vi "CRYO_MASTER_FULL_CHF2023.vi"() -> ()   [LabVIEW 2020]
uses:
  LSI218Data.lvclass
  LSI336Data.lvclass
  USBData.lvclass
  6240AData.lvclass
  DMMsData.lvclass
  LMData.lvclass
  <vilib>/DAQmx/miscellaneous.llb/DAQmx Fill In Error Info.vi
  <vilib>/DAQmx/create/channels.llb/DAQmx Create Channel (DO-Digital Output).vi
  <vilib>/DAQmx/create/channels.llb/DAQmx Create Channel (AO-Voltage-Basic).vi
  <vilib>/express/express arith-compare/Formula/XNode/ExpressFormulaBlockNode.xnode
  <vilib>/Analysis/NI_AALBase.lvlib
  istr.lib/Agilent 33XXX Series/Agilent 33XXX Series.lvlib
panel:
  out "Error Out (AZDAX status)":errorcluster
  in  "Automatic \nScreenshots?":bool=TRUE
  in  "Frontpanel screenshots":bool
  in  "Screenshots interval":i64=3605
  in  "Record interval":i64=1
  out "Cycle #":u32=1
  in  "Measurement Interval (s)":dbl=1.0
  in  "Stop Button":bool
  in  "?":T1(tab)=enum."CHF"
  out "RUN Identifier":string="20230719_105623_CHF2023"
  in  "Base Path (screenshots)":path=path "C:/LabVIEW/DATA/Google/TUCAN Experiments/KEK_cryotests_2019-2020/data/screenshots"
  out "error out (USB6210/6218 AOUT)":errorcluster
  in  "AOUT Labels":string[](array[string])=["PWR400H_I", "PMC183A_I"]
  in  "AOUT assignment":tag[](array[tag])=["Dev1/ao0", "Dev1/ao1"]
  out "AO task out":refnum<k21>="20230719_105623_CHF2023_AO"
  in  "Analog Out ON?":bool=TRUE
  in  "DOUT6218 Labels":string[](array[string])=["D_V1_NO", "D_V2_NC", "D_CV1", "D_H1", "D_HOME", "D_STOP", "D_M0", "D_M1"]
  in  "InstName (USB6218)":string="USB6218"
  in  "USB6218 Config":T2(array[cluster])=[{"Label"="P_yokogawa", "FileFormat"="%5.5e", "Active?"=TRUE, "Physical CH"="Dev1/ai0", " terminal\n type"=10106, "ConversionType"={"Type"=enum."SimpleProp", "ConversionParameters"=[1.0, 5.0, 0.0, 200000.0]}, "VoltageLimits"=[0.0, 5.0]}, {"Label"="P_Horiba", "FileFormat"="%5.5f", "Active?"=TRUE, "Physical CH"="Dev1/ai1", " terminal\n type"=10106, "ConversionType"={"Type"=enum."SimpleProp", "ConversionParameters"=[0.0, 10.0, 0.0, 13318.0]}, "VoltageLimits"=[0.0, 10.0]}, {"Label"="Level", "FileFormat"="%5.5f", "Active?"=TRUE, "Physical CH"="Dev1/ai2", " terminal\n type"=10106, "ConversionType"={"Type"=enum."SimpleProp", "ConversionParameters"=[0.0, 10.0, 0.0, 100.0]}, "VoltageLimits"=[0.0, 10.0]}, {"Label"="Kikusui_V_MON", "FileFormat"="%5.5f", "Active?"=TRUE, "Physical CH"="Dev1/ai3", " terminal\n type"=10106, "ConversionType"={"Type"=enum."SimpleProp", "ConversionParameters"=[0.0, 10.0, 0.0, 650.0]}, "VoltageLimits"=[0.0, 10.0]}, {"Label"="Kikusui_I_MON", "FileFormat"="%5.5f", "Active?"=TRUE, "Physical CH"="Dev1/ai4", " terminal\n type"=10106, "ConversionType"={"Type"=enum."SimpleProp", "ConversionParameters"=[0.0, 10.0, 0.0, 2000.0]}, "VoltageLimits"=[0.0, 10.0]}, {"Label"="H_V", "FileFormat"="%5.5f", "Active?"=TRUE, "Physical CH"="Dev1/ai5", " terminal\n type"=10106, "ConversionType"={"Type"=enum."SimpleProp", "ConversionParameters"=[0.0, 10.0, 0.0, 100.0]}, "VoltageLimits"=[0.0, 10.0]}] {"terminal\n type" items=["Default"=-1, "RSE"=10083, "NRSE"=10078, "Differential"=10106, "Pseudodifferential"=12529]}
  out "error out (USB6218)":errorcluster
  out "error out (USB6210/6218 DOUT)":errorcluster={"status"=TRUE, "code"=-200524, "source"="CRYO_MASTER_FULL_CHF2023.vi<append>\n<B>Number of Channels in Task: </B>8\n<B>Number of Channels in Data: </B>4\n\n<B>Task Name: </B>20230719_105623_CHF2023_DO"}
  out "DOUT task out":refnum<k21>="20230719_105623_CHF2023_DO"
  in  "DOUT Physical CH":tag[](array[tag])=["Dev1/port1/line0", "Dev1/port1/line1", "Dev1/port1/line2", "Dev1/port1/line3", "Dev1/port1/line4", "Dev1/port1/line5", "Dev1/port1/line6", "Dev1/port1/line7"]
  in  "Digital Out ON?":bool=TRUE
  in  "USB6210 Config":T2(array[cluster])=[{"Label"="P_ins", "FileFormat"="%5.5e", "Active?"=FALSE, "Physical CH"="Dev2/ai0", " terminal\n type"=10083, "ConversionType"={"Type"=enum."CC-10_LOG", "ConversionParameters"=[0.5, 9.0, 0.0, 1.0]}, "VoltageLimits"=[0.0, 10.0]}, {"Label"="P_4Kres", "FileFormat"="%5.5e", "Active?"=FALSE, "Physical CH"="Dev2/ai1", " terminal\n type"=10083, "ConversionType"={"Type"=enum."SimpleProp", "ConversionParameters"=[1.0, 5.0, 0.0, 200000.0]}, "VoltageLimits"=[0.0, 5.0]}, {"Label"="P_3HeIN", "FileFormat"="%5.5e", "Active?"=FALSE, "Physical CH"="Dev2/ai2", " terminal\n type"=10083, "ConversionType"={"Type"=enum."SimpleProp", "ConversionParameters"=[1.0, 5.0, 0.0, 200000.0]}, "VoltageLimits"=[0.0, 5.0]}, {"Label"="P_SldRTN", "FileFormat"="%5.5e", "Active?"=FALSE, "Physical CH"="Dev2/ai3", " terminal\n type"=10083, "ConversionType"={"Type"=enum."SimpleProp", "ConversionParameters"=[1.0, 5.0, 0.0, 200000.0]}, "VoltageLimits"=[0.0, 5.0]}, {"Label"="P_3Hepot", "FileFormat"="%5.5e", "Active?"=FALSE, "Physical CH"="Dev2/ai4", " terminal\n type"=10083, "ConversionType"={"Type"=enum."SimpleProp", "ConversionParameters"=[0.0, 10.0, 0.0, 133320.0]}, "VoltageLimits"=[0.0, 10.0]}, {"Label"="P_1Kpot", "FileFormat"="%5.5e", "Active?"=FALSE, "Physical CH"="Dev2/ai5", " terminal\n type"=10083, "ConversionType"={"Type"=enum."SimpleProp", "ConversionParameters"=[0.0, 10.0, 0.0, 133320.0]}, "VoltageLimits"=[0.0, 10.0]}, {"Label"="P_Dewar(old)", "FileFormat"="%5.5e", "Active?"=FALSE, "Physical CH"="Dev2/ai6", " terminal\n type"=10083, "ConversionType"={"Type"=enum."SimpleProp", "ConversionParameters"=[1.0, 5.0, 0.0, 200000.0]}, "VoltageLimits"=[0.0, 5.0]}, {"Label"="DP_HEX4", "FileFormat"="%5.5e", "Active?"=FALSE, "Physical CH"="Dev2/ai7", " terminal\n type"=10083, "ConversionType"={"Type"=enum."SimpleProp", "ConversionParameters"=[1.0, 5.0, 0.0, 1000.0]}, "VoltageLimits"=[0.0, 5.0]}, {"Label"="DP_HEX5", "FileFormat"="%5.5e", "Active?"=FALSE, "Physical CH"="Dev2/ai8", " terminal\n type"=10083, "ConversionType"={"Type"=enum."SimpleProp", "ConversionParameters"=[1.0, 5.0, 0.0, 1000.0]}, "VoltageLimits"=[0.0, 5.0]}, {"Label"="L1(old)", "FileFormat"="%5.5f", "Active?"=FALSE, "Physical CH"="Dev2/ai9", " terminal\n type"=10083, "ConversionType"={"Type"=enum."SimpleProp", "ConversionParameters"=[0.0, 10.0, 0.0, 100.0]}, "VoltageLimits"=[0.0, 10.0]}, {"Label"="L2-1", "FileFormat"="%5.5f", "Active?"=FALSE, "Physical CH"="Dev2/ai10", " terminal\n type"=10083, "ConversionType"={"Type"=enum."SimpleProp", "ConversionParameters"=[0.0, 10.0, 0.0, 100.0]}, "VoltageLimits"=[0.0, 10.0]}, {"Label"="L1", "FileFormat"="%5.5f", "Active?"=FALSE, "Physical CH"="Dev2/ai11", " terminal\n type"=10083, "ConversionType"={"Type"=enum."SimpleProp", "ConversionParameters"=[0.0, 10.0, 0.0, 100.0]}, "VoltageLimits"=[0.0, 10.0]}, {"Label"="L3", "FileFormat"="%5.5f", "Active?"=FALSE, "Physical CH"="Dev2/ai12", " terminal\n type"=10083, "ConversionType"={"Type"=enum."SimpleProp", "ConversionParameters"=[0.0, 10.0, 0.0, 100.0]}, "VoltageLimits"=[0.0, 10.0]}, {"Label"="P_HEX7OUT", "FileFormat"="%5.5e", "Active?"=FALSE, "Physical CH"="Dev2/ai13", " terminal\n type"=10083, "ConversionType"={"Type"=enum."SimpleProp", "ConversionParameters"=[1.0, 5.0, 0.0, 200000.0]}, "VoltageLimits"=[0.0, 5.0]}, {"Label"="P_IP", "FileFormat"="%5.5e", "Active?"=FALSE, "Physical CH"="Dev2/ai14", " terminal\n type"=10083, "ConversionType"={"Type"=enum."CC-10_LOG", "ConversionParameters"=[0.5, 9.0, 0.0, 1.0]}, "VoltageLimits"=[0.0, 10.0]}, {"Label"="V_H1", "FileFormat"="%3.5f", "Active?"=FALSE, "Physical CH"="Dev2/ai15", " terminal\n type"=10083, "ConversionType"={"Type"=enum."Raw", "ConversionParameters"=[0.0, 1.0, 0.0, 1.0]}, "VoltageLimits"=[0.0, 10.0]}] {"terminal\n type" items=["Default"=-1, "RSE"=10083, "NRSE"=10078, "Differential"=10106, "Pseudodifferential"=12529]}
  in  "RUN label":string="CHF2023"
  in  "Base Path":path=path "C:/LabVIEW/DATA/CHF2023"
  in  "InstName (USB6210)":string="USB6210"
  out "error out (USB6210)":errorcluster={"status"=TRUE, "code"=-200220, "source"="DAQmx Create Channel (AI-Voltage-Basic).vi:1780001<append>\n<B>Device Specified: </B>Dev2\n<B>Suggested Device(s): </B>Dev1\n\n<B>Task Name: </B>20230719_105623_CHF2023_USB6210__AIN"}
  out "File Refn USB AO":refnum<file>
  out "File Refn USB DO":refnum<file>
  out "File ref AZD-AX status":refnum<file>
  in  "LM measurement interval (>0)":i64=10
  in  "Active? (HP34401 LM)":bool
  in  "Labels (HP34401 LM)":string[](array[string])=["R_L2-2", "L2-2"]
  in  "FileFormat (HP34401 LM)":string[](array[string])=["%.4f", "%.4f"]
  in  "VISA (HP34401 LM)":refnum<visa-resource-name>="GPIB0::24::INSTR"
  in  "LevelCalibration (R0, R1, L0, L1)":dbl[](array[numeric])=[186.541, 0.0, 0.0, 100.0]
  in  "InstName (HP34401 LM)":string="HP34401LM"
  out "error out (LSI336)":errorcluster={"status"=TRUE, "code"=-1073807338, "source"="VISA Close in Lake Shore 336.lvlib:Close.vi->LSI336Data.lvclass:LSI336Data_terminate.vi->CRYO_MASTER_FULL_CHF2023.vi"}
  in  "InstName (LSI336)":string="LSI336"
  in  "FileFormat (336)":string="%4.4f"
  in  "LSI336Settings(X,Y)":T3(array[cluster])=[{"LSIName"="LSi336X", "Labels"=["T_Cu", "T_He", "N.C\n\n\n", "N.C"], "SensorLocations"=[enum."T1K3-1", enum."T1K3-2", enum."T3He5", enum."T3He8"], "Active?"=TRUE, "VISA res. name"="GPIB0::6::INSTR"}, {"LSIName"="LSi336Y", "Labels"=["T3He6-1", "T3He6-2", "T3He7-1", "T3He7-2"], "SensorLocations"=[enum."T3He6-1", enum."T3He6-2", enum."T3He7-1", enum."T3He7-2"], "Active?"=FALSE, "VISA res. name"="COM20_LSI336X"}]
  in  "FileFormat (218)":string="%4.4f"
  in  "InstName (LSI218)":string="LSI218"
  in  "LSI218Settings(A-F)":T3(array[cluster])=[{"LSIName"="LSI218A", "Labels"=["T3He10", "T3He1-1", "TTH3", "TTH4", "TTH1", "TTH2", "T4He1", "T1K1"], "SensorLocations"=[enum."T3He10", enum."T3He1-1", enum."TTH3", enum."TTH4", enum."TTH1", enum."TTH2", enum."T4He1", enum."T1K1"], "Active?"=FALSE, "VISA res. name"="GPIB0::7::INSTR"}, {"LSIName"="LSI218B", "Labels"=["N.C.", "N.C.", "N.C.", "N.C.", "T3He2-1", "T3He2-2", "T3He3", "T3He1-4"], "SensorLocations"=[enum."N.C.", enum."N.C.", enum."N.C.", enum."N.C.", enum."T3He2-1", enum."T3He2-2", enum."T3He3", enum."T3He1-4"], "Active?"=FALSE, "VISA res. name"="GPIB0::4::INSTR"}, {"LSIName"="LSI218C", "Labels"=["T4He3-1", "T4He3-2", "T4He3-3", "T4He3-4", "T4He2-1", "T4He2-2", "T4He4", "T4He5"], "SensorLocations"=[enum."T4He3-1", enum."T4He3-2", enum."T4He3-3", enum."T4He3-4", enum."T4He2-1", enum."T4He2-2", enum."T4He4", enum."T4He5"], "Active?"=FALSE, "VISA res. name"="GPIB0::3::INSTR"}, {"LSIName"="LSI218D", "Labels"=["T4He6", "T4He9", "T3He1-2", "T3He1-3", "T4He7", "T4He8", "T4He10", "T1K6"], "SensorLocations"=[enum."T4He6", enum."T4He9", enum."T3He1-2", enum."T3He1-3", enum."T4He7", enum."T4He8", enum."T4He10", enum."T1K6"], "Active?"=FALSE, "VISA res. name"="GPIB0::5::INSTR"}, {"LSIName"="LSI218E", "Labels"=["TIP1", "N.C.", "TIP2", "N.C.", "TIP3", "TIP4", "TIP5", "N.C."], "SensorLocations"=[enum."TIP1", enum."N.C.", enum."TIP2", enum."N.C.", enum."TIP3", enum."TIP4", enum."TIP5", enum."N.C."], "Active?"=FALSE, "VISA res. name"="GPIB0::11::INSTR"}, {"LSIName"="LSI218F", "Labels"=["T1K2", "T1K4", "T1K5", "T3He4", "T3He9", "TIP6", "N.C.", "N.C."], "SensorLocations"=[enum."T1K2", enum."T1K4", enum."T1K5", enum."T3He4", enum."T3He9", enum."TIP6", enum."N.C.", enum."N.C."], "Active?"=FALSE, "VISA res. name"="GPIB0::8::INSTR"}]
  out "error out (LSI218)":errorcluster
  out "RUN Identifier 2":string="20230719_105623_CHF2023" caption="RUN Identifier"
  out "error out (HP34401 LM)":errorcluster
  out "Graph 3":T4(graph)=[{"TimeArray"=[timestamp(3772576585.022536 s since 1904-01-01)], "DataArray"=[0.018423510306911722]}] caption="XY Graph"
  out "Graph 1":T4(graph)=[{"TimeArray"=[timestamp(3772576585.022536 s since 1904-01-01)], "DataArray"=[298.66]}, {"TimeArray"=[timestamp(3772576585.022536 s since 1904-01-01)], "DataArray"=[298.457]}] caption="XY Graph"
  in  "FIle suffix 4":string="Graph4_noise"
  in  "Take Screenshot! 4":bool
  in  "Take Screenshot! 3":bool
  in  "Take Screenshot! 2":bool
  in  "Take Screenshot! 1":bool
  in  "FIle suffix 3":string="Graph3_noise"
  in  "FIle suffix 2":string="Graph2_build"
  in  "FIle suffix 1":string="Graph1_noise"
  in  "log/linear 2":bool
  in  "Tab Control 2":T5(tab)=enum."Temperature (3)"
  in  "Plot selecter (USB6210)\n    1      2     3     4":bool[][](array[boolean])=[[FALSE, FALSE, FALSE, FALSE], [TRUE, FALSE, FALSE, FALSE], [TRUE, FALSE, FALSE, FALSE], [TRUE, FALSE, FALSE, FALSE], [TRUE, FALSE, FALSE, FALSE], [TRUE, FALSE, FALSE, FALSE], [TRUE, FALSE, FALSE, FALSE], [FALSE, FALSE, FALSE, FALSE], [FALSE, FALSE, FALSE, FALSE], [FALSE, TRUE, FALSE, FALSE], [FALSE, TRUE, FALSE, FALSE], [FALSE, TRUE, FALSE, FALSE], [FALSE, TRUE, FALSE, FALSE], [TRUE, FALSE, FALSE, FALSE], [TRUE, FALSE, FALSE, FALSE], [FALSE, FALSE, FALSE, FALSE]]
  out "All Labels (USB6210)":string[](array[string])
  out "Last Data \n(USB6210)":dbl[](array[numeric]) format="%#_6e"
  out "Time of Last Measurement (USB6210)":timestamp
  out "USB6210 Status":T6(ring)=enum."Ready"
  out "Last Vol\n(USB6210)":dbl[](array[numeric]) format="%_5f"
  out "Labels (HP34401 LM) 2":string[](array[string])=["R_L2-2", "L2-2"]
  out "LastData (HP34401 LM)":dbl[](array[numeric])
  in  "Plot selecter (HP34401A)\n    1      2     3     4":bool[][](array[boolean])=[[FALSE, TRUE, FALSE, FALSE], [FALSE, TRUE, FALSE, FALSE], [TRUE, FALSE, FALSE, FALSE], [TRUE, FALSE, FALSE, FALSE], [TRUE, FALSE, FALSE, FALSE], [TRUE, FALSE, FALSE, FALSE], [TRUE, FALSE, FALSE, FALSE], [FALSE, TRUE, FALSE, FALSE], [FALSE, TRUE, FALSE, FALSE], [FALSE, TRUE, FALSE, FALSE], [FALSE, TRUE, FALSE, FALSE], [FALSE, TRUE, FALSE, FALSE], [FALSE, TRUE, FALSE, FALSE], [TRUE, FALSE, FALSE, FALSE], [TRUE, FALSE, FALSE, FALSE], [FALSE, FALSE, FALSE, FALSE]]
  out "Time of Last Measurement (USB6218)":timestamp=timestamp(3772576585.022536 s since 1904-01-01)
  out "USB6218 Status":T6(ring)=enum."Ready"
  out "Last Vol \n(USB6218)":dbl[](array[numeric])=[3.002313120260557, 10.743101988532857, 0.0018423510306911721, -0.29656235341614134, 0.1802800774598221, 0.002105436509847161] format="%_5f"
  out "Last Data \n(USB6218)":dbl[](array[numeric])=[100115.65601302785, 14307.663228328058, 0.018423510306911722, -19.27655297204919, 36.05601549196442, 0.02105436509847161] format="%#_6e"
  out "All Labels (USB6218)":string[](array[string])=["P_yokogawa", "P_Horiba", "Level", "Kikusui_V_MON", "Kikusui_I_MON", "H_V"]
  in  "Plot selecter (USB6218)\n    1      2     3     4":bool[][](array[boolean])=[[FALSE, TRUE, FALSE, FALSE], [FALSE, TRUE, FALSE, FALSE], [FALSE, FALSE, TRUE, FALSE], [FALSE, FALSE, FALSE, TRUE], [FALSE, FALSE, FALSE, TRUE], [FALSE, FALSE, FALSE, TRUE], [FALSE, FALSE, FALSE, FALSE], [FALSE, FALSE, FALSE, FALSE], [FALSE, TRUE, FALSE, FALSE], [FALSE, FALSE, FALSE, TRUE], [FALSE, FALSE, FALSE, TRUE], [FALSE, FALSE, FALSE, TRUE], [FALSE, FALSE, FALSE, TRUE], [FALSE, FALSE, FALSE, FALSE], [FALSE, FALSE, FALSE, FALSE], [FALSE, FALSE, FALSE, FALSE]]
  out "Time of Last Measurement (LSI218)":timestamp=timestamp(3772576585.022536 s since 1904-01-01)
  out "LSI218 Status":T7(ring)=enum."Measuring"
  out "Last Data \nLSI218 (1)":dbl[](array[numeric])
  out "Labels LSI218 (1)":string[](array[string])=["T3He10", "T3He1-1", "TTH3", "TTH4", "TTH1", "TTH2", "T4He1", "T1K1", "N.C.", "N.C.", "N.C.", "N.C.", "T3He2-1", "T3He2-2", "T3He3", "T3He1-4", "T4He3-1", "T4He3-2", "T4He3-3", "T4He3-4", "T4He2-1", "T4He2-2", "T4He4", "T4He5"]
  in  "Plot selecter LSI218(1)\n    1      2     3     4":bool[][](array[boolean])=[[FALSE, FALSE, FALSE, FALSE], [FALSE, FALSE, FALSE, FALSE], [FALSE, FALSE, FALSE, FALSE], [FALSE, FALSE, FALSE, FALSE], [FALSE, FALSE, FALSE, FALSE], [FALSE, FALSE, FALSE, FALSE], [FALSE, FALSE, FALSE, FALSE], [FALSE, FALSE, FALSE, FALSE], [FALSE, FALSE, FALSE, FALSE], [FALSE, FALSE, FALSE, FALSE], [FALSE, FALSE, FALSE, FALSE], [FALSE, FALSE, FALSE, FALSE], [FALSE, FALSE, FALSE, FALSE], [FALSE, FALSE, FALSE, FALSE], [FALSE, FALSE, FALSE, FALSE], [FALSE, FALSE, FALSE, FALSE], [FALSE, FALSE, FALSE, FALSE], [FALSE, FALSE, FALSE, FALSE], [FALSE, FALSE, FALSE, FALSE], [FALSE, FALSE, FALSE, FALSE], [FALSE, FALSE, FALSE, FALSE], [FALSE, FALSE, FALSE, FALSE], [FALSE, FALSE, FALSE, FALSE], [FALSE, FALSE, FALSE, FALSE]]
  out "Active?\n (1)":bool[](array[boolean])
  out "Labels LSI218 (2)":string[](array[string])=["T4He6", "T4He9", "T3He1-2", "T3He1-3", "T4He7", "T4He8", "T4He10", "T1K6", "TIP1", "N.C.", "TIP2", "N.C.", "TIP3", "TIP4", "TIP5", "N.C.", "T1K2", "T1K4", "T1K5", "T3He4", "T3He9", "TIP6", "N.C.", "N.C."]
  out "Active?\n(2)":bool[](array[boolean])
  out "Last Data \nLSI218 (2)":dbl[](array[numeric])
  in  "Plot selecter LSI218(2)\n    1      2     3     4":bool[][](array[boolean])=[[FALSE, FALSE, FALSE, FALSE], [FALSE, FALSE, FALSE, FALSE], [FALSE, FALSE, FALSE, FALSE], [FALSE, FALSE, FALSE, FALSE], [FALSE, FALSE, FALSE, FALSE], [FALSE, FALSE, FALSE, FALSE], [FALSE, FALSE, FALSE, FALSE], [FALSE, FALSE, FALSE, FALSE], [FALSE, FALSE, FALSE, FALSE], [FALSE, FALSE, FALSE, FALSE], [FALSE, FALSE, FALSE, FALSE], [FALSE, FALSE, FALSE, FALSE], [FALSE, FALSE, FALSE, FALSE], [FALSE, FALSE, FALSE, FALSE], [FALSE, FALSE, FALSE, FALSE], [FALSE, FALSE, FALSE, FALSE], [FALSE, FALSE, FALSE, FALSE], [FALSE, FALSE, FALSE, FALSE], [FALSE, FALSE, FALSE, FALSE], [FALSE, FALSE, FALSE, FALSE], [FALSE, FALSE, FALSE, FALSE], [FALSE, FALSE, FALSE, FALSE], [FALSE, FALSE, FALSE, FALSE], [FALSE, FALSE, FALSE, FALSE]]
  in  "Plot selecter LSI336 \n     1      2     3     4":bool[][](array[boolean])=[[TRUE, FALSE, FALSE, FALSE], [TRUE, FALSE, FALSE, FALSE], [FALSE, FALSE, FALSE, FALSE], [FALSE, FALSE, FALSE, FALSE], [FALSE, FALSE, FALSE, FALSE], [FALSE, FALSE, FALSE, FALSE], [FALSE, FALSE, FALSE, FALSE], [FALSE, FALSE, FALSE, FALSE]]
  out "Time of Last Measurement (LSI336)":timestamp=timestamp(3772576585.022536 s since 1904-01-01)
  out "Last Data \nLSI336":dbl[](array[numeric])=[298.66, 298.457, 0.0, 0.0, 0.0, 0.0, 0.0, 0.0, 0.0, 0.0, 0.0, 0.0]
  out "Active?\n(LSI336)":bool[](array[boolean])=[TRUE, TRUE, TRUE, TRUE, FALSE, FALSE, FALSE, FALSE]
  out "Labels LSI336":string[](array[string])=["T_Cu", "T_He", "N.C\n\n\n", "N.C", "T3He6-1", "T3He6-2", "T3He7-1", "T3He7-2"]
  out "LSI336 Status":T7(ring)=enum."Measuring"
  in  "log/linear 1":bool
  out "Graph 2":T4(graph)=[{"TimeArray"=[timestamp(3772576585.022536 s since 1904-01-01)], "DataArray"=[100115.65601302785]}, {"TimeArray"=[timestamp(3772576585.022536 s since 1904-01-01)], "DataArray"=[14307.663228328058]}, {"TimeArray"=[], "DataArray"=[]}, {"TimeArray"=[], "DataArray"=[]}] caption="XY Graph"
  out "Graph 4":T4(graph)=[{"TimeArray"=[timestamp(3772576585.022536 s since 1904-01-01)], "DataArray"=[-19.27655297204919]}, {"TimeArray"=[timestamp(3772576585.022536 s since 1904-01-01)], "DataArray"=[36.05601549196442]}, {"TimeArray"=[timestamp(3772576585.022536 s since 1904-01-01)], "DataArray"=[0.02105436509847161]}] caption="XY Graph"
  in  "log/linear 4":bool
  in  "log/linear 3":bool
  out "RUN Identifier 3":string="20230719_105623_CHF2023" caption="RUN Identifier"
  in  "AutoFill Source (P)":T8(ring)=enum."USB6218AI"
  in  "AutoFill Source (L)":T8(ring)
  out "RUN Identifier 4":string="20230719_105623_CHF2023" caption="RUN Identifier"
  out "Fill (false)":bool=TRUE
  in  "Fill state":bool
  out "state 1 (false)":bool=TRUE
  out "state 1":bool
  out "state 2":bool
  out "state 2 (false)":bool=TRUE
  out "Status V2 CTRL":enum16{"Pressurize", "Release"}(ring)=enum."Release"
  out "Status V1 CTRL":enum16{"Pressurize", "Release"}(ring)
  out "Lav (%)":dbl=nan format="%0.2f"
  out "Lstd":dbl=-0.0 format="%0.2f"
  out "Last N M.A. Levels":dbl[](array[numeric]) format="%_5e"
  out "Lstd history":dbl(graph)=-0.0
  out "Lav history":dbl(graph)=nan
  out "Target Index (L)":i32=-1
  in  "Auto Fll He L. label":string="L3"
  out "Target Index (P)":i32=-1
  in  "Auto Fll Dewar P. label":string="P_Dewar"
  out "He Level":T9(graph) caption="XY Graph"
  in  "P_safelimit_high (Pa)":dbl=300000.0 format="%_4e"
  in  "P_safelimit_low (Pa)":dbl=100.0 format="%_4e"
  in  "Auto Fill ON?":bool=TRUE
  out "Pstd history":dbl(graph)
  out "Pav history":dbl(graph)
  in  "Mov. Avg Interval":i64=4
  in  "V2 (N.C.)":bool
  in  "V1 (N.O.)":bool=TRUE
  in  "N for sampling":i64=7
  in  "L_low (%)":dbl=100.0 format="%_3f"
  in  "L_high (%)":dbl=100.0 format="%_3g"
  in  "P_2_low (Pa)":dbl=125000.0 format="%_4e"
  in  "P_1_low (Pa)":dbl=130000.0 format="%_4g"
  in  "P_2_high (Pa)":dbl=130000.0 format="%_4e"
  in  "P_1_high (Pa)":dbl=140000.0 format="%_4e"
  out "Dewar Pressure":T9(graph) caption="XY Graph"
  out "Last N M.A. Pressures":dbl[](array[numeric]) format="%_5e"
  out "Pav (Pa)":dbl format="%0.4e"
  out "Pstd":dbl format="%0.4e"
  out "File Refn DewarCTRL":refnum<file>
  out "Error Out (Dewar CTRL":errorcluster
  out "... more steps":u64
  in  "Current position":dbl format="%_4f"
  out "AZD-AZ status":string
  out "Opening rate (Closed:0, Full open:100)":dbl(knob)=8.822438978731505 scale=0.0..100.0
  in  "DOUT Raw state":bool[](array[boolean])=[FALSE, FALSE, FALSE, FALSE, FALSE, FALSE, FALSE, FALSE]
  out "DOUT Labels 2":string[](array[string])=["D_V1_NO", "D_V2_NC", "D_CV1", "D_H1", "D_HOME", "D_STOP", "D_M0", "D_M1"]
  in  "DOUT (PMC)":string="D_H1"
  in  "DOUT (PWR)":string="D_CV1"
  in  "lower limit (mA) \n(PMC)":dbl=4.0 format="%_3f"
  in  "upper limit (mA)\n (PMC)":dbl=40.0 format="%_3f"
  in  "OUTPUT\n(PMC)":bool
  in  "Set Current (mA)\n (PMC)":dbl=4.0 min=4.0 max=40.0 format="%_3g"
  in  "update values":bool
  out "USB 6218 AOUT":dbl[](array[numeric])=[0.0, 0.004, 0.049823637537880675, 0.06969546425555169]
  out "Graph 7":T10(graph) caption="XY Graph"
  in  "lower limit (mA)":dbl=4.0 format="%_3f"
  in  "SetCurrent 2 (mA)":dbl=4.0 min=4.0 max=500.0 format="%_3f"
  in  "upper limit (mA)":dbl=500.0 format="%_3f"
  out "error out (KIKUSI CTRL)":errorcluster
  out "ActualVoltage (V)":dbl[](array[numeric]) format="%_6g"
  out "ActualCurrent (A)":dbl[](array[numeric])=[0.004, 0.004] format="%_3e"
  in  "SetCurrent 1 (mA)":dbl=4.0 min=4.0 max=500.0 format="%_3g"
  in  "Output\n (ADCMT)":bool[](array[boolean])=[FALSE, FALSE]
  out "error out (ADCMT6420A)":errorcluster
  out "Monitor Current (mA)":dbl=0.4 min=0.0 max=1.9 format="%_4e"
  in  "update current":bool
  in  "lower limit (mA) \n(PWR)":dbl=4.0 format="%_3f"
  in  "upper limit (mA)\n (PWR)":dbl format="%_3f"
  in  "CONTROL KIKUSUI?":bool=TRUE
  in  "OUTPUT\n(PWR)":bool
  in  "Set Current (mA)\n (PWR)":dbl min=4.0 max=4.0 format="%_3g"
  in  "Voltage limits (V)":dbl[](array[numeric])=[12.0, 12.0] format="%_3f"
  in  "CtrlLabels":string[](array[string])=["CV2", "CV3"]
  in  "VISA":refnum<visa-resource-name>[](array[refnum])=["GPIB0::1::INSTR", "GPIB0::12::INSTR"]
  out "Initialized?":bool
  in  "InstName":string="ADCMT6240"
  out "Graph 6":T9(graph)=[{"TimeArray"=[timestamp(3695085214.3168983 s since 1904-01-01), timestamp(3695085244.964852 s since 1904-01-01), timestamp(3695085246.0168433 s since 1904-01-01), timestamp(3695085588.0010176 s since 1904-01-01)], "Filtered X"=[0.001, 0.005, 0.005, 0.01]}, {"TimeArray"=[timestamp(3695085214.3168983 s since 1904-01-01), timestamp(3695085244.964852 s since 1904-01-01), timestamp(3695085246.0168433 s since 1904-01-01), timestamp(3695085588.0010176 s since 1904-01-01)], "Filtered X"=[0.004, 0.004, 0.004, 0.004]}, {"TimeArray"=[timestamp(3695085214.3168983 s since 1904-01-01), timestamp(3695085244.964852 s since 1904-01-01), timestamp(3695085246.0168433 s since 1904-01-01), timestamp(3695085588.0010176 s since 1904-01-01)], "Filtered X"=[0.001, 0.005, 0.005, 0.01]}, {"TimeArray"=[timestamp(3695085214.3168983 s since 1904-01-01), timestamp(3695085244.964852 s since 1904-01-01), timestamp(3695085246.0168433 s since 1904-01-01), timestamp(3695085588.0010176 s since 1904-01-01)], "Filtered X"=[0.004, 0.004, 0.004, 0.004]}] caption="XY Graph"
  in  "Initialize":bool
  out "RUN Identifier 5":string="20230719_105623_CHF2023" caption="RUN Identifier"
  in  "Tab Control 3":enum32{"Basic control", "Advanced control"}(tab)=enum."Advanced control"
  in  "wait for home (s)":dbl=50.0
  in  "wait for open/close/stop (s)":dbl=2.0
  in  "AZD-AZ open":string="D_M0"
  in  "AZD-AZ close":string="D_M1"
  in  "AZD-AZ home":string="D_HOME"
  in  "AZD-AZ stop":string="D_STOP"
  in  "Motor stop":bool
  in  "Open 1/4":bool
  in  "Close 1/4":bool
  in  "Motor home":bool
  in  "N to close":u64=1
  in  "N to open":u64=1
  in  "Open N":bool
  in  "Close N":bool
  out "Close Command accepted":bool
  out "Open Command accepted":bool
  in  "DMMsConfig":T11(array[cluster])=[{"Label"="I_H", "Active?"=TRUE, "VISA resource name"="GPIB0::24::INSTR", "Device"=enum."Agilent34401A", "Measurement"=enum."DC Currents", "FileFormat"="%.4e"}, {"Label"="V_H", "Active?"=TRUE, "VISA resource name"="GPIB0::22::INSTR", "Device"=enum."Agilent34401A", "Measurement"=enum."DC Volts", "FileFormat"="%.4e"}, {"Label"="P_yokogawa_DMM", "Active?"=FALSE, "VISA resource name"="GPIB0::23::INSTR", "Device"=enum."ADCMT7451", "Measurement"=enum."DC Volts", "FileFormat"="%.4e"}]
  out "ƒ¢T=T_2 -T_1":dbl
  out "Graph DMMs 3":T4(graph)=[{"TimeArray"=[timestamp(3772576585.60657 s since 1904-01-01)], "DataArray"=[1.6400000000000001e-09]}, {"TimeArray"=[timestamp(3772576585.60657 s since 1904-01-01)], "DataArray"=[-8.08998e-05]}, {"TimeArray"=[timestamp(3772576585.60657 s since 1904-01-01)], "DataArray"=[0.0]}, {"TimeArray"=[timestamp(3772576585.60657 s since 1904-01-01)], "DataArray"=[0.0]}, {"TimeArray"=[timestamp(3772576585.60657 s since 1904-01-01)], "DataArray"=[0.0]}, {"TimeArray"=[timestamp(3772576585.60657 s since 1904-01-01)], "DataArray"=[0.0]}, {"TimeArray"=[timestamp(3772576585.60657 s since 1904-01-01)], "DataArray"=[0.0]}, {"TimeArray"=[timestamp(3772576585.60657 s since 1904-01-01)], "DataArray"=[0.0]}, {"TimeArray"=[timestamp(3772576585.60657 s since 1904-01-01)], "DataArray"=[0.0]}, {"TimeArray"=[timestamp(3772576585.60657 s since 1904-01-01)], "DataArray"=[0.0]}, {"TimeArray"=[timestamp(3772576585.60657 s since 1904-01-01)], "DataArray"=[0.0]}, {"TimeArray"=[timestamp(3772576585.60657 s since 1904-01-01)], "DataArray"=[0.0]}] caption="XY Graph"
  out "Q = I *V":dbl=-1.3267567200000002e-13
  in  "index I":i64
  in  "index V":i64=1
  out "VariableSources":T12(array[ring])=[enum."USB6210", enum."USB6218AI", enum."USB6218AI", enum."USB6218AI", enum."USB6210", enum."LSI336", enum."LSI336", enum."LSI336", enum."LSI336"]
  in  "DMMsConfig (variables)":T13(array[cluster])=[{"Label"="P_3Hepot", "Active?"=FALSE, "Source"=enum."USB6210", "SourceLabel"="P_3Hepot", "FileFormat"="%6.4e"}, {"Label"="F_1", "Active?"=FALSE, "Source"=enum."USB6218AI", "SourceLabel"="F_1", "FileFormat"="%3.4f"}, {"Label"="F_4", "Active?"=FALSE, "Source"=enum."USB6218AI", "SourceLabel"="F_4", "FileFormat"="%3.4f"}, {"Label"="F_5", "Active?"=FALSE, "Source"=enum."USB6218AI", "SourceLabel"="F_5", "FileFormat"="%3.4f"}, {"Label"="DP_HEX4", "Active?"=FALSE, "Source"=enum."USB6210", "SourceLabel"="DP_HEX4", "FileFormat"="%4.3e"}, {"Label"="T3He6-1", "Active?"=FALSE, "Source"=enum."LSI336", "SourceLabel"="T3He6-1", "FileFormat"="%3.4f"}, {"Label"="T3He6-2", "Active?"=FALSE, "Source"=enum."LSI336", "SourceLabel"="T3He6-2", "FileFormat"="%3.4f"}, {"Label"="T3He7-1", "Active?"=FALSE, "Source"=enum."LSI336", "SourceLabel"="T3He7-1", "FileFormat"="%3.4f"}, {"Label"="T3He7-2", "Active?"=FALSE, "Source"=enum."LSI336", "SourceLabel"="T3He7-2", "FileFormat"="%3.4f"}]
  in  "Measure DMMs?":bool=TRUE
  out "DMMsLabels":string[](array[string])=["I_H", "V_H", "P_yokogawa_DMM", "P_3Hepot", "F_1", "F_4", "F_5", "DP_HEX4", "T3He6-1", "T3He6-2", "T3He7-1", "T3He7-2"]
  out "Active?":bool[](array[boolean])=[TRUE, TRUE, FALSE, FALSE, FALSE, FALSE, FALSE, FALSE, FALSE, FALSE, FALSE, FALSE]
  out "DMM LastMeasurements":dbl[](array[numeric])=[1.6400000000000001e-09, -8.08998e-05, 0.0, 0.0, 0.0, 0.0, 0.0, 0.0, 0.0, 0.0, 0.0, 0.0]
  out "Graph DMMs 2":T4(graph)=[{"TimeArray"=[timestamp(3772576585.60657 s since 1904-01-01)], "DataArray"=[1.6400000000000001e-09]}, {"TimeArray"=[timestamp(3772576585.60657 s since 1904-01-01)], "DataArray"=[-8.08998e-05]}, {"TimeArray"=[timestamp(3772576585.60657 s since 1904-01-01)], "DataArray"=[0.0]}, {"TimeArray"=[timestamp(3772576585.60657 s since 1904-01-01)], "DataArray"=[0.0]}, {"TimeArray"=[timestamp(3772576585.60657 s since 1904-01-01)], "DataArray"=[0.0]}, {"TimeArray"=[timestamp(3772576585.60657 s since 1904-01-01)], "DataArray"=[0.0]}, {"TimeArray"=[timestamp(3772576585.60657 s since 1904-01-01)], "DataArray"=[0.0]}, {"TimeArray"=[timestamp(3772576585.60657 s since 1904-01-01)], "DataArray"=[0.0]}, {"TimeArray"=[timestamp(3772576585.60657 s since 1904-01-01)], "DataArray"=[0.0]}, {"TimeArray"=[timestamp(3772576585.60657 s since 1904-01-01)], "DataArray"=[0.0]}, {"TimeArray"=[timestamp(3772576585.60657 s since 1904-01-01)], "DataArray"=[0.0]}, {"TimeArray"=[timestamp(3772576585.60657 s since 1904-01-01)], "DataArray"=[0.0]}] caption="XY Graph"
  out "DMMFileName":string="20230719_105623_CHF2023_DMMs_20230719_105623.csv"
  out "error out (DMMs)":errorcluster
  out "cycle # (DMMs)":i32=1
  in  "Measurement Interval DMMs (ms)":i64=500
  in  "InstName DMMs":string="DMMs"
  in  "Initialize (DMMs)":bool
  out "Graph DMMs 1":T4(graph)=[{"TimeArray"=[timestamp(3772576585.60657 s since 1904-01-01)], "DataArray"=[1.6400000000000001e-09]}, {"TimeArray"=[timestamp(3772576585.60657 s since 1904-01-01)], "DataArray"=[-8.08998e-05]}, {"TimeArray"=[timestamp(3772576585.60657 s since 1904-01-01)], "DataArray"=[0.0]}, {"TimeArray"=[timestamp(3772576585.60657 s since 1904-01-01)], "DataArray"=[0.0]}, {"TimeArray"=[timestamp(3772576585.60657 s since 1904-01-01)], "DataArray"=[0.0]}, {"TimeArray"=[timestamp(3772576585.60657 s since 1904-01-01)], "DataArray"=[0.0]}, {"TimeArray"=[timestamp(3772576585.60657 s since 1904-01-01)], "DataArray"=[0.0]}, {"TimeArray"=[timestamp(3772576585.60657 s since 1904-01-01)], "DataArray"=[0.0]}, {"TimeArray"=[timestamp(3772576585.60657 s since 1904-01-01)], "DataArray"=[0.0]}, {"TimeArray"=[timestamp(3772576585.60657 s since 1904-01-01)], "DataArray"=[0.0]}, {"TimeArray"=[timestamp(3772576585.60657 s since 1904-01-01)], "DataArray"=[0.0]}, {"TimeArray"=[timestamp(3772576585.60657 s since 1904-01-01)], "DataArray"=[0.0]}] caption="XY Graph"
  out "error out (DMM graphs)":errorcluster
  in  "Sample #":i32=5
  in  "index T_ 1":i64=6
  in  "index T_2":i64=9
  out "error out (DMMs) 2":errorcluster
  out "P_HEX7OUT":dbl format="%_4e"
  out "P (HEX7 out)":dbl format="%_4e"
  out "DP HEX5":dbl format="%_4e"
  out "DP_HEX5":dbl format="%_4e"
  in  "Diff pressure HEX5":string="DP_HEX5"
  out "3He pot level":dbl format="%_4f"
  in  "3He pot":string="L1"
  out "He level (3He)":dbl(slide) scale=0.0..100.0
  out "He level (1K) b":dbl(slide) scale=0.0..100.0
  out "He level (1K)":dbl(slide) scale=0.0..100.0
  out "He level (4K)":dbl(slide) scale=0.0..100.0
  out "1K pot(b1)":dbl format="%_4f"
  in  "1K pot (b)":string="L2-2"
  in  "1K pot level":string="L2-1"
  out "L(1K) (a1)":dbl format="%_4f"
  in  "SensorLocation 2":T14(ring)=enum."T3He5"
  out "Temperature 2":dbl
  out "DP HEX4":dbl format="%_4e"
  in  "Diff pressure HEX4":string="DP_HEX4"
  out "V2":bool
  out "V1":bool=TRUE
  out "F5 (1K pump ex.)":dbl format="%_4f"
  out "F4 (3He in to HEX7)":dbl format="%_3f"
  out "F3 (4He rtn flw via HEX7)":dbl format="%_4f"
  out "F1 (3He pump exhaust) flow":dbl format="%_4f"
  out "P (Dewar)":dbl format="%_4e"
  out "P (1K pot)":dbl format="%_4e"
  out "P (3He pot)":dbl format="%_4e"
  out "P (shield return)":dbl format="%_4e"
  out "P (3He IN)":dbl format="%_4e"
  out "P (4K reservoir)":dbl format="%_4e"
  out "P (insulation)":dbl format="%_4e"
  in  "1Kpot pump exhaust flow":string="F_5"
  out "F_5":dbl format="%_4f"
  in  "3He incoming flow into HEX7":string="F_4"
  out "F_4":dbl format="%_4f"
  out "F_3":dbl format="%_4f"
  in  "4He return flow from HEX7":string="F_3"
  out "F_2":dbl format="%_4f"
  in  "Shield flow":string="F_2"
  out "P_SldRTN":dbl format="%_4e"
  in  "3He pot pressure":string="P_3Hepot"
  out "P_3Hepot":dbl format="%_4e"
  in  "Shield return press.":string="P_SldRTN"
  out "F_1":dbl format="%_4f"
  in  "3He pump exhaust flow":string="F_1"
  out "P_Dewar":dbl format="%_4e"
  in  "Dewar pressure":string="P_Dewar"
  out "P_1Kpot":dbl format="%_4e"
  in  "1Kpot pressure":string="P_1Kpot"
  out "P_3HeIN":dbl format="%_4e"
  in  "3He inlet pressure":string="P_3HeIN"
  in  "4K reservoir pressure":string="P_4Kres"
  out "P_4Kres":dbl format="%_4e"
  out "P_ins":dbl format="%_4e"
  in  "Insulation vacuum":string="P_ins"
  out "T3He7-1/6-2 (3He pot) 2":dbl format="%_4f"
  out "T3He7-1/7-2 (HEX1)":dbl format="%_4f"
  out "T3He6-1/6-2 (3He pot) 2":dbl format="%_4f"
  out "T3He6-1/6-2 (HEX1)":dbl format="%_4f"
  out "T1K3-1/3-2 (1K pot) 2":dbl=9.0036 format="%_4f"
  out "T1K3-1/3-2 (1K pot)":dbl=2.1697 format="%_4f"
  out "T4He1 (4K reservoir )":dbl format="%_4f"
  out "Temperature 1":dbl
  in  "SensorLocation 1":T14(ring)=enum."TTH2"
  out "TIP7":dbl format="%_4g"
  out "T3He6-2":dbl format="%_4g"
  out "T3He7-2":dbl format="%_4g"
  out "T3He6-1":dbl format="%_4g"
  out "T3He4":dbl format="%_4g"
  out "T3He7-1":dbl format="%_4g"
  out "T3He8":dbl format="%_4g"
  out "T3He5":dbl format="%_4g"
  out "T1K3-2":dbl=9.0036 format="%_4g"
  out "T1K3-1":dbl=2.1697 format="%_4g"
  out "TIP6":dbl format="%_4g"
  out "T3He9":dbl format="%_4g"
  out "T1K5":dbl format="%_4g"
  out "T1K4":dbl format="%_4g"
  out "T1K2":dbl format="%_4g"
  out "TIP5":dbl format="%_4g"
  out "TIP4":dbl format="%_4g"
  out "TIP3":dbl format="%_4g"
  out "TIP2":dbl format="%_4g"
  out "TIP1":dbl format="%_4g"
  out "T1K6":dbl format="%_4g"
  out "T4He10":dbl format="%_4g"
  out "T4He8":dbl format="%_4g"
  out "T4He7":dbl format="%_4g"
  out "T3He1-3":dbl format="%_4g"
  out "T3He1-2":dbl format="%_4g"
  out "T4He9":dbl format="%_4g"
  out "T4He6":dbl format="%_4g"
  out "T4He5":dbl format="%_4g"
  out "T4He4":dbl format="%_4g"
  out "T4He2-2":dbl format="%_4g"
  out "T4He2-1":dbl format="%_4g"
  out "T4He3-4":dbl format="%_4g"
  out "T4He3-3":dbl format="%_4g"
  out "T4He3-2":dbl format="%_4g"
  out "T4He3-1":dbl format="%_4g"
  out "T3He1-4":dbl format="%_4g"
  out "T3He3":dbl format="%_4g"
  out "T3He2-2":dbl format="%_4g"
  out "T3He2-1":dbl format="%_4g"
  out "T1K1":dbl format="%_4g"
  out "T4He1":dbl format="%_4g"
  out "TTH1":dbl format="%_4g"
  out "TTH2":dbl format="%_4g"
  out "TTH4":dbl format="%_4g"
  out "TTH3":dbl format="%_4g"
  out "T3He1-1":dbl format="%_4g"
  out "T3He10":dbl format="%_4g"
  out "F2 (shield flow)":dbl format="%_4f"
  out "DP_HEX4":dbl format="%_4e"
  in  "4K reservoir level":string="L3"
  out "L3":dbl format="%_4f"
  out "RUN Identifier 6":string="20230719_105623_CHF2023" caption="RUN Identifier"
  in  "HEX7 out pressure":string="P_HEX7OUT"
  in  "CHF Graph Comment":string="CHF_RUN13"
  in  "REFRESH GRAPH":bool
  in  "RECORD GRAPH":bool
  out "Graph CHF log 2":T4(graph) caption="XY Graph"
  out "ƒ¢T_array":dbl[](array[numeric])=[-0.007199999999999873, -0.007199999999999873, -0.007100000000000106, -0.007100000000000106, -0.007100000000000106, -0.007100000000000106, -0.007400000000000073, -0.007400000000000073, -0.007400000000000073, -0.007400000000000073, -0.007400000000000073, -0.00869999999999993, -0.00869999999999993, -0.00869999999999993, -0.00869999999999993, -0.009399999999999853, -0.009399999999999853, -0.009399999999999853, -0.009399999999999853, -0.00869999999999993, -0.00869999999999993, -0.00869999999999993, -0.00869999999999993, -0.006000000000000005, -0.006000000000000005, -0.008299999999999974, -0.008299999999999974, -0.008299999999999974, -0.008299999999999974, -0.008299999999999974, -0.0046000000000001595, -0.0046000000000001595, -0.0046000000000001595, -0.0046000000000001595, -0.007500000000000062, -0.007500000000000062, -0.0025000000000001688, -0.0025000000000001688, -0.0025000000000001688, -0.0025000000000001688, -0.00029999999999996696, -0.00029999999999996696, -0.00029999999999996696, -0.00029999999999996696, -0.0026999999999999247, -0.0026999999999999247, -0.0026999999999999247, 0.0028999999999999027, 0.0028999999999999027, 0.0028999999999999027, 0.0028999999999999027, 0.0025999999999999357, 0.0025999999999999357, 0.0025999999999999357, 0.0025999999999999357, 0.005599999999999827, 0.005599999999999827, 0.005599999999999827, 0.005599999999999827, 0.006399999999999961, 0.006399999999999961, 0.013600000000000056, 0.013600000000000056, 0.013600000000000056, 0.013600000000000056, 0.013600000000000056, 0.018500000000000183, 0.018500000000000183, 0.018500000000000183, 0.018500000000000183, 0.014900000000000135, 0.014900000000000135, 0.014900000000000135, 0.014900000000000135, 0.023199999999999887, 0.023199999999999887, 0.024899999999999922, 0.024899999999999922, 0.024899999999999922, 0.024899999999999922, 0.024899999999999922, 0.03080000000000016, 0.03080000000000016, 0.03080000000000016, 0.03080000000000016, 0.03479999999999994, 0.03479999999999994, 0.03479999999999994, 0.03479999999999994, 0.039999999999999813, 0.039999999999999813, 0.04710000000000014, 0.04710000000000014, 0.04710000000000014, 0.04710000000000014, 0.04899999999999993, 0.04899999999999993, 0.04899999999999993, 0.04899999999999993, 0.04899999999999993, 0.055399999999999894, 0.055399999999999894, 0.055399999999999894, 0.055399999999999894, 0.056599999999999984, 0.056599999999999984, 0.0651999999999997, 0.0651999999999997, 0.0651999999999997, 0.0651999999999997, 0.06809999999999983, 0.06809999999999983, 0.06809999999999983, 0.06809999999999983, 0.06809999999999983, 0.0757000000000001, 0.0757000000000001, 0.0757000000000001, 0.0757000000000001, 0.07920000000000016, 0.07920000000000016, 0.07920000000000016, 0.07920000000000016, 0.08809999999999985, 0.08809999999999985, 0.08809999999999985, 0.08809999999999985, 0.09220000000000006, 0.09220000000000006, 0.10330000000000017, 0.10330000000000017, 0.10330000000000017, 0.10330000000000017, 0.10330000000000017, 0.11239999999999983, 0.11239999999999983, 0.11239999999999983, 0.11239999999999983, 0.11450000000000027, 0.11450000000000027, 0.11450000000000027, 0.11450000000000027, 0.11780000000000013, 0.11780000000000013, 0.11080000000000001, 0.11080000000000001, 0.11080000000000001, 0.11080000000000001, 0.13419999999999987, 0.13419999999999987, 0.13419999999999987, 0.13419999999999987, 0.13419999999999987, 0.1434000000000002, 0.1434000000000002, 0.1434000000000002, 0.1434000000000002, 0.14870000000000005, 0.14870000000000005, 0.16070000000000007, 0.16070000000000007, 0.16070000000000007, 0.16070000000000007, 0.17449999999999988, 0.17449999999999988, 0.17449999999999988, 0.17449999999999988, 0.1776000000000002, 0.1776000000000002, 0.1776000000000002, 0.1776000000000002, 0.1776000000000002, 0.1828000000000003, 0.1828000000000003, 0.1828000000000003, 0.1828000000000003, 0.19720000000000004, 0.19720000000000004, 0.2064999999999999, 0.2064999999999999, 0.2064999999999999, 0.2064999999999999, 0.21720000000000006, 0.21720000000000006, 0.21720000000000006, 0.21720000000000006, 0.21720000000000006, 0.21629999999999971, 0.21629999999999971, 0.22709999999999986, 0.22709999999999986, 0.22709999999999986, 0.22709999999999986, 0.2370000000000001, 0.2370000000000001, 0.2370000000000001, 0.2370000000000001, 0.2470000000000001, 0.2470000000000001, 0.2470000000000001, 0.2470000000000001, 0.25460000000000016, 0.25460000000000016, 0.25460000000000016, 0.25460000000000016, 0.25460000000000016, 0.26419999999999977, 0.26419999999999977, 0.2744, 0.2744, 0.2744, 0.2744, 0.28439999999999976, 0.28439999999999976, 0.28439999999999976, 0.28439999999999976, 0.2901, 0.2901, 0.2901, 0.2901, 0.2129000000000003, 0.2129000000000003, 0.2129000000000003, 0.13389999999999969, 0.13389999999999969, 0.13389999999999969, 0.13389999999999969, 0.05500000000000016, 0.05500000000000016, 0.05500000000000016, 0.05500000000000016, 0.025900000000000034, 0.025900000000000034, 0.025900000000000034, 0.025900000000000034, 0.06000000000000005, 0.06000000000000005, 0.06559999999999988, 0.06559999999999988, 0.06559999999999988, 0.06559999999999988, 0.06559999999999988, 0.026499999999999968, 0.026499999999999968, 0.026499999999999968, 0.026499999999999968, 0.0466000000000002, 0.0466000000000002, 0.0466000000000002, 0.0466000000000002, 0.17149999999999999, 0.17149999999999999, 0.17149999999999999, 0.17149999999999999, 0.23720000000000008, 0.23720000000000008, 0.23720000000000008, 0.23720000000000008, 0.23720000000000008, 0.22160000000000002, 0.22160000000000002, 0.22160000000000002]
  out "Graph CHF":cluster{dbl[], dbl[]}(graph)
  out "V":dbl=39.8877222
  out "I":dbl=0.512303718
  out "Q":dbl=20.434628385611138
  out "T_low":dbl=2.1784
  out "Graph CHF log 1":T4(graph) caption="XY Graph"
  out "CHF Data Labels":string[](array[string])=["I_H", "V_H", "P_yokogawa", "P_Horiba", "Level", "Kikusui_V_MON", "Kikusui_I_MON", "H_V", "T_Cu", "T_He"]
  out "CHF last data":dbl[](array[numeric])=[0.512303718, 39.8877222, -50002.111838482066, -0.7873463781670694, -0.005254182819311032, 40.990082197003616, 513.6482603879665, 0.034866352755703184, 2.4, 2.1784]
  out "Error out (CHF rec)":errorcluster
  out "CHF measurement counter":i32
  out "T_high":dbl=2.4
  out "ƒ¢T":dbl=0.22160000000000002
  out "Q_array":dbl[](array[numeric])=[4.127401428334401e-08, 4.127401428334401e-08, 4.127401428334401e-08, 4.127401428334401e-08, 0.0014636100296856248, 0.0014636100296856248, 0.0014636100296856248, 0.0014636100296856248, 0.014543418849067999, 0.014543418849067999, 0.014543418849067999, 0.014543418849067999, 0.014543418849067999, 0.03924009430914699, 0.03924009430914699, 0.03924009430914699, 0.03924009430914699, 0.07443989686341417, 0.07443989686341417, 0.07443989686341417, 0.07443989686341417, 0.12091715111624018, 0.12091715111624018, 0.12091715111624018, 0.12091715111624018, 0.1786395044898887, 0.1786395044898887, 0.1786395044898887, 0.1786395044898887, 0.1786395044898887, 0.24712862797531324, 0.24712862797531324, 0.24712862797531324, 0.24712862797531324, 0.3275519629777947, 0.3275519629777947, 0.3275519629777947, 0.3275519629777947, 0.4186165452566927, 0.4186165452566927, 0.4186165452566927, 0.4186165452566927, 0.5208831592555557, 0.5208831592555557, 0.5208831592555557, 0.5208831592555557, 0.5208831592555557, 0.6343878740253031, 0.6343878740253031, 0.6343878740253031, 0.6343878740253031, 0.7585276907155796, 0.7585276907155796, 0.7585276907155796, 0.7585276907155796, 0.8923458670460318, 0.8923458670460318, 0.8923458670460318, 0.8923458670460318, 1.0386523155285559, 1.0386523155285559, 1.0386523155285559, 1.0386523155285559, 1.0386523155285559, 1.1969341291160438, 1.1969341291160438, 1.1969341291160438, 1.1969341291160438, 1.3673977838780702, 1.3673977838780702, 1.3673977838780702, 1.3673977838780702, 1.5470680284405687, 1.5470680284405687, 1.5470680284405687, 1.5470680284405687, 1.7387284272658998, 1.7387284272658998, 1.7387284272658998, 1.7387284272658998, 1.7387284272658998, 1.9413112117211908, 1.9413112117211908, 1.9413112117211908, 1.9413112117211908, 2.1570408363240086, 2.1570408363240086, 2.1570408363240086, 2.1570408363240086, 2.3809825434175638, 2.3809825434175638, 2.3809825434175638, 2.3809825434175638, 2.6173240335749126, 2.6173240335749126, 2.6173240335749126, 2.6173240335749126, 2.6173240335749126, 2.8628895382863337, 2.8628895382863337, 2.8628895382863337, 2.8628895382863337, 3.1217260906079214, 3.1217260906079214, 3.1217260906079214, 3.1217260906079214, 3.388731762138769, 3.388731762138769, 3.388731762138769, 3.388731762138769, 3.6694986562755165, 3.6694986562755165, 3.6694986562755165, 3.6694986562755165, 3.959860078129326, 3.959860078129326, 3.959860078129326, 3.959860078129326, 3.959860078129326, 4.262717794423667, 4.262717794423667, 4.262717794423667, 4.262717794423667, 4.573693684239568, 4.573693684239568, 4.573693684239568, 4.573693684239568, 4.898093869305062, 4.898093869305062, 4.898093869305062, 4.898093869305062, 5.230620775216983, 5.230620775216983, 5.230620775216983, 5.230620775216983, 5.230620775216983, 5.579670862072944, 5.579670862072944, 5.579670862072944, 5.579670862072944, 5.93407362278231, 5.93407362278231, 5.93407362278231, 5.93407362278231, 6.303630520840891, 6.303630520840891, 6.303630520840891, 6.303630520840891, 6.683926740087989, 6.683926740087989, 6.683926740087989, 6.683926740087989, 6.683926740087989, 7.07505134041537, 7.07505134041537, 7.07505134041537, 7.07505134041537, 7.476471560262807, 7.476471560262807, 7.476471560262807, 7.476471560262807, 7.88820603691946, 7.88820603691946, 7.88820603691946, 7.88820603691946, 8.313406301141132, 8.313406301141132, 8.313406301141132, 8.313406301141132, 8.313406301141132, 8.750385250146007, 8.750385250146007, 8.750385250146007, 8.750385250146007, 9.195533395012008, 9.195533395012008, 9.195533395012008, 9.195533395012008, 9.65227348104519, 9.65227348104519, 9.65227348104519, 9.65227348104519, 10.121912587637079, 10.121912587637079, 10.121912587637079, 10.121912587637079, 10.121912587637079, 10.601947141630403, 10.601947141630403, 10.601947141630403, 10.601947141630403, 11.09151985577636, 11.09151985577636, 11.09151985577636, 11.09151985577636, 11.591597634155027, 11.591597634155027, 11.591597634155027, 11.591597634155027, 12.10291786333025, 12.10291786333025, 12.10291786333025, 12.10291786333025, 12.10291786333025, 12.625298221386252, 12.625298221386252, 12.625298221386252, 12.625298221386252, 13.1568716125126, 13.1568716125126, 13.1568716125126, 13.1568716125126, 13.701379032657679, 13.701379032657679, 13.701379032657679, 13.701379032657679, 14.258107749588685, 14.258107749588685, 14.258107749588685, 14.258107749588685, 14.825450890446854, 14.825450890446854, 14.825450890446854, 14.825450890446854, 14.825450890446854, 15.401931323763176, 15.401931323763176, 15.401931323763176, 15.401931323763176, 15.989058770907702, 15.989058770907702, 15.989058770907702, 15.989058770907702, 16.58963541826619, 16.58963541826619, 16.58963541826619, 16.58963541826619, 17.20455023250212, 17.20455023250212, 17.20455023250212, 17.20455023250212, 17.20455023250212, 17.822741169278203, 17.822741169278203, 17.822741169278203, 17.822741169278203, 18.46281032377074, 18.46281032377074, 18.46281032377074, 18.46281032377074, 19.107769414825285, 19.107769414825285, 19.107769414825285, 19.107769414825285, 19.76703712962949, 19.76703712962949, 19.76703712962949, 19.76703712962949, 19.76703712962949, 20.434628385611138, 20.434628385611138, 20.434628385611138]
  out "CHF file name":string="20230706_132211_CHF2023_CHF20230706_160853_CHF_RUN13.csv"
  out "Graph CHF log 3":T4(graph) caption="XY Graph"
  out "File Refnum (CHF)":refnum<file>
  in  "Tab Control":T15(tab)
  in  "Tab Control 5":enum32{"Kenwood", "Kikusui"}(tab)=enum."Kikusui"
  in  "V_start (V)":dbl format="%_4f"
  in  "V_end (V)":dbl=65.0 format="%_4f"
  in  "ƒ¢V / cycle (V)":dbl=0.5 format="%_4f"
  in  "ƒ¢I / cycle (mA)":dbl=2.0 format="%_4f"
  in  "I_end (mA)":dbl=1000.0 format="%_4f"
  in  "I_start (mA)":dbl format="%_4f"
  in  "CHF cycle interval (s) (>1s)":dbl=1.0 format="%_3f"
  in  "Data I":T16={"Source"=enum."DMMs", "SourceLabel"="I_H"}
  in  "Data V":T16={"Source"=enum."DMMs", "SourceLabel"="V_H"}
  in  "RecordSettings":T17(array[cluster])=[{"Source"=enum."DMMs", "SourceLabel"="I_H", "FileFormat"="%4.4e"}, {"Source"=enum."DMMs", "SourceLabel"="V_H", "FileFormat"="%4.4f"}, {"Source"=enum."USB6218AI", "SourceLabel"="P_yokogawa", "FileFormat"="%5.5e"}, {"Source"=enum."USB6218AI", "SourceLabel"="P_Horiba", "FileFormat"="%5.5f"}, {"Source"=enum."USB6218AI", "SourceLabel"="Level", "FileFormat"="%5.5f"}, {"Source"=enum."USB6218AI", "SourceLabel"="Kikusui_V_MON", "FileFormat"="%5.5f"}, {"Source"=enum."USB6218AI", "SourceLabel"="Kikusui_I_MON", "FileFormat"="%5.5f"}, {"Source"=enum."USB6218AI", "SourceLabel"="H_V", "FileFormat"="%5.5f"}, {"Source"=enum."LSI336", "SourceLabel"="T_Cu", "FileFormat"="%4.4f"}, {"Source"=enum."LSI336", "SourceLabel"="T_He", "FileFormat"="%4.4f"}]
  in  "Data T_high":T16={"Source"=enum."LSI336", "SourceLabel"="T_Cu"}
  in  "Data T_low":T16={"Source"=enum."LSI336", "SourceLabel"="T_He"}
  out "CHF log file name":string="20230706_132211_CHF2023_20230706_162135_CHFlog.csv"
  in  "STOP CHF":bool
  in  "START CHF":bool
  in  "V_peak":dbl=65.0 format="%_4f"
  out "Heat Cycle counter":i32=3
  in  "t_off":dbl=5.0 format="%_4f"
  in  "t_on":dbl=10.0 format="%_4f"
  in  "Q_input":dbl=65.0 format="%_4f"
  out "V_input":dbl=1.0 format="%_4f"
  out "R_sample":dbl=65.0 format="%_4f"
  in  "V_sample":dbl=65.0 format="%_4f"
  out "Q_sample":dbl=65.0 format="%_4f"
  in  "I_sample":dbl=1.0 format="%_4f"
  in  "START heater cycle":bool
  in  "STOP heater cycle":bool
  in  "CHF power supply selection":bool=TRUE
  in  "Tab Control 4":enum32{"Kenwood", "Kikusui PWR400"}(tab)=enum."Kikusui PWR400"
  in  "Kenwood set V (V)":dbl min=0.0 max=120.0 format="%_5f"
  in  "OUTPUT \nKenwood":bool
  in  "VISA (Agilent 34402)":refnum<visa-resource-name>="USB0::0x0957::0x0407::MY44010230::INSTR"
  in  "V_lim_low (V)":dbl format="%_5f"
  out "error out (Agilent)":errorcluster
  in  "V_lim_up (V)":dbl=120.0 format="%_5f"
  in  "Initialize (Agilent)":bool
  out "Agilent\nIntialized?":bool
  in  "Kikusui I (mA)":dbl min=0.0 max=120.0 format="%_5f"
  in  "OUTPUT \nKikusui":bool
  in  "I_lim_up (mA)":dbl=50.0 format="%_5f"
  in  "I_lim_low (mA)":dbl format="%_5f"
  out "Series 1":string[](array[string])=["T_Cu", "T_He"]
  out "Series 2":string[](array[string])=["P_yokogawa", "P_Horiba", "R_L2-2", "L2-2"]
  out "Series 3":string[](array[string])=["Level"]
  out "Series 4":string[](array[string])=["Kikusui_V_MON", "Kikusui_I_MON", "H_V"]
  out "Plot errors":errorcluster
  out "LastMeasurementConfig (218)":T18(array[cluster])=[{"LSIName"="LSI218A", "Active?"=FALSE, "LastData"=[0.0, 0.0, 0.0, 0.0, 0.0, 0.0, 0.0, 0.0], "Labels"=["T3He10", "T3He1-1", "TTH3", "TTH4", "TTH1", "TTH2", "T4He1", "T1K1"]}, {"LSIName"="LSI218B", "Active?"=FALSE, "LastData"=[0.0, 0.0, 0.0, 0.0, 0.0, 0.0, 0.0, 0.0], "Labels"=["N.C.", "N.C.", "N.C.", "N.C.", "T3He2-1", "T3He2-2", "T3He3", "T3He1-4"]}, {"LSIName"="LSI218C", "Active?"=FALSE, "LastData"=[0.0, 0.0, 0.0, 0.0, 0.0, 0.0, 0.0, 0.0], "Labels"=["T4He3-1", "T4He3-2", "T4He3-3", "T4He3-4", "T4He2-1", "T4He2-2", "T4He4", "T4He5"]}, {"LSIName"="LSI218D", "Active?"=FALSE, "LastData"=[0.0, 0.0, 0.0, 0.0, 0.0, 0.0, 0.0, 0.0], "Labels"=["T4He6", "T4He9", "T3He1-2", "T3He1-3", "T4He7", "T4He8", "T4He10", "T1K6"]}, {"LSIName"="LSI218E", "Active?"=FALSE, "LastData"=[0.0, 0.0, 0.0, 0.0, 0.0, 0.0, 0.0, 0.0], "Labels"=["TIP1", "N.C.", "TIP2", "N.C.", "TIP3", "TIP4", "TIP5", "N.C."]}, {"LSIName"="LSI218F", "Active?"=FALSE, "LastData"=[0.0, 0.0, 0.0, 0.0, 0.0, 0.0, 0.0, 0.0], "Labels"=["T1K2", "T1K4", "T1K5", "T3He4", "T3He9", "TIP6", "N.C.", "N.C."]}]
  out "DataArrayConv (USB6210)":dbl[][](array[numeric])
  out "LastMeasurementConfig (336)":T18(array[cluster])=[{"LSIName"="LSi336X", "Active?"=TRUE, "LastData"=[298.66, 298.457, 0.0, 0.0], "Labels"=["T_Cu", "T_He", "N.C\n\n\n", "N.C"]}, {"LSIName"="LSi336Y", "Active?"=FALSE, "LastData"=[0.0, 0.0, 0.0, 0.0, 0.0, 0.0, 0.0, 0.0], "Labels"=["T3He6-1", "T3He6-2", "T3He7-1", "T3He7-2"]}]
  out "DataArrayConv (USB6218)":dbl[][](array[numeric])=[[100115.65601302785, 14307.663228328058, 0.018423510306911722, -19.27655297204919, 36.05601549196442, 0.02105436509847161]]
  out "TimeArray (USB6218)":timestamp[](array[timestamp])=[timestamp(3772576585.022536 s since 1904-01-01)]
  out "Data Array sizes (6210)":i32[](array[numeric])
  out "DataArraySize (6218)":i32[](array[numeric])=[1, 6]
  out "TimeArray size (6218)":i32=1
  out "TimeArray (LSI336)":timestamp[](array[timestamp])=[timestamp(3772576585.022536 s since 1904-01-01)]
  out "TimeArray Size (336)":i32=1
  out "DataArray (336)":dbl[][](array[numeric])=[[298.66, 298.457, 0.0, 0.0, 0.0, 0.0, 0.0, 0.0, 0.0, 0.0, 0.0, 0.0]]
  out "DataArray size (336)":i32[](array[numeric])=[1, 12]
  out "LastData (LSI218)":dbl[](array[numeric])
  out "TempSensorsLocations":T19(array[ring])=[enum."T3He10", enum."T3He1-1", enum."TTH3", enum."TTH4", enum."TTH1", enum."TTH2", enum."T4He1", enum."T1K1", enum."N.C.", enum."N.C.", enum."N.C.", enum."N.C.", enum."T3He2-1", enum."T3He2-2", enum."T3He3", enum."T3He1-4", enum."T4He3-1", enum."T4He3-2", enum."T4He3-3", enum."T4He3-4", enum."T4He2-1", enum."T4He2-2", enum."T4He4", enum."T4He5", enum."T4He6", enum."T4He9", enum."T3He1-2", enum."T3He1-3", enum."T4He7", enum."T4He8", enum."T4He10", enum."T1K6", enum."TIP1", enum."N.C.", enum."TIP2", enum."N.C.", enum."TIP3", enum."TIP4", enum."TIP5", enum."N.C.", enum."T1K2", enum."T1K4", enum."T1K5", enum."T3He4", enum."T3He9", enum."TIP6", enum."N.C.", enum."N.C.", enum."T1K3-1", enum."T1K3-2", enum."T3He5", enum."T3He8", enum."T3He6-1", enum."T3He6-2", enum."T3He7-1", enum."T3He7-2"]
  out "AllTemperatures":dbl[](array[numeric])=[0.0, 0.0, 0.0, 0.0, 0.0, 0.0, 0.0, 0.0, 0.0, 0.0, 0.0, 0.0, 0.0, 0.0, 0.0, 0.0, 0.0, 0.0, 0.0, 0.0, 0.0, 0.0, 0.0, 0.0, 0.0, 0.0, 0.0, 0.0, 0.0, 0.0, 0.0, 0.0, 0.0, 0.0, 0.0, 0.0, 0.0, 0.0, 0.0, 0.0, 0.0, 0.0, 0.0, 0.0, 0.0, 0.0, 0.0, 0.0, 2.1697, 9.0036, 0.0, 0.0, 0.0, 0.0, 0.0, 0.0, 0.0, 0.0, 0.0, 0.0]
  out "error out (frontpanel screenshots)":errorcluster
  out "error out (graph operations)":errorcluster
  out "error out (monthly folder creation)":errorcluster={"status"=TRUE, "code"=10, "source"="Create Folder in CRYO_MASTER_FULL_CHF2023.vi<APPEND>\nC:\\LabVIEW\\DATA\\Google\\TUCAN Experiments\\KEK_cryotests_2019-2020\\data\\screenshots\\202307"}
  out "RUN Identifier 7":string="20230719_105623_CHF2023" caption="RUN Identifier"
  out "error out (notifier)":errorcluster
  # "GLOBAL STATUS/CONTROL"
  # "Global Settings"
  # "USB6210 Analog inputs Settings"
  # "USB6218 Analog inputs Settings"
  # "USB6218/6210 Digital Outputs"
  # "USB6218 Analog Output Settings"
  # "LSI218 Settings"
  # "LSI336 Settings"
  # "HP 34401A (He level meter)"
  # "Graph screenshots"
  # "Configuration"
  # "Activated only when *FIll state* = TRUE"
  # "Activated only when *FIll state* = TRUE"
  # "Vavle Status"
  # "OPEN"
  # "CLOSED"
  # "ADCMT6240A Control/Status"
  # "ADCMT6240A Initialization"
  # "Set Currents (mA)"
  # "PWR400H CTRL via USB6218"
  # "PMC18-3A CTRL via USB6218"
  # "USB6218 low-level control"
  # "Stepping motor AZD-AX"
  # "DMM configurations"
  # "DMM measurements"
  # "CAUTION: ADCMT 7351 does not have 4-wire resistance measurement function. \n 4-Wire Resistance --> 2-Wire Resistance wih Low Power for this device"
  # "Representative temperatures"
  # "Pressures / Flows"
  # "Labels"
  # "Values"
  # "Helium Levels"
  # "Automatic Boiling Cruve Measurement"
  # "Before the measurement\n - Choose the power supply and intialize the output \n - Refresh the CHF graph if necessary\n - Go to DMMs tab and check that DMM measurement is running \n - Fill in the CHF measurement parameters below \nThen press START CHF!"
  # "Measurement Configurations"
  # "Channel selection"
  # "Q = I x V"
  # "ƒ¢T = T_high - T_low"
  # "Record Configurations"
  # "Beam Heat Emulation"
  # "Before starting, \n - turn off the boiling curve measuremnt on the other tab\n - make sure that the DMMs are running"
  # "Calculator"
  # "Previous measurement:"
  # "Caclulate V which corresponds to derired Q:"
  # "Manual Control of Kenwood"
  # "Manual Control of Kikusui"
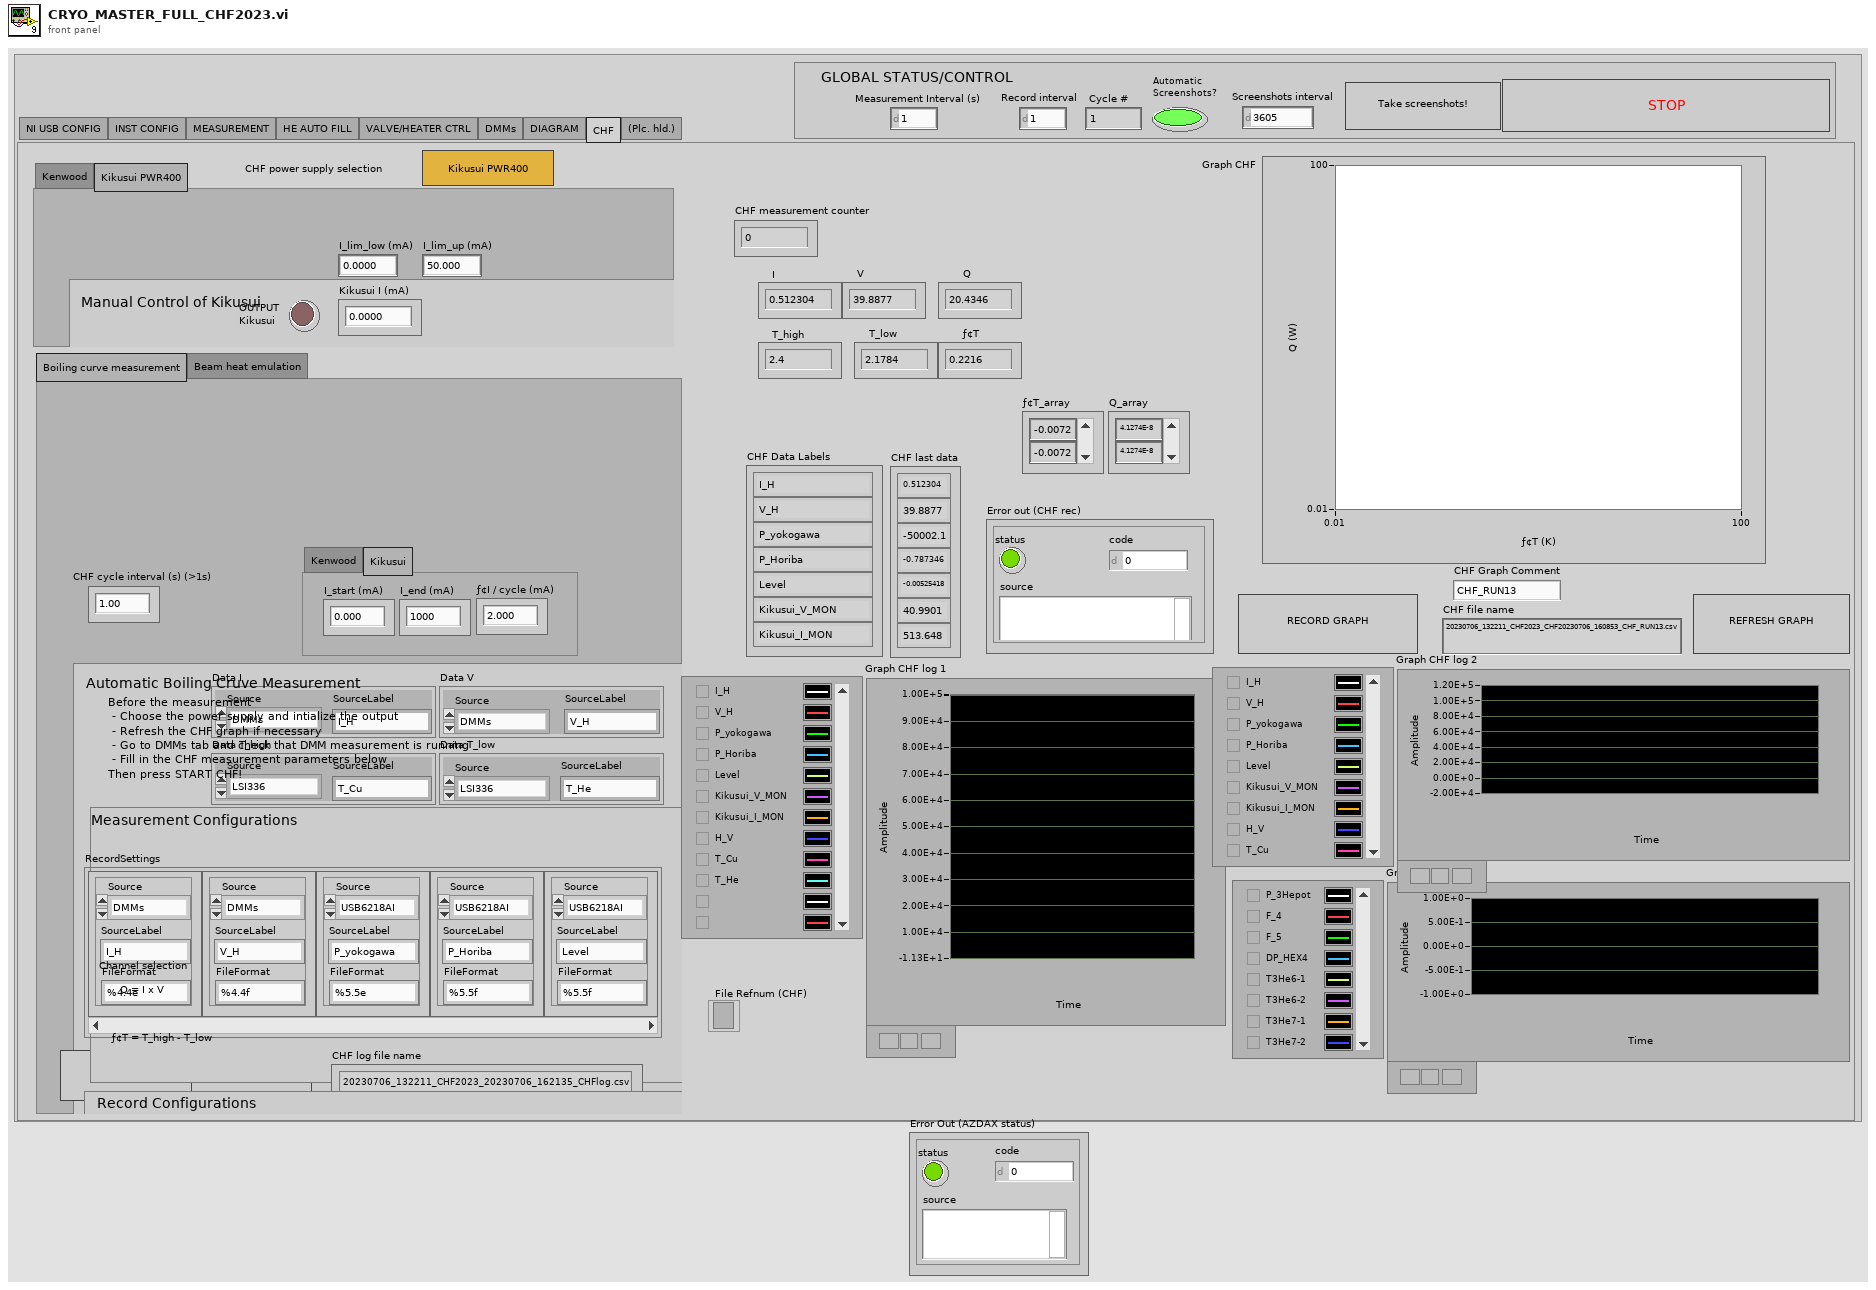
[diagram p1: front panel]
types:
  T1 = enum32{"NI USB CONFIG", "INST CONFIG", "MEASUREMENT", "HE AUTO FILL", "VALVE/HEATER CTRL", "DMMs", "DIAGRAM", "CHF", "(Plc. hld.)"}
  T2 = cluster{"Label":string, "FileFormat":string, "Active?":bool, "Physical CH":tag, " terminal\n type":i32, "ConversionType":cluster{"Type":enum16{"Raw", "SimpleProp", "CC-10_COMBINED", "CC-10_LOG", "LeakDet_EXP", "LeakDet_Mantissa", "Baratron"}, "ConversionParameters":dbl[]}, "VoltageLimits":dbl[]}[]
  T3 = cluster{"LSIName":string, "Labels":string[], "SensorLocations":enum16{"N.C.", "T3He1-1", "T3He1-2", "T3He1-3", "T3He1-4", "T3He2-1", "T3He2-2", "T3He3", "T3He4", "T3He5", "T3He6-1", "T3He6-2", "T3He7-1", "T3He7-2", "T3He8", "T3He9", "T3He10", "T4He1", "T4He2-1", "T4He2-2", "T4He3-1", "T4He3-2", "T4He3-3", "T4He3-4", "T4He4", "T4He5", "T4He6", "T4He7", "T4He8", "T4He9", "T4He10", "T1K1", "T1K2", "T1K3-1", "T1K3-2", "T1K4", "T1K5", "T1K6", "TIP1", "TIP2", "TIP3", "TIP4", "TIP5", "TIP6", "TIP7", "TTH1", "TTH2", "TTH3", "TTH4"}[], "Active?":bool, "VISA res. name":refnum<visa-resource-name>}[]
  T4 = cluster{"TimeArray":timestamp[], "DataArray":dbl[]}[]
  T5 = enum32{"USB6210", "USB6218", "Temeprature (1)", "Temperature (2)", "Temperature (3)"}
  T6 = enum16{"Intialized", "Ready", "Measuring", "Terminated"}
  T7 = enum16{"Initialized", "Ready", "Measuring", "Terminated"}
  T8 = enum16{"USB6210", "USB6218AI", "USB6218AO", "LSI218", "LSI336"}
  T9 = cluster{"TimeArray":timestamp[], "Filtered X":dbl[]}[]
  T10 = cluster{"TimeArray (USB6218)":timestamp[], "DataArrayConv (USB6218)":dbl[]}[]
  T11 = cluster{"Label":string, "Active?":bool, "VISA resource name":refnum<visa-resource-name>, "Device":enum16{"Agilent34401A", "ADCMT7351", "HP3478A", "ADCMT7451"}, "Measurement":enum16{"DC Volts", "DC Currents", "2-Wire Resistance", "4-Wire Resistance"}, "FileFormat":string}[]
  T12 = enum16{"USB6210", "USB6218AI", "USB6218AO", "LSI218", "LSI336"}[]
  T13 = cluster{"Label":string, "Active?":bool, "Source":enum16{"USB6210", "USB6218AI", "USB6218AO", "LSI218", "LSI336"}, "SourceLabel":string, "FileFormat":string}[]
  T14 = enum16{"N.C.", "T3He1-1", "T3He1-2", "T3He1-3", "T3He1-4", "T3He2-1", "T3He2-2", "T3He3", "T3He4", "T3He5", "T3He6-1", "T3He6-2", "T3He7-1", "T3He7-2", "T3He8", "T3He9", "T3He10", "T4He1", "T4He2-1", "T4He2-2", "T4He3-1", "T4He3-2", "T4He3-3", "T4He3-4", "T4He4", "T4He5", "T4He6", "T4He7", "T4He8", "T4He9", "T4He10", "T1K1", "T1K2", "T1K3-1", "T1K3-2", "T1K4", "T1K5", "T1K6", "TIP1", "TIP2", "TIP3", "TIP4", "TIP5", "TIP6", "TIP7", "TTH1", "TTH2", "TTH3", "TTH4"}
  T15 = enum32{"Boiling curve measurement", "Beam heat emulation"}
  T16 = cluster{"Source":enum16{"USB6210", "USB6218AI", "USB6218AO", "LSI218", "LSI336", "DMMs"}, "SourceLabel":string}
  T17 = cluster{"Source":enum16{"USB\n6218\n", "USB6218AI", "USB6218AO", "LSI218", "LSI336", "DMMs"}, "SourceLabel":string, "FileFormat":string}[]
  T18 = cluster{"LSIName":string, "Active?":bool, "LastData":dbl[], "Labels":string[]}[]
  T19 = enum16{"N.C.", "T3He1-1", "T3He1-2", "T3He1-3", "T3He1-4", "T3He2-1", "T3He2-2", "T3He3", "T3He4", "T3He5", "T3He6-1", "T3He6-2", "T3He7-1", "T3He7-2", "T3He8", "T3He9", "T3He10", "T4He1", "T4He2-1", "T4He2-2", "T4He3-1", "T4He3-2", "T4He3-3", "T4He3-4", "T4He4", "T4He5", "T4He6", "T4He7", "T4He8", "T4He9", "T4He10", "T1K1", "T1K2", "T1K3-1", "T1K3-2", "T1K4", "T1K5", "T1K6", "TIP1", "TIP2", "TIP3", "TIP4", "TIP5", "TIP6", "TIP7", "TTH1", "TTH2", "TTH3", "TTH4"}[]
  T20 = cluster{"TimeArray (USB6218)":timestamp[], "DataArrayConv (USB6218)":dbl[]}
  T21 = cluster{"appended array":timestamp[], "ActualCurrentArray":dbl[]}
  T22 = cluster{"appended array":timestamp[], "SetCurrentArray":dbl[]}
  T23 = cluster{"appended array":timestamp[], "SetCurrentArray":dbl[]}[]
  T24 = typedef "imagedata.ctl" = cluster{"image type":i32, "image depth":i32, "image":u8[], "mask":u8[], "colors":u32[], "Rectangle":cluster{"left":i16, "top":i16, "right":i16, "bottom":i16}}
  T25 = enum16{"open", "replace", "create", "open or create", "replace or create", "replace or create with confirmation"}
  T26 = cluster{"TimeArray":timestamp[], "DataArrayConv":dbl[]}[]
  T27 = cluster{"IndexArray":i64[], "TimeArray":timestamp[], "DataArrayRaw":dbl[][], "DataArrayConv":dbl[][], "LDArray":dbl[]}
  T28 = cluster{"InstName":string, "Active?":bool, "Status":enum16{"Intialized", "Ready", "Measuring", "Terminated"}, "Labels":string[], "LabelLD":string, "FileFormat":string[], "FileFormatLD":string, "ReadLeakDet?":bool}
  T29 = cluster{"AOUT Labels[0]":string, "AOUT Labels[1]":string, "AOUT Labels[2]":string, "AOUT Labels[3]":string, "AOUT Labels[4]":string, "AOUT Labels[5]":string, "AOUT Labels[6]":string, "AOUT Labels[7]":string, "AOUT Labels[8]":string}
  T30 = cluster{"LastTimeArray":timestamp[], "LastDataArray":dbl[]}
  T31 = cluster{"LastTimeArray":timestamp[], "LastDataArray":dbl[]}[]
  T32 = cluster{"TimeArray":timestamp[], "DataArrayConv":dbl[]}
  T33 = cluster{"TimeArray":timestamp[], "DataArrayConv (USB6218)":dbl[]}
  T34 = cluster{"TimeArray":timestamp[], "M.A. Array":dbl[]}
  T35 = cluster{"TimeArray":timestamp[], "M.A. Array":dbl[]}[]
  T36 = cluster{"TimeArray":timestamp[], "DataArray":dbl[]}
  T37 = enum16{"USB\n6218\n", "USB6218AI", "USB6218AO", "LSI218", "LSI336", "DMMs"}
  T38 = enum16{"USB6210", "USB6218AI", "USB6218AO", "LSI218", "LSI336", "DMMs"}
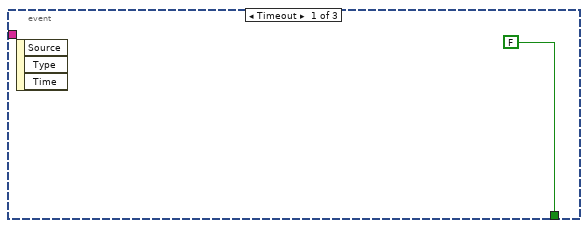
[diagram p3: hidden frame]
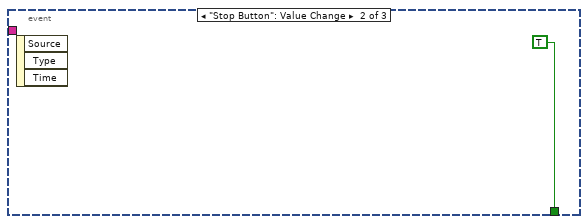
[diagram p4: hidden frame]
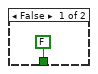
[diagram p5: hidden frame]
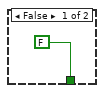
[diagram p7: hidden frame]
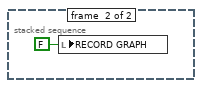
[diagram p9: hidden frame]
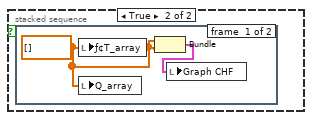
[diagram p10: hidden frame]
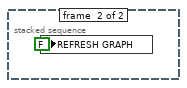
[diagram p11: hidden frame]
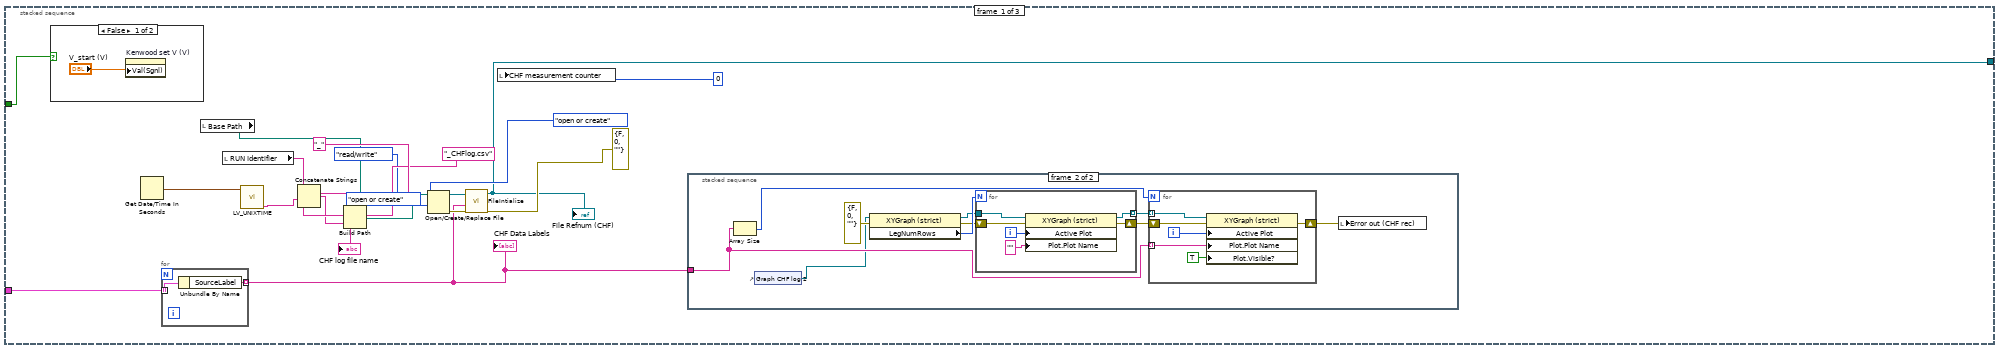
[diagram p13: hidden frame]
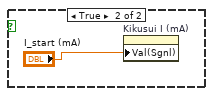
[diagram p14: hidden frame]
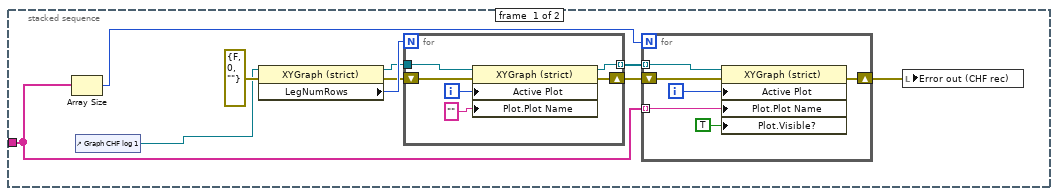
[diagram p15: hidden frame]
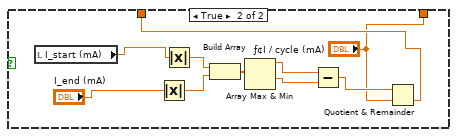
[diagram p16: hidden frame]
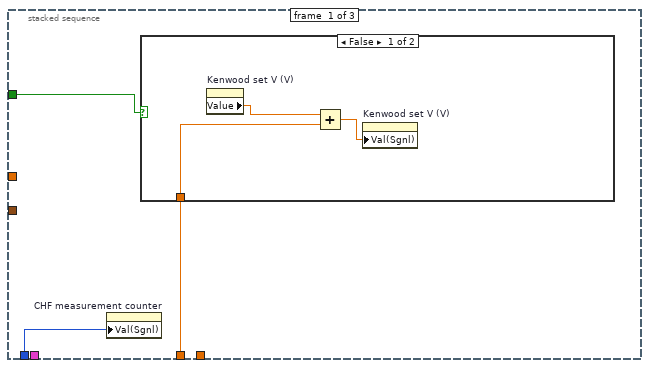
[diagram p17: hidden frame]
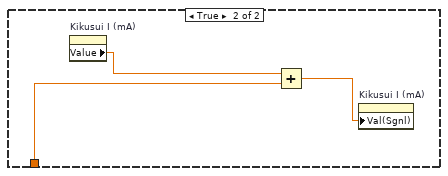
[diagram p18: hidden frame]
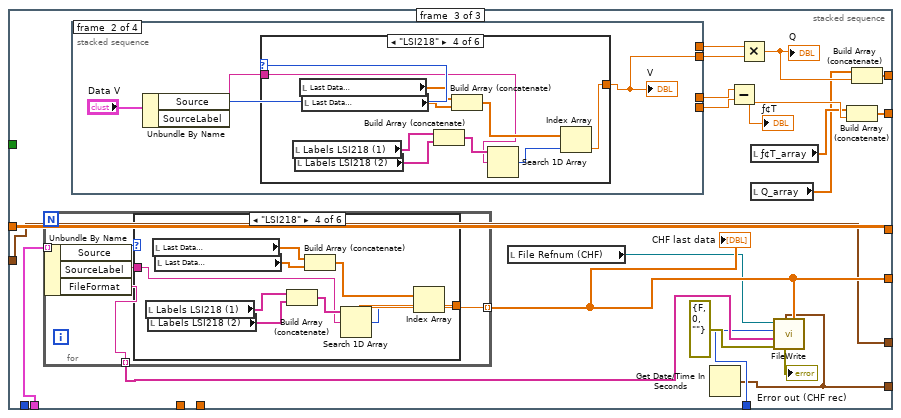
[diagram p19: hidden frame]
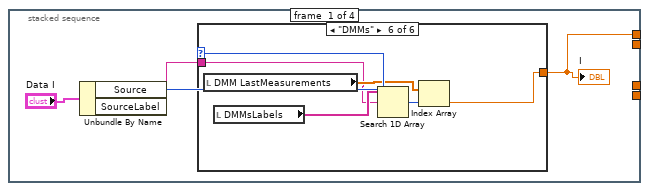
[diagram p20: hidden frame]
diagram:
  w17 = TRUE ("create if not found? (T)")
  w21 = errorcluster {"status"=FALSE, "code"=0, "source"=""} ("error in (no error)")
  w6 = errorcluster {"status"=FALSE, "code"=0, "source"=""} ("error in (no error)")
  n1 = while {
    shift-right: [w45] -> _
    shift-left: dbl[] [] -> [w51]
    shift-right: [w48] -> _
    shift-left: timestamp[] [] -> [w50]
    i -> [w49]
    stop <- w52 stop-if-true
    n2 = Wait (ms)(milliseconds to wait=u32 113) -> ()  [unwired: 1 out]
    n3 = event shown="[3] \"Set Current (mA)  (PMC)\", \"Set Current (mA)  (PWR)\", \"update current\": Value Change" {
      selector: _ -> [_ _ _ _ _ _ _ _]
      dyn-events: _ -> [_ _ _ _ _ _ _ _]
      timeout: _ -> [_ _ _ _ _ _ _ _]
      tunnel: [_ TRUE _ _ _ _ _ _] -> w52
      tunnel: w49 -> [_ _ _ w100 _ _ _ _]
      tunnel: [_ _ _ w99 w183 _ _ _] -> w45
      tunnel: w51 -> [_ _ _ w96 w183 _ _ _]
      tunnel: [w53 w63 _ w98 w182 w186 _ _] -> w48
      tunnel: w50 -> [w53 w63 _ w97 w182 w186 _ _]
      tunnel: [_ _ _ w87 _ _ _ _] -> w44
      event Timeout {
        n4 = event-data() -> ()  [unwired: 1 in, 3 out]
      }
      event "Stop Button": Value Change {
        w54 = FALSE
        n5 = event-data() -> ()  [unwired: 1 in, 3 out]
        n6 = local read "error out (USB6210/6218 DOUT)"() -> (w62:errorcluster)
        n7 = local read "error out (USB6210/6218 AOUT)"() -> (w59:errorcluster)
        n8 = local read "DOUT task out"() -> (w58:refnum<k21>)
        n9 = local read "AO task out"() -> (w65:refnum<k21>)
        n10 = property on="OUTPUT\n(PWR)" class="Bool (strict)"("Value"=w54) -> ()  [unwired: 2 in, 2 out]
        n11 = property on="V2 (N.C.)" class="Bool (strict)"("Val(Sgnl)"=w54) -> ()  [unwired: 2 in, 2 out]
        n12 = property on="OUTPUT\n(PMC)" class="Bool (strict)"("Value"=w54) -> ()  [unwired: 2 in, 2 out]
        n13 = Build Array(w54, w54, w54, w54) -> (w61:bool[])
        n14 = Not(x=w54) -> (.not. x?=w55:bool)
        n15 = call <vilib>:"DAQmx Clear Task.vi"("task in"=w65, "error in"=w59) -> ("error out"=w64:errorcluster)  [unwired: 13 in]
        n16 = property on="V1 (N.O.)" class="Bool (strict)"("Val(Sgnl)"=w55) -> ()  [unwired: 2 in, 2 out]
        n17 = call <vilib>:"DAQmx Write (Digital 1D Bool NChan 1Samp 1Line).vi"("task/channels in"=w58, "data"=w61, "timeout"=10.0, "error in"=w62) -> ("task out"=w57:refnum<k21>, "error out"=w56:errorcluster)  [unwired: 9 in, 1 out]
        n18 = call <vilib>:"DAQmx Clear Task.vi"("task in"=w57, "error in"=w56) -> ("error out"=w66:errorcluster)  [unwired: 13 in]
        n19 = local write "error out (USB6210/6218 AOUT)"(w64) -> ()
        n20 = local write "error out (USB6210/6218 DOUT)"(w66) -> ()
      }
      event "V1 (N.O.)", "V2 (N.C.)": Value Change {
        n21 = event-data() -> ()  [unwired: 1 in, 3 out]
        n22 = local read "Cycle #"() -> (w72:u32)
        n23 = Greater?(x=w72, y=u32 0) -> (0:w70:bool)
        n24 = case shown="False" w70 {
          tunnel: "V1 (N.O.)" -> [_ w83]
          tunnel: "V2 (N.C.)" -> [_ w73]
          frame False {
          }
          frame True {
            n25 = local read "DOUT6218 Labels"() -> (w74:string[])
            n26 = property on="DOUT Raw state" class="Arr (strict)"() -> ("Value"=w82:bool[])  [unwired: 2 in, 2 out]
            n27 = Search 1D Array(1D array=w74, element="D_V1_NO") -> (index of element=w81:i32)  [unwired: 1 in]
            n28 = Search 1D Array(1D array=w74, element="D_V2_NC") -> (index of element=w80:i32)  [unwired: 1 in]
            n29 = Not(x=w83) -> (.not. x?=w76:bool)
            n30 = Replace Array Subset(array=w82, new element=w76, index=w81) -> (w79:bool[])
            n31 = Replace Array Subset(array=w79, new element=w73, index=w80) -> (w78:bool[])
            n32 = property on="DOUT Raw state" class="Arr (strict)"("Val(Sgnl)"=w78) -> ()  [unwired: 2 in, 2 out]
          }
        }
        "V1" <- "V1 (N.O.)"
        "V2" <- "V2 (N.C.)"
      }
      event "Set Current (mA)\n (PMC)", "Set Current (mA)\n (PWR)", "update current": Value Change {
        n33 = event-data() -> ()  [unwired: 1 in, 3 out]
        n34 = case shown="True" "CONTROL KIKUSUI?" {
          tunnel: w100 -> [_ w151]
          tunnel: [w110 w144] -> w99
          tunnel: [w113 w143] -> w98
          tunnel: w97 -> [w115 w146]
          tunnel: w96 -> [w111 w145]
          tunnel: "Set Current (mA)\n (PWR)" -> [_ w123]
          tunnel: "Set Current (mA)\n (PMC)" -> [_ w127]
          frame False {
            w112 = 0.0 ("element")
            n35 = Get Date/Time In Seconds() -> (seconds since 1Jan1904=w114:timestamp)
            n36 = local read "AO task out"() -> (w120:refnum<k21>)
            n37 = Build Array (concatenate)(w115, w114) -> (w113:timestamp[])
            n38 = Build Array (concatenate)(w111, w112) -> (w110:dbl[])
            n39 = Build Array(w112, w112) -> (w118:dbl[])
            n40 = call <vilib>:"DAQmx Write (Analog 1D DBL NChan 1Samp).vi"("task/channels in"=w120, "data"=w118, "timeout"=100.0, "error in"=errorcluster {"status"=FALSE, "code"=0, "source"=""}) -> ("task out"=w121:refnum<k21>, "error out"=w116:errorcluster)  [unwired: 9 in, 1 out]
            n41 = local write "AO task out"(w121) -> ()
            n42 = local write "error out (KIKUSI CTRL)"(w116) -> ()
          }
          frame True {
            w138 = 2 ("index")
            n43 = xnode "Formula"("X1"=w123) -> ("Result"=w140:dbl)  [unwired: 1 in, 1 out]
            n44 = xnode "Formula"("X1"=w127) -> ("Result"=w134:dbl)  [unwired: 1 in, 1 out]
            n45 = Build Array (concatenate)(w145, w123) -> (w144:dbl[])
            n46 = In Range and Coerce(upper limit=10.0, x=w140, lower limit=0.0 ("y")) -> (coerced(x)=w132:dbl, In Range?=w133:bool)
            n47 = In Range and Coerce(upper limit=10.0, x=w134, lower limit=0.0 ("y")) -> (coerced(x)=w129:dbl, In Range?=w130:bool)
            n48 = case shown="False" w133 {
              tunnel: w132 -> [_ w163]
              tunnel: [0.0 ("upper limit") w163] -> w131
              frame False {
              }
              frame True {
              }
            }
            n49 = case shown="True" w130 {
              tunnel: w129 -> [_ w161]
              tunnel: [0.0 ("upper limit") w161] -> w128
              frame False {
              }
              frame True {
              }
            }
            n50 = Multiply(x=w123, y=0.001) -> (x*y=w122:dbl)
            n51 = Multiply(x=w127, y=0.001) -> (x*y=w126:dbl)
            n52 = local read "File Refn USB AO"() -> (w152:refnum<file>)
            n53 = Build Array(w122, w126, w131, w128) -> (w139:dbl[])
            "USB 6218 AOUT" <- w139
            n54 = Initialize Array("%.3f", 4 ("dimension size")) -> (w153:string[])
            n55 = Get Date/Time In Seconds() -> (seconds since 1Jan1904=w147:timestamp)
            n56 = local read "AO task out"() -> (w157:refnum<k21>)
            n57 = call "FileWrite.vi"("DataArray"=w139, "Time Stamp"=w147, "Error In"=errorcluster {"status"=FALSE, "code"=0, "source"=""} ("error in"), "FileFormat"=w153, "Index"=w151, "refnum in"=w152) -> ("Error Out"=w149:errorcluster, "Byte Stream File Refnum"=w148:refnum<file>)  [unwired: 4 in]
            n58 = Build Array (concatenate)(w146, w147) -> (w143:timestamp[])
            n59 = Array Subset(array=w139, index=w138, length=w138) -> (w137:dbl[])
            n60 = local write "File Refn USB AO"(w148) -> ()
            n61 = call <vilib>:"DAQmx Write (Analog 1D DBL NChan 1Samp).vi"("task/channels in"=w157, "data"=w137, "timeout"=100.0, "error in"=w149) -> ("task out"=w158:refnum<k21>, "error out"=→"error out (KIKUSI CTRL)":errorcluster)  [unwired: 9 in, 1 out]
            n62 = local write "AO task out"(w158) -> ()
          }
        }
        n63 = local read "All Labels (USB6218)"() -> (w93:string[])
        n64 = local read "DataArrayConv (USB6218)"() -> (w92:dbl[][])
        n65 = local read "Last Data \n(USB6218)"() -> (w89:dbl[])
        n66 = local read "TimeArray (USB6218)"() -> (w90:timestamp[])
        n67 = Search 1D Array(1D array=w93, element="I_CV") -> (index of element=w94:i32)  [unwired: 1 in]
        n68 = Index Array(array=w92, index (row)=w94) -> (element=w91:dbl[])  [unwired: 1 in]
        n69 = Index Array(array=w89, index=w94) -> (element=w86:dbl)
        n70 = Bundle("TimeArray (USB6218)"=w90, "DataArrayConv (USB6218)"=w91) -> (w87:T20)  [unwired: 1 in]
        n71 = xnode "Formula"("X1"=w86) -> ("Result"=→"Monitor Current (mA)":dbl)  [unwired: 1 in, 1 out]
      }
      event "upper limit (mA)\n (PWR)", "lower limit (mA) \n(PWR)": Value Change {
        n72 = event-data() -> ()  [unwired: 1 in, 6 out]
        n73 = property on="Set Current (mA)\n (PWR)" class="DigNum (strict)"("Maximum"="upper limit (mA)\n (PWR)", "Minimum"="lower limit (mA) \n(PWR)") -> ()  [unwired: 2 in, 2 out]
        n74 = property on="Set Current (mA)\n (PMC)" class="DigNum (strict)"("Maximum"="upper limit (mA)\n (PMC)", "Minimum"="lower limit (mA) \n(PMC)") -> ()  [unwired: 2 in, 2 out]
      }
      event "OUTPUT\n(PWR)", "OUTPUT\n(PMC)": Value Change {
        n75 = event-data() -> ()  [unwired: 1 in, 6 out]
        n76 = local read "Cycle #"() -> (w189:u32)
        n77 = Greater?(x=w189, y=u32 0) -> (0:w187:bool)
        n78 = case shown="True" w187 {
          frame False {
          }
          frame True {
            (unwired) FALSE
            n79 = local read "DOUT6218 Labels"() -> (w195:string[])
            n80 = local read "DOUT Raw state"() -> (w190:bool[])
            n81 = Search 1D Array(1D array=w195, element="DOUT (PWR)") -> (index of element=w198:i32)  [unwired: 1 in]
            n82 = Search 1D Array(1D array=w195, element="DOUT (PMC)") -> (index of element=w193:i32)  [unwired: 1 in]
            n83 = Replace Array Subset(array=w190, new element="OUTPUT\n(PWR)", index=w198) -> (w192:bool[])
            n84 = Replace Array Subset(array=w192, new element="OUTPUT\n(PMC)", index=w193) -> (w191:bool[])
            n85 = property on="DOUT Raw state" class="Arr (strict)"("Val(Sgnl)"=w191) -> ()  [unwired: 2 in, 2 out]
          }
        }
      }
      event "Motor stop", "Close 1/4", "Open 1/4", "Motor home": Value Change {
        n86 = event-data() -> ()  [unwired: 1 in, 6 out]
        n87 = Divide(x="Current position", y=10.0) -> (x/y=w210:dbl)
        n88 = Multiply(x=w210, y=100.0) -> (x*y=→"Opening rate (Closed:0, Full open:100)":dbl)
        n89 = Multiply(x="wait for home (s)", y=1000) -> (x*y=w201:dbl)
        n90 = Multiply(x="wait for open/close/stop (s)", y=1000) -> (x*y=w203:dbl)
        n91 = stacked-sequence {
          tunnel: u32 100 ("milliseconds to wait") -> [w213 w254 w293 w322 _]
          tunnel: w203 -> [w212 w253 _ w321 _]
          tunnel: w201 -> [_ _ w290 _ _]
          frame #0 {
            n92 = case shown="True" "Open 1/4" {
              tunnel: "AZD-AZ open" -> [_ w221]
              tunnel: w213 -> [_ w220]
              tunnel: w212 -> [_ w219]
              frame False {
              }
              frame True {
                n93 = local read "Current position"() -> (w218:dbl)
                n94 = Less?(x=w218, y=10.0) -> (x < y?=w216:bool)
                n95 = case shown="False" w216 {
                  tunnel: w221 -> [_ w226]
                  tunnel: w220 -> [_ w225]
                  tunnel: w219 -> [_ w224]
                  frame False {
                    n96 = local write "Open 1/4"(FALSE ("Open 1/4")) -> ()
                    n97 = local write "AZD-AZ status"("Cannot open further!" ("AZD-AZ status")) -> ()
                  }
                  frame True {
                    n98 = flat-sequence {
                      tunnel: w226 -> [w229]
                      tunnel: [w229] -> w228
                      tunnel: w225 -> [w237]
                      tunnel: w228 -> [w236]
                      tunnel: [w236] -> w227
                      tunnel: w227 -> [w239]
                      tunnel: w224 -> [w246]
                      frame #0 {
                        n99 = local read "DOUT6218 Labels"() -> (w234:string[])
                        n100 = local read "DOUT Raw state"() -> (w233:bool[])
                        n101 = Search 1D Array(1D array=w234, element=w229) -> (index of element=w232:i32)  [unwired: 1 in]
                        n102 = Replace Array Subset(array=w233, new element=TRUE ("new element/subarray"), index=w232) -> (w230:bool[])
                        n103 = property on="DOUT Raw state" class="Arr (strict)"("Val(Sgnl)"=w230) -> ()  [unwired: 2 in, 2 out]
                      }
                      frame #1 {
                        n104 = Wait (ms)(milliseconds to wait=w237) -> ()  [unwired: 1 out]
                        n105 = local write "AZD-AZ status"("Command sent \"open 1/4\"" ("AZD-AZ status")) -> ()
                      }
                      frame #2 {
                        n106 = local read "DOUT6218 Labels"() -> (w240:string[])
                        n107 = local read "DOUT Raw state"() -> (w241:bool[])
                        n108 = Search 1D Array(1D array=w240, element=w239) -> (index of element=w242:i32)  [unwired: 1 in]
                        n109 = Replace Array Subset(array=w241, new element=FALSE ("new element/subarray"), index=w242) -> (w244:bool[])
                        n110 = property on="Open 1/4" class="Bool (strict)"("Val(Sgnl)"=FALSE ("Value (Signaling)")) -> ()  [unwired: 2 in, 2 out]
                        n111 = property on="DOUT Raw state" class="Arr (strict)"("Val(Sgnl)"=w244) -> ()  [unwired: 2 in, 2 out]
                      }
                      frame #3 {
                        n112 = local write "AZD-AZ status"("In operation..." ("AZD-AZ status")) -> ()
                        n113 = Wait (ms)(milliseconds to wait=w246) -> ()  [unwired: 1 out]
                      }
                      frame #4 {
                        n114 = property on="Current position" class="DigNum (strict)"() -> ("Value"=w250:dbl)  [unwired: 2 in, 2 out]
                        n115 = Add(x=w250, y=0.25) -> (x+y=w247:dbl)
                        n116 = local write "AZD-AZ status"("Operation complete" ("AZD-AZ status")) -> ()
                        n117 = property on="Current position" class="DigNum (strict)"("Val(Sgnl)"=w247) -> ()  [unwired: 2 in, 2 out]
                      }
                    }
                  }
                }
              }
            }
          }
          frame #1 {
            n118 = case shown="True" "Close 1/4" {
              tunnel: "AZD-AZ close" -> [_ w260]
              tunnel: w254 -> [_ w259]
              tunnel: w253 -> [_ w258]
              frame False {
              }
              frame True {
                n119 = local read "Current position"() -> (w257:dbl)
                n120 = Greater?(x=w257, y=0.0) -> (0:w255:bool)
                n121 = case shown="False" w255 {
                  tunnel: w260 -> [_ w265]
                  tunnel: w259 -> [_ w264]
                  tunnel: w258 -> [_ w263]
                  frame False {
                    n122 = local write "AZD-AZ status"("Cannot close further!" ("AZD-AZ status")) -> ()
                    n123 = local write "Close 1/4"(FALSE ("Value (Signaling)")) -> ()
                  }
                  frame True {
                    n124 = flat-sequence {
                      tunnel: w265 -> [w268]
                      tunnel: [w268] -> w267
                      tunnel: w264 -> [w276]
                      tunnel: w267 -> [w275]
                      tunnel: [w275] -> w266
                      tunnel: w266 -> [w278]
                      tunnel: w263 -> [w285]
                      frame #0 {
                        n125 = local read "DOUT6218 Labels"() -> (w273:string[])
                        n126 = local read "DOUT Raw state"() -> (w272:bool[])
                        n127 = Search 1D Array(1D array=w273, element=w268) -> (index of element=w271:i32)  [unwired: 1 in]
                        n128 = Replace Array Subset(array=w272, new element=TRUE ("new element/subarray"), index=w271) -> (w269:bool[])
                        n129 = property on="DOUT Raw state" class="Arr (strict)"("Val(Sgnl)"=w269) -> ()  [unwired: 2 in, 2 out]
                      }
                      frame #1 {
                        n130 = Wait (ms)(milliseconds to wait=w276) -> ()  [unwired: 1 out]
                        n131 = local write "AZD-AZ status"("Command sent \"close 1/4\"" ("AZD-AZ status")) -> ()
                      }
                      frame #2 {
                        n132 = local read "DOUT6218 Labels"() -> (w279:string[])
                        n133 = local read "DOUT Raw state"() -> (w280:bool[])
                        n134 = Search 1D Array(1D array=w279, element=w278) -> (index of element=w281:i32)  [unwired: 1 in]
                        n135 = Replace Array Subset(array=w280, new element=FALSE ("new element/subarray"), index=w281) -> (w283:bool[])
                        n136 = property on="Close 1/4" class="Bool (strict)"("Val(Sgnl)"=FALSE ("Value (Signaling)")) -> ()  [unwired: 2 in, 2 out]
                        n137 = property on="DOUT Raw state" class="Arr (strict)"("Val(Sgnl)"=w283) -> ()  [unwired: 2 in, 2 out]
                      }
                      frame #3 {
                        n138 = local write "AZD-AZ status"("In operation..." ("AZD-AZ status")) -> ()
                        n139 = Wait (ms)(milliseconds to wait=w285) -> ()  [unwired: 1 out]
                      }
                      frame #4 {
                        n140 = property on="Current position" class="DigNum (strict)"() -> ("Value"=w288:dbl)  [unwired: 2 in, 2 out]
                        n141 = Subtract(x=w288, y=0.25) -> (x-y=w286:dbl)
                        n142 = local write "AZD-AZ status"("Operation complete" ("AZD-AZ status")) -> ()
                        n143 = property on="Current position" class="DigNum (strict)"("Val(Sgnl)"=w286) -> ()  [unwired: 2 in, 2 out]
                      }
                    }
                  }
                }
              }
            }
          }
          frame #2 {
            n144 = case shown="True" "Motor home" {
              tunnel: "AZD-AZ home" -> [_ w298]
              tunnel: w293 -> [_ w297]
              tunnel: w290 -> [_ w294]
              frame False {
              }
              frame True {
                n145 = flat-sequence {
                  tunnel: w298 -> [w299]
                  tunnel: [w299] -> w296
                  tunnel: w297 -> [w307]
                  tunnel: w296 -> [w306]
                  tunnel: [w306] -> w295
                  tunnel: w295 -> [w309]
                  tunnel: w294 -> [w316]
                  frame #0 {
                    n146 = local read "DOUT6218 Labels"() -> (w304:string[])
                    n147 = local read "DOUT Raw state"() -> (w303:bool[])
                    n148 = Search 1D Array(1D array=w304, element=w299) -> (index of element=w302:i32)  [unwired: 1 in]
                    n149 = Replace Array Subset(array=w303, new element=TRUE ("new element/subarray"), index=w302) -> (w300:bool[])
                    n150 = property on="DOUT Raw state" class="Arr (strict)"("Val(Sgnl)"=w300) -> ()  [unwired: 2 in, 2 out]
                  }
                  frame #1 {
                    n151 = Wait (ms)(milliseconds to wait=w307) -> ()  [unwired: 1 out]
                    n152 = local write "AZD-AZ status"("Command sent \"Go home\"" ("AZD-AZ status")) -> ()
                  }
                  frame #2 {
                    n153 = local read "DOUT6218 Labels"() -> (w310:string[])
                    n154 = local read "DOUT Raw state"() -> (w311:bool[])
                    n155 = Search 1D Array(1D array=w310, element=w309) -> (index of element=w312:i32)  [unwired: 1 in]
                    n156 = property on="Motor home" class="Bool (strict)"("Val(Sgnl)"=FALSE ("Value (Signaling)")) -> ()  [unwired: 2 in, 2 out]
                    n157 = Replace Array Subset(array=w311, new element=FALSE ("new element/subarray"), index=w312) -> (w314:bool[])
                    n158 = property on="DOUT Raw state" class="Arr (strict)"("Val(Sgnl)"=w314) -> ()  [unwired: 2 in, 2 out]
                  }
                  frame #3 {
                    n159 = local write "AZD-AZ status"("In operation..." ("AZD-AZ status")) -> ()
                    n160 = Wait (ms)(milliseconds to wait=w316) -> ()  [unwired: 1 out]
                  }
                  frame #4 {
                    n161 = local write "AZD-AZ status"("Operation complete" ("AZD-AZ status")) -> ()
                    n162 = property on="Current position" class="DigNum (strict)"("Val(Sgnl)"=0.0 ("y")) -> ()  [unwired: 2 in, 2 out]
                  }
                }
              }
            }
          }
          frame #3 {
            n163 = case shown="True" "Motor stop" {
              tunnel: "AZD-AZ stop" -> [_ w327]
              tunnel: w322 -> [_ w326]
              tunnel: w321 -> [_ w323]
              frame False {
              }
              frame True {
                n164 = flat-sequence {
                  tunnel: w327 -> [w328]
                  tunnel: [w328] -> w325
                  tunnel: w326 -> [w336]
                  tunnel: w325 -> [w335]
                  tunnel: [w335] -> w324
                  tunnel: w324 -> [w338]
                  tunnel: w323 -> [w345]
                  frame #0 {
                    n165 = local read "DOUT6218 Labels"() -> (w333:string[])
                    n166 = local read "DOUT Raw state"() -> (w332:bool[])
                    n167 = Search 1D Array(1D array=w333, element=w328) -> (index of element=w331:i32)  [unwired: 1 in]
                    n168 = Replace Array Subset(array=w332, new element=TRUE ("new element/subarray"), index=w331) -> (w329:bool[])
                    n169 = property on="DOUT Raw state" class="Arr (strict)"("Val(Sgnl)"=w329) -> ()  [unwired: 2 in, 2 out]
                  }
                  frame #1 {
                    n170 = Wait (ms)(milliseconds to wait=w336) -> ()  [unwired: 1 out]
                    n171 = local write "AZD-AZ status"("Command sent \"Stop\"" ("AZD-AZ status")) -> ()
                  }
                  frame #2 {
                    n172 = local read "DOUT6218 Labels"() -> (w339:string[])
                    n173 = local read "DOUT Raw state"() -> (w340:bool[])
                    n174 = Search 1D Array(1D array=w339, element=w338) -> (index of element=w341:i32)  [unwired: 1 in]
                    n175 = Replace Array Subset(array=w340, new element=FALSE ("new element/subarray"), index=w341) -> (w343:bool[])
                    n176 = property on="Motor stop" class="Bool (strict)"("Val(Sgnl)"=FALSE ("Value (Signaling)")) -> ()  [unwired: 2 in, 2 out]
                    n177 = property on="DOUT Raw state" class="Arr (strict)"("Val(Sgnl)"=w343) -> ()  [unwired: 2 in, 2 out]
                  }
                  frame #3 {
                    n178 = local write "AZD-AZ status"("In operation..." ("AZD-AZ status")) -> ()
                    n179 = Wait (ms)(milliseconds to wait=w345) -> ()  [unwired: 1 out]
                  }
                  frame #4 {
                    n180 = local write "AZD-AZ status"("Operation complete" ("AZD-AZ status")) -> ()
                  }
                }
              }
            }
          }
          frame #4 {
            n181 = local read "Cycle #"() -> (w353:u32)
            n182 = local read "File ref AZD-AX status"() -> (w352:refnum<file>)
            n183 = property on="Current position" class="DigNum (strict)"() -> ("Value"=w350:dbl)  [unwired: 2 in, 2 out]
            n184 = Get Date/Time In Seconds() -> (seconds since 1Jan1904=w351:timestamp)
            n185 = Build Array(w350) -> (w349:dbl[])
            n186 = call "FileWrite.vi"("DataArray"=w349, "Time Stamp"=w351, "Error In"=errorcluster {"status"=FALSE, "code"=0, "source"=""}, "FileFormat"=string[] ["%.2f"], "Index"=w353, "refnum in"=w352) -> ("Error Out"=→"Error Out (AZDAX status)":errorcluster)  [unwired: 4 in, 1 out]
          }
        }
      }
      event "Open N", "Close N": Value Change {
        n187 = event-data() -> ()  [unwired: 1 in, 6 out]
        n188 = property on="Current position" class="DigNum (strict)"() -> ("Value"=w355:dbl)  [unwired: 2 in, 2 out]
        n189 = Divide(x=w355, y=10.0) -> (x/y=w362:dbl)
        n190 = Multiply(x=w362, y=100.0) -> (x*y=w356:dbl)
        n191 = property on="Opening rate (Closed:0, Full open:100)" class="Knob (strict)"("Val(Sgnl)"=w356) -> ()  [unwired: 2 in, 2 out]
        n192 = local read "wait for open/close/stop (s)"() -> (w357:dbl)
        n193 = Multiply(x=w357, y=1000) -> (x*y=w358:dbl)
        n194 = stacked-sequence {
          tunnel: u32 100 ("milliseconds to wait") -> [w370 w435]
          tunnel: w358 -> [w369 w434]
          frame #0 {
            n195 = local read "AZD-AZ open"() -> (w364:string)
            n196 = Multiply(x="N to open", y=u64 4) -> (x*y=w365:u64)
            n197 = case shown="True" "Open N" {
              tunnel: w364 -> [_ w380]
              tunnel: w370 -> [_ w379]
              tunnel: w369 -> [_ w378]
              tunnel: w365 -> [_ w374]
              frame False {
              }
              frame True {
                n198 = property on="Current position" class="DigNum (strict)"() -> ("Value"=w377:dbl)  [unwired: 2 in, 2 out]
                n199 = Multiply(x=0.25, y=w374) -> (x*y=w376:dbl)
                n200 = Add(x=w377, y=w376) -> (x+y=w373:dbl)
                n201 = Less Or Equal?(x=w373, y=9.9) -> (x <= y?=w371:bool)
                "Open Command accepted" <- w371
                n202 = case shown="False" w371 {
                  tunnel: w380 -> [_ w386]
                  tunnel: w379 -> [_ w385]
                  tunnel: w378 -> [_ w384]
                  tunnel: w374 -> [_ w383]
                  frame False {
                    n203 = local write "AZD-AZ status"("Cannot open further!" ("AZD-AZ status")) -> ()
                    n204 = local write "Open N"(FALSE ("Close N")) -> ()
                  }
                  frame True {
                    n205 = for {
                      N: w383 -> [w394]
                      tunnel: w386 -> [w399]
                      tunnel: w385 -> [w398]
                      tunnel: w384 -> [w397]
                      i -> [w396]
                      (unwired) errorcluster {"status"=FALSE, "code"=0, "source"=""} ("Error In")
                      n206 = stacked-sequence {
                        tunnel: w399 -> [w400 _ w408 _ _]
                        tunnel: w398 -> [_ w407 _ _ _]
                        tunnel: w396 -> [_ _ w413 _ _]
                        tunnel: w394 -> [_ _ w412 _ _]
                        tunnel: w397 -> [_ _ _ w421 _]
                        tunnel: [_ _ _ _ w425] -> w389
                        frame #0 {
                          n207 = local read "DOUT6218 Labels"() -> (w405:string[])
                          n208 = local read "DOUT Raw state"() -> (w404:bool[])
                          n209 = Search 1D Array(1D array=w405, element=w400) -> (index of element=w403:i32)  [unwired: 1 in]
                          n210 = Replace Array Subset(array=w404, new element=TRUE ("new element/subarray"), index=w403) -> (w401:bool[])
                          n211 = property on="DOUT Raw state" class="Arr (strict)"("Val(Sgnl)"=w401) -> ()  [unwired: 2 in, 2 out]
                        }
                        frame #1 {
                          n212 = Wait (ms)(milliseconds to wait=w407) -> ()  [unwired: 1 out]
                          n213 = local write "AZD-AZ status"("Command sent \"open 1/4\"" ("AZD-AZ status")) -> ()
                        }
                        frame #2 {
                          n214 = Subtract(x=w412, y=1) -> (x-y=w410:i32)
                          n215 = local read "DOUT6218 Labels"() -> (w414:string[])
                          n216 = Equal?(x=w413, y=w410) -> (x = y?=w409:bool)
                          n217 = case shown="True" w409 {
                            frame False {
                            }
                            frame True {
                              n218 = property on="Open N" class="Bool (strict)"("Val(Sgnl)"=FALSE ("Value (Signaling)")) -> ()  [unwired: 2 in, 2 out]
                            }
                          }
                          n219 = local read "DOUT Raw state"() -> (w415:bool[])
                          n220 = Search 1D Array(1D array=w414, element=w408) -> (index of element=w416:i32)  [unwired: 1 in]
                          n221 = Replace Array Subset(array=w415, new element=FALSE ("new element/subarray"), index=w416) -> (w418:bool[])
                          n222 = property on="DOUT Raw state" class="Arr (strict)"("Val(Sgnl)"=w418) -> ()  [unwired: 2 in, 2 out]
                        }
                        frame #3 {
                          n223 = local write "AZD-AZ status"("In operation..." ("AZD-AZ status")) -> ()
                          n224 = Wait (ms)(milliseconds to wait=w421) -> ()  [unwired: 1 out]
                        }
                        frame #4 {
                          n225 = property on="Current position" class="DigNum (strict)"() -> ("Value"=w426:dbl)  [unwired: 2 in, 2 out]
                          n226 = property on="Opening rate (Closed:0, Full open:100)" class="Knob (strict)"() -> ("Value"=w423:dbl)  [unwired: 2 in, 2 out]
                          n227 = Add(x=w423, y=2.5) -> (x+y=w422:dbl)
                          n228 = Add(x=w426, y=0.25) -> (x+y=w425:dbl)
                          n229 = local write "AZD-AZ status"("Operation complete" ("AZD-AZ status")) -> ()
                          n230 = property on="Current position" class="DigNum (strict)"("Val(Sgnl)"=w425) -> ()  [unwired: 2 in, 2 out]
                          n231 = property on="Opening rate (Closed:0, Full open:100)" class="Knob (strict)"("Val(Sgnl)"=w422) -> ()  [unwired: 2 in, 2 out]
                        }
                      }
                      n232 = Subtract(x=w394, y=w396) -> (x-y=w395:i32)
                      n233 = local write "... more steps"(w395) -> ()
                      n234 = local read "Cycle #"() -> (w393:u32)
                      n235 = local read "File ref AZD-AX status"() -> (w392:refnum<file>)
                      n236 = Get Date/Time In Seconds() -> (seconds since 1Jan1904=w391:timestamp)
                      n237 = Build Array(w389) -> (w388:dbl[])
                      n238 = call "FileWrite.vi"("DataArray"=w388, "Time Stamp"=w391, "FileFormat"=string[] ["%.2f"], "Index"=w393, "refnum in"=w392) -> ("Error Out"=w390:errorcluster)  [unwired: 5 in, 1 out]
                      n239 = local write "Error Out (AZDAX status)"(w390) -> ()
                    }
                  }
                }
              }
            }
          }
          frame #1 {
            n240 = local read "AZD-AZ close"() -> (w433:string)
            n241 = Multiply(x="N to close", y=u64 4) -> (x*y=w429:u64)
            n242 = case shown="True" "Close N" {
              tunnel: w433 -> [_ w446]
              tunnel: w435 -> [_ w445]
              tunnel: w434 -> [_ w444]
              tunnel: w429 -> [_ w443]
              tunnel: w429 -> [_ w441]
              frame False {
              }
              frame True {
                n243 = property on="Current position" class="DigNum (strict)"() -> ("Value"=w439:dbl)  [unwired: 2 in, 2 out]
                n244 = Multiply(x=0.25, y=w441) -> (x*y=w440:dbl)
                n245 = Subtract(x=w439, y=w440) -> (x-y=w438:dbl)
                n246 = Greater Or Equal?(x=w438, y=0.0) -> (x >= y?=w436:bool)
                "Close Command accepted" <- w436
                n247 = case shown="False" w436 {
                  tunnel: w446 -> [_ w452]
                  tunnel: w445 -> [_ w451]
                  tunnel: w444 -> [_ w450]
                  tunnel: w443 -> [_ w449]
                  frame False {
                    n248 = local write "Close N"(FALSE ("Close N")) -> ()
                    n249 = local write "AZD-AZ status"("Cannot close further!" ("AZD-AZ status")) -> ()
                  }
                  frame True {
                    n250 = flat-sequence {
                      tunnel: w452 -> [w456]
                      tunnel: w451 -> [w455]
                      tunnel: w450 -> [w454]
                      tunnel: w449 -> [w453]
                      frame #0 {
                        n251 = for {
                          N: w453 -> [w468]
                          tunnel: w456 -> [w457]
                          tunnel: w455 -> [w471]
                          tunnel: w454 -> [w470]
                          i -> [w466]
                          n252 = Subtract(x=w468, y=w466) -> (x-y=w467:i32)
                          n253 = stacked-sequence {
                            tunnel: w471 -> [_ w479 _ _ _]
                            tunnel: w468 -> [_ _ w484 _ _]
                            tunnel: w467 -> [_ _ _ _ _]
                            tunnel: w466 -> [_ _ w482 _ _]
                            tunnel: w470 -> [_ _ _ w493 _]
                            tunnel: [_ _ _ _ w497] -> w460
                            tunnel: w457 -> [w472 _ w480 _ _]
                            frame #0 {
                              n254 = local read "DOUT6218 Labels"() -> (w477:string[])
                              n255 = local read "DOUT Raw state"() -> (w476:bool[])
                              n256 = Search 1D Array(1D array=w477, element=w472) -> (index of element=w475:i32)  [unwired: 1 in]
                              n257 = Replace Array Subset(array=w476, new element=TRUE ("new element/subarray"), index=w475) -> (w473:bool[])
                              n258 = property on="DOUT Raw state" class="Arr (strict)"("Val(Sgnl)"=w473) -> ()  [unwired: 2 in, 2 out]
                            }
                            frame #1 {
                              n259 = local write "AZD-AZ status"("Command sent \"close 1/4\"" ("AZD-AZ status")) -> ()
                              n260 = Wait (ms)(milliseconds to wait=w479) -> ()  [unwired: 1 out]
                            }
                            frame #2 {
                              n261 = local read "DOUT6218 Labels"() -> (w487:string[])
                              n262 = local read "DOUT Raw state"() -> (w488:bool[])
                              n263 = Search 1D Array(1D array=w487, element=w480) -> (index of element=w489:i32)  [unwired: 1 in]
                              n264 = Replace Array Subset(array=w488, new element=FALSE ("new element/subarray"), index=w489) -> (w490:bool[])
                              n265 = property on="DOUT Raw state" class="Arr (strict)"("Val(Sgnl)"=w490) -> ()  [unwired: 2 in, 2 out]
                              n266 = Subtract(x=w484, y=1) -> (x-y=w483:i32)
                              n267 = Equal?(x=w482, y=w483) -> (x = y?=w481:bool)
                              n268 = case shown="True" w481 {
                                frame False {
                                }
                                frame True {
                                n269 = property on="Close N" class="Bool (strict)"("Val(Sgnl)"=FALSE ("new element/subarray")) -> ()  [unwired: 2 in, 2 out]
                                }
                              }
                            }
                            frame #3 {
                              n270 = local write "AZD-AZ status"("In operation..." ("AZD-AZ status")) -> ()
                              n271 = Wait (ms)(milliseconds to wait=w493) -> ()  [unwired: 1 out]
                            }
                            frame #4 {
                              n272 = property on="Current position" class="DigNum (strict)"() -> ("Value"=w498:dbl)  [unwired: 2 in, 2 out]
                              n273 = property on="Opening rate (Closed:0, Full open:100)" class="Knob (strict)"() -> ("Value"=w495:dbl)  [unwired: 2 in, 2 out]
                              n274 = Subtract(x=w495, y=2.5) -> (x-y=w496:dbl)
                              n275 = Subtract(x=w498, y=0.25) -> (x-y=w497:dbl)
                              n276 = local write "AZD-AZ status"("Operation complete" ("AZD-AZ status")) -> ()
                              n277 = property on="Current position" class="DigNum (strict)"("Val(Sgnl)"=w497) -> ()  [unwired: 2 in, 2 out]
                              n278 = property on="Opening rate (Closed:0, Full open:100)" class="Knob (strict)"("Val(Sgnl)"=w496) -> ()  [unwired: 2 in, 2 out]
                            }
                          }
                          n279 = local write "... more steps"(w467) -> ()
                          n280 = Wait (ms)(milliseconds to wait=u32 5) -> ()  [unwired: 1 out]
                          n281 = local read "File ref AZD-AX status"() -> (w464:refnum<file>)
                          n282 = local read "Cycle #"() -> (w465:u32)
                          n283 = Get Date/Time In Seconds() -> (seconds since 1Jan1904=w463:timestamp)
                          n284 = Build Array(w460) -> (w459:dbl[])
                          n285 = call "FileWrite.vi"("DataArray"=w459, "Time Stamp"=w463, "Error In"=errorcluster {"status"=FALSE, "code"=0, "source"=""}, "FileFormat"=string[] ["%.2f"], "Index"=w465, "refnum in"=w464) -> ("Error Out"=w458:errorcluster)  [unwired: 4 in, 1 out]
                          n286 = local write "Error Out (AZDAX status)"(w458) -> ()
                        }
                      }
                      frame #1 {
                        n287 = local write "... more steps"(u64 1 ("... more steps")) -> ()
                      }
                    }
                  }
                }
              }
            }
          }
        }
      }
    }
    n288 = Bundle(w48, w45) -> (w47:cluster{timestamp[], dbl[]})  [unwired: 1 in]
    n289 = Build Array(w47, w44) -> (→"Graph 7":T10)
  }
  n290 = while {
    i -> [w505]
    stop <- w507 stop-if-true
    n291 = local read "DOUT6218 Labels"() -> (w502:string[])
    "DOUT Labels 2" <- w502
    n292 = Wait (ms)(milliseconds to wait=u32 99) -> ()  [unwired: 1 out]
    n293 = Equal?(x=w505, y=0) -> (x = y?=w503:bool)
    n294 = case shown="True" w503 {
      tunnel: w502 -> [_ w510]
      frame False {
      }
      frame True {
        n295 = Array Size(array=w510) -> (size(s)=w509:i32)
        n296 = for {
          N: w509 -> [_]
          tunnel: [FALSE] -> w508 mode=indexing
        }
        n297 = property on="DOUT Raw state" class="Arr (strict)"("Val(Sgnl)"=w508) -> ()  [unwired: 2 in, 2 out]
      }
    }
    n298 = event shown="[2] \"DOUT Raw state\": Value Change" {
      selector: _ -> [_ _ _]
      dyn-events: _ -> [_ _ _]
      timeout: _ -> [_ _ _]
      tunnel: [FALSE TRUE w519] -> w507
      tunnel: w502 -> [_ _ w514]
      event Timeout {
        n299 = event-data() -> ()  [unwired: 1 in, 3 out]
      }
      event "Stop Button": Value Change {
        n300 = event-data() -> ()  [unwired: 1 in, 3 out]
      }
      event "DOUT Raw state": Value Change {
        n301 = event-data() -> ()  [unwired: 1 in, 3 out]
        n302 = local read "Cycle #"() -> (w516:u32)
        n303 = Greater?(x=w516, y=u32 0) -> (0:w517:bool)
        n304 = case shown="True" w517 {
          tunnel: [FALSE FALSE] -> w519
          tunnel: w516 -> [_ w525]
          tunnel: "DOUT Raw state" -> [_ w524]
          tunnel: "DOUT Raw state" -> [_ w523]
          tunnel: w514 -> [_ w522]
          frame False {
          }
          frame True {
            n305 = local read "error out (USB6210/6218 DOUT)"() -> (w528:errorcluster)
            n306 = local read "DOUT task out"() -> (w527:refnum<k21>)
            n307 = Array Size(array=w522) -> (size(s)=w521:i32)
            n308 = local read "File Refn USB DO"() -> (w536:refnum<file>)
            n309 = Boolean To (0,1)(Boolean=w524) -> (0, 1=w538:i16[])
            n310 = call <vilib>:"DAQmx Write (Digital 1D Bool NChan 1Samp 1Line).vi"("task/channels in"=w527, "data"=w523, "timeout"=10.0, "error in"=w528) -> ("task out"=w530:refnum<k21>, "error out"=w532:errorcluster)  [unwired: 9 in, 1 out]
            n311 = Initialize Array("%d" ("element"), w521) -> (w534:string[])
            n312 = local write "DOUT task out"(w530) -> ()
            n313 = Get Date/Time In Seconds() -> (seconds since 1Jan1904=w535:timestamp)
            n314 = call "FileWrite.vi"("DataArray"=w538, "Time Stamp"=w535, "Error In"=w532, "FileFormat"=w534, "Index"=w525, "refnum in"=w536) -> ("Error Out"=w533:errorcluster, "Byte Stream File Refnum"=w537:refnum<file>)  [unwired: 4 in]
            n315 = local write "File Refn USB DO"(w537) -> ()
            n316 = local write "error out (USB6210/6218 DOUT)"(w533) -> ()
          }
        }
      }
    }
  }
  n317 = while {
    shift-right: [w547] -> _
    shift-left: refnum<class "6240AData.lvclass"> refnum ("6240AData.lvclass") -> [w545]
    shift-right: [w543] -> _
    shift-left: errorcluster {"status"=FALSE, "code"=0, "source"=""} ("error in (no error)") -> [w544]
    i -> [w539]
    stop <- w546 stop-if-true
    n318 = Wait (ms)(milliseconds to wait=u32 231) -> ()  [unwired: 1 out]
    n319 = Equal?(x=w539, y=0) -> (x = y?=w541:bool)
    n320 = case shown="True" w541 {
      frame False {
      }
      frame True {
        n321 = property on="Initialized?" class="Bool (strict)"("Val(Sgnl)"=FALSE ("Value (Signaling)")) -> ()  [unwired: 2 in, 2 out]
      }
    }
    n322 = event shown="[1] \"update values\", \"SetCurrent 1 (mA)\", \"SetCurrent 2 (mA)\": Value Change" {
      selector: _ -> [_ _ _ _ _]
      dyn-events: _ -> [_ _ _ _ _]
      timeout: _ -> [_ _ _ _ _]
      tunnel: [w550 w565 _ w614 w635] -> w547
      tunnel: [_ _ _ _ TRUE ("Value (Signaling)")] -> w546
      tunnel: w545 -> [w550 w564 _ w598 w633]
      tunnel: w544 -> [w549 w563 _ w597 w631]
      tunnel: [w549 w562 _ w612 w634] -> w543
      tunnel: w539 -> [_ w561 _ _ _]
      tunnel: w539 -> [_ _ _ w606 _]
      event Timeout {
        n323 = event-data() -> ()  [unwired: 1 in, 3 out]
      }
      event "update values", "SetCurrent 1 (mA)", "SetCurrent 2 (mA)": Value Change {
        w554 = 1000.0 ("y")
        n324 = event-data() -> ()  [unwired: 1 in, 6 out]
        n325 = local read "Initialized?"() -> (w560:bool)
        n326 = Divide(x="SetCurrent 1 (mA)", y=w554) -> (x/y=w555:dbl)
        n327 = Divide(x="SetCurrent 2 (mA)", y=w554) -> (x/y=w556:dbl)
        n328 = Build Array(w555, w556) -> (w553:dbl[])
        n329 = Not Equal?(x=w560, y=FALSE) -> (x != y?=w558:bool)
        n330 = case shown="True" w558 {
          tunnel: [w567 w591] -> w565
          tunnel: "Output\n (ADCMT)" -> [_ w590]
          tunnel: w564 -> [w567 w589]
          tunnel: w563 -> [w566 w588]
          tunnel: [w566 w587] -> w562
          tunnel: w561 -> [_ w583]
          tunnel: w553 -> [_ w569]
          frame False {
          }
          frame True {
            w576 = 1 ("index (col)")
            w577 = 0 ("disabled index (col)")
            n331 = call-dynamic "6240AData_execute.vi"("6240AData in"=w589, "SetCurrent (A)"=w569, "FileFormat"="%3.5f", "Output status"=w590, "ExecutionIndex"=w583, "error in (no error)"=w588) -> ("ActualVoltage (V)"=w568:dbl[], "ActualCurrent (A)"=w582:dbl[], "6240AData out"=w591:refnum<class "6240AData.lvclass">, "appended array"=w572:timestamp[], "SetCurrentArray"=w578:dbl[][], "ActualCurrentArray"=w585:dbl[][], "error out"=w587:errorcluster)  [unwired: 3 in]
            n332 = property on="ActualVoltage (V)" class="Arr (strict)"("Val(Sgnl)"=w568) -> ()  [unwired: 2 in, 2 out]
            n333 = property on="ActualCurrent (A)" class="Arr (strict)"("Val(Sgnl)"=w582) -> ()  [unwired: 2 in, 2 out]
            n334 = Index Array(array=w585, index (col) #1=w577, index (col) #2=w576) -> (element #1=w586:dbl[], element #2=w580:dbl[])  [unwired: 2 in]
            n335 = Index Array(array=w578, index (col) #1=w577, index (col) #2=w576) -> (element #1=w574:dbl[], element #2=w571:dbl[])  [unwired: 2 in]
            n336 = Bundle("appended array"=w572, "ActualCurrentArray"=w586) -> (w581:T21)  [unwired: 1 in]
            n337 = Bundle("appended array"=w572, "ActualCurrentArray"=w580) -> (w575:T21)  [unwired: 1 in]
            n338 = Bundle("appended array"=w572, "SetCurrentArray"=w574) -> (w573:T22)  [unwired: 1 in]
            n339 = Bundle("appended array"=w572, "SetCurrentArray"=w571) -> (w570:T22)  [unwired: 1 in]
            n340 = Build Array(w581, w575, w573, w570) -> (→"Graph 6":T23)
          }
        }
      }
      event "upper limit (mA)", "lower limit (mA)": Value Change {
        n341 = event-data() -> ()  [unwired: 1 in, 6 out]
        n342 = property on="SetCurrent 1 (mA)" class="DigNum (strict)"("Maximum"="upper limit (mA)", "Minimum"="lower limit (mA)") -> ()  [unwired: 2 in, 2 out]
        n343 = property on="SetCurrent 2 (mA)" class="DigNum (strict)"("Maximum"="upper limit (mA)", "Minimum"="lower limit (mA)") -> ()  [unwired: 2 in, 2 out]
      }
      event "Initialize": Value Change {
        w608 = FALSE
        n344 = event-data() -> ()  [unwired: 1 in, 6 out]
        n345 = local read "Initialized?"() -> (w596:bool)
        n346 = case shown="True" w596 {
          tunnel: w598 -> [w624 w628]
          tunnel: w597 -> [w623 w627]
          tunnel: [w624 w626] -> w595
          tunnel: [w623 w625] -> w594
          frame False {
          }
          frame True {
            n347 = call-dynamic "6240AData_terrminate.vi"("error in (no error)"=w627, "6240AData in"=w628) -> ("error out"=w625:errorcluster, "6240AData out"=w626:refnum<class "6240AData.lvclass">)  [unwired: 8 in]
          }
        }
        n348 = property on="Initialized?" class="Bool (strict)"("Val(Sgnl)"=TRUE ("Value (Signaling)")) -> ()  [unwired: 2 in, 2 out]
        n349 = local read "SetCurrent 2 (mA)"() -> (w601:dbl)
        n350 = local read "SetCurrent 1 (mA)"() -> (w604:dbl)
        n351 = local read "RUN Identifier"() -> (w616:string)
        n352 = local read "Base Path"() -> (w617:path)
        n353 = Divide(x=w604, y=1000.0) -> (x/y=w603:dbl)
        n354 = Divide(x=w601, y=1000.0) -> (x/y=w600:dbl)
        n355 = Get Date/Time In Seconds() -> ()  [unwired: 1 out]
        n356 = call-dynamic "6240AData_initialize.vi"("6240AData in"=w595, "RunIdentifier"=w616, "InstName"="InstName", "base path"=w617, "VISA"="VISA", "error in (no error)"=w594, "CtrlLabels"="CtrlLabels", "Voltage limits (V)"="Voltage limits (V)") -> ("6240AData out"=w615:refnum<class "6240AData.lvclass">, "error out"=w613:errorcluster)  [unwired: 6 in]
        n357 = Build Array(w603, w600) -> (w599:dbl[])
        n358 = Build Array(w608, w608) -> (w607:bool[])
        n359 = call-dynamic "6240AData_execute.vi"("6240AData in"=w615, "SetCurrent (A)"=w599, "FileFormat"="%3.5f", "Output status"=w607, "ExecutionIndex"=w606, "error in (no error)"=w613) -> ("ActualVoltage (V)"=w610:dbl[], "ActualCurrent (A)"=w609:dbl[], "6240AData out"=w614:refnum<class "6240AData.lvclass">, "error out"=w612:errorcluster)  [unwired: 3 in, 3 out]
        n360 = property on="ActualVoltage (V)" class="Arr (strict)"("Val(Sgnl)"=w610) -> ()  [unwired: 2 in, 2 out]
        n361 = property on="ActualCurrent (A)" class="Arr (strict)"("Val(Sgnl)"=w609) -> ()  [unwired: 2 in, 2 out]
      }
      event "Stop Button": Value Change {
        n362 = event-data() -> ()  [unwired: 1 in, 6 out]
        n363 = local read "Initialized?"() -> (w629:bool)
        n364 = case shown="False" w629 {
          tunnel: w633 -> [w638 w650]
          tunnel: [w638 w649] -> w632
          tunnel: w631 -> [w637 w648]
          tunnel: [w637 w647] -> w630
          frame False {
          }
          frame True {
            w654 = FALSE
            n365 = local read "SetCurrent 2 (mA)"() -> (w640:dbl)
            n366 = local read "SetCurrent 1 (mA)"() -> (w644:dbl)
            n367 = Divide(x=w644, y=1000.0) -> (x/y=w642:dbl)
            n368 = Divide(x=w640, y=1000.0) -> (x/y=w639:dbl)
            n369 = Build Array(w642, w639) -> (w646:dbl[])
            n370 = Build Array(w654, w654) -> (w645:bool[])
            n371 = property on="Output\n (ADCMT)" class="Arr (strict)"("Val(Sgnl)"=w645) -> ()  [unwired: 2 in, 2 out]
            n372 = call-dynamic "6240AData_execute.vi"("6240AData in"=w650, "SetCurrent (A)"=w646, "FileFormat"="%3.5f", "Output status"=w645, "error in (no error)"=w648) -> ("ActualVoltage (V)"=w651:dbl[], "ActualCurrent (A)"=w652:dbl[], "6240AData out"=w649:refnum<class "6240AData.lvclass">, "error out"=w647:errorcluster)  [unwired: 4 in, 3 out]
            n373 = property on="ActualVoltage (V)" class="Arr (strict)"("Val(Sgnl)"=w651) -> ()  [unwired: 2 in, 2 out]
            n374 = property on="ActualCurrent (A)" class="Arr (strict)"("Val(Sgnl)"=w652) -> ()  [unwired: 2 in, 2 out]
          }
        }
        n375 = call-dynamic "6240AData_terrminate.vi"("error in (no error)"=w630, "6240AData in"=w632) -> ("error out"=w634:errorcluster, "6240AData out"=w635:refnum<class "6240AData.lvclass">)  [unwired: 8 in]
      }
    }
    "error out (ADCMT6420A)" <- w543
  }
  n376 = while {
    stop <- w663 stop-if-true
    n377 = Get Date/Time In Seconds() -> (seconds since 1Jan1904=w662:timestamp)
    n378 = Format Date/Time String(time format string (%c)="%Y%m", seconds (now)=w662) -> (date/time string=w659:string)  [unwired: 1 in]
    n379 = Build Path(base path="Base Path (screenshots)", name or relative path=w659) -> (appended path=w658:path)
    n380 = Create Folder(path (use dialog)=w658, error in=errorcluster {"status"=FALSE, "code"=0, "source"=""}) -> (created path=w655:path, error out=→"error out (monthly folder creation)":errorcluster)  [unwired: 1 in, 1 out]
    n381 = event shown="[1] \"Frontpanel screenshots\": Value Change" {
      selector: _ -> [_ _ _]
      dyn-events: _ -> [_ _ _]
      timeout: _ -> [_ _ _]
      tunnel: [FALSE _ TRUE] -> w663
      tunnel: w655 -> [_ w671 _]
      tunnel: w662 -> [_ w670 _]
      event Timeout {
        n382 = event-data() -> ()  [unwired: 1 in, 3 out]
      }
      event "Frontpanel screenshots": Value Change {
        n383 = event-data() -> ()  [unwired: 1 in, 3 out]
        n384 = property class="TabCtl (strict)"() -> ("Value"=w668:T1)  [unwired: 2 in, 2 out]
        n385 = stacked-sequence {
          tunnel: w671 -> [w677 w699 w721 w743 w765 w787 w809 w831 w853 _]
          tunnel: w670 -> [w676 w698 w720 w742 w764 w786 w808 w830 w852 _]
          tunnel: [w674 _ _ _ _ _ _ _ _ _] -> w669
          tunnel: w668 -> [w673 _ _ _ _ _ _ _ _ _]
          tunnel: [w673 _ _ _ _ _ _ _ _ _] -> w667
          tunnel: "cryostatus_" ("string") -> [w672 w695 w717 w739 w761 w783 w805 w827 w849 _]
          frame #0 {
            n386 = flat-sequence {
              tunnel: w676 -> [w679]
              tunnel: [w679] -> w675
              tunnel: w677 -> [w694]
              tunnel: w675 -> [w682]
              tunnel: [w681] -> w674
              tunnel: w672 -> [w680]
              frame #0 {
                n387 = property class="TabCtl (strict)"("Val(Sgnl)"=T1."NI USB CONFIG" ("Value (Signaling)")) -> ()  [unwired: 2 in, 2 out]
              }
              frame #1 {
                w692 = "_" ("string")
                n388 = local read "Cycle #"() -> (w690:u32)
                n389 = call "LV_UNIXTIME.vi"("current time"=w682) -> ("date/time string"=w693:string)  [unwired: 9 in, 1 out]
                n390 = Format Value(format string="%06d", value (0)=w690) -> (output string=w689:string)  [unwired: 1 in]
                n391 = Concatenate Strings(w680, w693, w692, w689, w692, "page1.png" ("string")) -> (w687:string)
                n392 = invoke class="TabCtl (strict)" method="Get Image"(error in=errorcluster {"status"=FALSE, "code"=0, "source"=""} ("error in (no error)")) -> (error out=w683:errorcluster, "image data"=w685:T24)  [unwired: 5 in, 4 out]
                n393 = Build Path(base path=w694, name or relative path=w687) -> (appended path=w686:path)
                n394 = call <vilib>:"Write PNG File.vi"("error in (no error)"=w683, "image data"=w685, "path to PNG file"=w686) -> ("error out"=w681:errorcluster)  [unwired: 7 in, 1 out]
              }
            }
          }
          frame #1 {
            n395 = flat-sequence {
              tunnel: w698 -> [w701]
              tunnel: [w701] -> w697
              tunnel: w699 -> [w716]
              tunnel: w697 -> [w704]
              tunnel: [w703] -> w696
              tunnel: w695 -> [w702]
              frame #0 {
                n396 = property class="TabCtl (strict)"("Val(Sgnl)"=T1."NI USB CONFIG" ("Value (Signaling)")) -> ()  [unwired: 2 in, 2 out]
              }
              frame #1 {
                w714 = "_" ("string")
                n397 = local read "Cycle #"() -> (w712:u32)
                n398 = call "LV_UNIXTIME.vi"("current time"=w704) -> ("date/time string"=w715:string)  [unwired: 9 in, 1 out]
                n399 = Format Value(format string="%06d", value (0)=w712) -> (output string=w711:string)  [unwired: 1 in]
                n400 = Concatenate Strings(w702, w715, w714, w711, w714, "page2.png" ("string")) -> (w709:string)
                n401 = invoke class="TabCtl (strict)" method="Get Image"(error in=errorcluster {"status"=FALSE, "code"=0, "source"=""} ("error in (no error)")) -> (error out=w705:errorcluster, "image data"=w707:T24)  [unwired: 5 in, 4 out]
                n402 = Build Path(base path=w716, name or relative path=w709) -> (appended path=w708:path)
                n403 = call <vilib>:"Write PNG File.vi"("error in (no error)"=w705, "image data"=w707, "path to PNG file"=w708) -> ("error out"=w703:errorcluster)  [unwired: 7 in, 1 out]
              }
            }
            n404 = local write "error out (frontpanel screenshots)"(w696) -> ()
          }
          frame #2 {
            n405 = flat-sequence {
              tunnel: w720 -> [w723]
              tunnel: [w723] -> w719
              tunnel: w721 -> [w738]
              tunnel: w719 -> [w726]
              tunnel: [w725] -> w718
              tunnel: w717 -> [w724]
              frame #0 {
                n406 = property class="TabCtl (strict)"("Val(Sgnl)"=T1."MEASUREMENT" ("Value (Signaling)")) -> ()  [unwired: 2 in, 2 out]
              }
              frame #1 {
                w736 = "_" ("string")
                n407 = local read "Cycle #"() -> (w734:u32)
                n408 = Format Value(format string="%06d", value (0)=w734) -> (output string=w733:string)  [unwired: 1 in]
                n409 = call "LV_UNIXTIME.vi"("current time"=w726) -> ("date/time string"=w737:string)  [unwired: 9 in, 1 out]
                n410 = Concatenate Strings(w724, w737, w736, w733, w736, "page3.png" ("string")) -> (w731:string)
                n411 = invoke class="TabCtl (strict)" method="Get Image"(error in=errorcluster {"status"=FALSE, "code"=0, "source"=""} ("error in (no error)")) -> (error out=w727:errorcluster, "image data"=w729:T24)  [unwired: 5 in, 4 out]
                n412 = Build Path(base path=w738, name or relative path=w731) -> (appended path=w730:path)
                n413 = call <vilib>:"Write PNG File.vi"("error in (no error)"=w727, "image data"=w729, "path to PNG file"=w730) -> ("error out"=w725:errorcluster)  [unwired: 7 in, 1 out]
              }
            }
            n414 = local write "error out (frontpanel screenshots)"(w718) -> ()
          }
          frame #3 {
            n415 = flat-sequence {
              tunnel: w742 -> [w745]
              tunnel: [w745] -> w741
              tunnel: w743 -> [w760]
              tunnel: w741 -> [w748]
              tunnel: [w747] -> w740
              tunnel: w739 -> [w746]
              frame #0 {
                n416 = property class="TabCtl (strict)"("Val(Sgnl)"=T1."HE AUTO FILL" ("Value (Signaling)")) -> ()  [unwired: 2 in, 2 out]
              }
              frame #1 {
                w758 = "_" ("string")
                n417 = local read "Cycle #"() -> (w756:u32)
                n418 = Format Value(format string="%06d", value (0)=w756) -> (output string=w755:string)  [unwired: 1 in]
                n419 = call "LV_UNIXTIME.vi"("current time"=w748) -> ("date/time string"=w759:string)  [unwired: 9 in, 1 out]
                n420 = Concatenate Strings(w746, w759, w758, w755, w758, "page4.png" ("string")) -> (w753:string)
                n421 = invoke class="TabCtl (strict)" method="Get Image"(error in=errorcluster {"status"=FALSE, "code"=0, "source"=""} ("error in (no error)")) -> (error out=w749:errorcluster, "image data"=w751:T24)  [unwired: 5 in, 4 out]
                n422 = Build Path(base path=w760, name or relative path=w753) -> (appended path=w752:path)
                n423 = call <vilib>:"Write PNG File.vi"("error in (no error)"=w749, "image data"=w751, "path to PNG file"=w752) -> ("error out"=w747:errorcluster)  [unwired: 7 in, 1 out]
              }
            }
            n424 = local write "error out (frontpanel screenshots)"(w740) -> ()
          }
          frame #4 {
            n425 = flat-sequence {
              tunnel: w764 -> [w767]
              tunnel: [w767] -> w763
              tunnel: w765 -> [w782]
              tunnel: w763 -> [w770]
              tunnel: [w769] -> w762
              tunnel: w761 -> [w768]
              frame #0 {
                n426 = property class="TabCtl (strict)"("Val(Sgnl)"=T1."VALVE/HEATER CTRL" ("Value (Signaling)")) -> ()  [unwired: 2 in, 2 out]
              }
              frame #1 {
                w780 = "_" ("string")
                n427 = local read "Cycle #"() -> (w778:u32)
                n428 = call "LV_UNIXTIME.vi"("current time"=w770) -> ("date/time string"=w781:string)  [unwired: 9 in, 1 out]
                n429 = Format Value(format string="%06d", value (0)=w778) -> (output string=w777:string)  [unwired: 1 in]
                n430 = Concatenate Strings(w768, w781, w780, w777, w780, "page5.png" ("string")) -> (w775:string)
                n431 = invoke class="TabCtl (strict)" method="Get Image"(error in=errorcluster {"status"=FALSE, "code"=0, "source"=""} ("error in (no error)")) -> (error out=w771:errorcluster, "image data"=w773:T24)  [unwired: 5 in, 4 out]
                n432 = Build Path(base path=w782, name or relative path=w775) -> (appended path=w774:path)
                n433 = call <vilib>:"Write PNG File.vi"("error in (no error)"=w771, "image data"=w773, "path to PNG file"=w774) -> ("error out"=w769:errorcluster)  [unwired: 7 in, 1 out]
              }
            }
            n434 = local write "error out (frontpanel screenshots)"(w762) -> ()
          }
          frame #5 {
            n435 = flat-sequence {
              tunnel: w786 -> [w789]
              tunnel: [w789] -> w785
              tunnel: w787 -> [w804]
              tunnel: w785 -> [w792]
              tunnel: [w791] -> w784
              tunnel: w783 -> [w790]
              frame #0 {
                n436 = property class="TabCtl (strict)"("Val(Sgnl)"=T1."DMMs" ("Value (Signaling)")) -> ()  [unwired: 2 in, 2 out]
              }
              frame #1 {
                w802 = "_" ("string")
                n437 = local read "Cycle #"() -> (w800:u32)
                n438 = call "LV_UNIXTIME.vi"("current time"=w792) -> ("date/time string"=w803:string)  [unwired: 9 in, 1 out]
                n439 = Format Value(format string="%06d", value (0)=w800) -> (output string=w799:string)  [unwired: 1 in]
                n440 = Concatenate Strings(w790, w803, w802, w799, w802, "page6.png" ("string")) -> (w797:string)
                n441 = invoke class="TabCtl (strict)" method="Get Image"(error in=errorcluster {"status"=FALSE, "code"=0, "source"=""} ("error in (no error)")) -> (error out=w793:errorcluster, "image data"=w795:T24)  [unwired: 5 in, 4 out]
                n442 = Build Path(base path=w804, name or relative path=w797) -> (appended path=w796:path)
                n443 = call <vilib>:"Write PNG File.vi"("error in (no error)"=w793, "image data"=w795, "path to PNG file"=w796) -> ("error out"=w791:errorcluster)  [unwired: 7 in, 1 out]
              }
            }
            n444 = local write "error out (frontpanel screenshots)"(w784) -> ()
          }
          frame #6 {
            n445 = flat-sequence {
              tunnel: w808 -> [w811]
              tunnel: [w811] -> w807
              tunnel: w809 -> [w826]
              tunnel: w807 -> [w814]
              tunnel: [w813] -> w806
              tunnel: w805 -> [w812]
              frame #0 {
                n446 = property class="TabCtl (strict)"("Val(Sgnl)"=T1."DIAGRAM" ("Value (Signaling)")) -> ()  [unwired: 2 in, 2 out]
              }
              frame #1 {
                w824 = "_" ("string")
                n447 = local read "Cycle #"() -> (w822:u32)
                n448 = Format Value(format string="%06d", value (0)=w822) -> (output string=w821:string)  [unwired: 1 in]
                n449 = call "LV_UNIXTIME.vi"("current time"=w814) -> ("date/time string"=w825:string)  [unwired: 9 in, 1 out]
                n450 = Concatenate Strings(w812, w825, w824, w821, w824, "page7.png" ("string")) -> (w819:string)
                n451 = invoke class="TabCtl (strict)" method="Get Image"(error in=errorcluster {"status"=FALSE, "code"=0, "source"=""} ("error in (no error)")) -> (error out=w815:errorcluster, "image data"=w817:T24)  [unwired: 5 in, 4 out]
                n452 = Build Path(base path=w826, name or relative path=w819) -> (appended path=w818:path)
                n453 = call <vilib>:"Write PNG File.vi"("error in (no error)"=w815, "image data"=w817, "path to PNG file"=w818) -> ("error out"=w813:errorcluster)  [unwired: 7 in, 1 out]
              }
            }
            n454 = local write "error out (frontpanel screenshots)"(w806) -> ()
          }
          frame #7 {
            n455 = flat-sequence {
              tunnel: w830 -> [w833]
              tunnel: [w833] -> w829
              tunnel: w831 -> [w848]
              tunnel: w829 -> [w836]
              tunnel: [w835] -> w828
              tunnel: w827 -> [w834]
              frame #0 {
                n456 = property class="TabCtl (strict)"("Val(Sgnl)"=T1."CHF" ("Value (Signaling)")) -> ()  [unwired: 2 in, 2 out]
              }
              frame #1 {
                w846 = "_" ("string")
                n457 = local read "Cycle #"() -> (w844:u32)
                n458 = Format Value(format string="%06d", value (0)=w844) -> (output string=w843:string)  [unwired: 1 in]
                n459 = call "LV_UNIXTIME.vi"("current time"=w836) -> ("date/time string"=w847:string)  [unwired: 9 in, 1 out]
                n460 = Concatenate Strings(w834, w847, w846, w843, w846, "page8.png" ("string")) -> (w841:string)
                n461 = invoke class="TabCtl (strict)" method="Get Image"(error in=errorcluster {"status"=FALSE, "code"=0, "source"=""} ("error in (no error)")) -> (error out=w837:errorcluster, "image data"=w839:T24)  [unwired: 5 in, 4 out]
                n462 = Build Path(base path=w848, name or relative path=w841) -> (appended path=w840:path)
                n463 = call <vilib>:"Write PNG File.vi"("error in (no error)"=w837, "image data"=w839, "path to PNG file"=w840) -> ("error out"=w835:errorcluster)  [unwired: 7 in, 1 out]
              }
            }
            n464 = local write "error out (frontpanel screenshots)"(w828) -> ()
          }
          frame #8 {
            n465 = flat-sequence {
              tunnel: w852 -> [w855]
              tunnel: [w855] -> w851
              tunnel: w853 -> [w870]
              tunnel: w851 -> [w858]
              tunnel: [w857] -> w850
              tunnel: w849 -> [w856]
              frame #0 {
                n466 = property class="TabCtl (strict)"("Val(Sgnl)"=T1."(Plc. hld.)" ("Value (Signaling)")) -> ()  [unwired: 2 in, 2 out]
              }
              frame #1 {
                w868 = "_" ("string")
                n467 = local read "Cycle #"() -> (w866:u32)
                n468 = Format Value(format string="%06d", value (0)=w866) -> (output string=w865:string)  [unwired: 1 in]
                n469 = call "LV_UNIXTIME.vi"("current time"=w858) -> ("date/time string"=w869:string)  [unwired: 9 in, 1 out]
                n470 = Concatenate Strings(w856, w869, w868, w865, w868, "page8.png" ("string")) -> (w863:string)
                n471 = invoke class="TabCtl (strict)" method="Get Image"(error in=errorcluster {"status"=FALSE, "code"=0, "source"=""} ("error in (no error)")) -> (error out=w859:errorcluster, "image data"=w861:T24)  [unwired: 5 in, 4 out]
                n472 = Build Path(base path=w870, name or relative path=w863) -> (appended path=w862:path)
                n473 = call <vilib>:"Write PNG File.vi"("error in (no error)"=w859, "image data"=w861, "path to PNG file"=w862) -> ("error out"=w857:errorcluster)  [unwired: 7 in, 1 out]
              }
            }
            n474 = local write "error out (frontpanel screenshots)"(w850) -> ()
          }
          frame #9 {
            n475 = local write "Frontpanel screenshots"(FALSE ("Frontpanel screenshots")) -> ()
          }
        }
        "error out (frontpanel screenshots)" <- w669
        n476 = property class="TabCtl (strict)"("Val(Sgnl)"=w667) -> ()  [unwired: 2 in, 2 out]
      }
      event "Stop Button": Value Change {
        n477 = event-data() -> ()  [unwired: 1 in, 3 out]
      }
    }
    n478 = Wait (ms)(milliseconds to wait=u32 123) -> ()  [unwired: 1 out]
  }
  n479 = while {
    stop <- w877 stop-if-true
    n480 = event shown="[5] \"Plot selecter LSI218(1)     1      2     3     4\", \"Plot selecter LSI218(2)     1      2     3     4\", \"Plot selecter (USB6210)     1      2     3     4\", \"Plot selecter LSI336       1      2     3     4\", \"Plot selecter (USB6218)     1      2     3     4\", \"Plot selecter (HP34401A)     1      2     3     4\": Value Change" {
      selector: _ -> [_ _ _ _ _ _ _ _ _ _ _]
      dyn-events: _ -> [_ _ _ _ _ _ _ _ _ _ _]
      timeout: _ -> [_ _ _ _ _ _ _ _ _ _ _]
      tunnel: [_ _ _ _ _ _ _ _ _ _ TRUE] -> w877
      tunnel: [errorcluster {"status"=FALSE, "code"=0, "source"=""} ("error out") w881 _ _ _ _ w1017 w1034 w1051 w1068 errorcluster {"status"=FALSE, "code"=0, "source"=""} ("error out")] -> w873
      event Timeout {
        n481 = event-data() -> ()  [unwired: 1 in, 3 out]
      }
      event "log/linear 1": Value Change {
        n482 = event-data() -> ()  [unwired: 1 in, 6 out]
        n483 = flat-sequence {
          tunnel: [w882] -> w881
          frame #0 {
            n484 = Boolean To (0,1)(Boolean="log/linear 1") -> (0, 1=w887:i16)
            n485 = control-ref of="Graph 1"() -> (w883:refnum<vi>)
            n486 = property class="XYGraph (strict)"(reference=w883, error in=errorcluster {"status"=FALSE, "code"=0, "source"=""} ("error in (no error)"), "YScale.Mapping Mode"=w887) -> (error out=w885:errorcluster)  [unwired: 1 out]
            n487 = control-ref of="error out (USB6210)"() -> (w886:refnum<vi>)
            n488 = property class="Clust (strict)"(reference=w886, "Val(Sgnl)"=w885) -> (error out=w882:errorcluster)  [unwired: 1 in, 1 out]
          }
        }
      }
      event "log/linear 2": Value Change {
        n489 = event-data() -> ()  [unwired: 1 in, 6 out]
        n490 = flat-sequence {
          frame #0 {
            n491 = Boolean To (0,1)(Boolean="log/linear 2") -> (0, 1=w893:i16)
            n492 = control-ref of="Graph 2"() -> (w891:refnum<vi>)
            n493 = property class="XYGraph (strict)"(reference=w891, error in=errorcluster {"status"=FALSE, "code"=0, "source"=""} ("error in (no error)"), "YScale.Mapping Mode"=w893) -> (error out=w892:errorcluster)  [unwired: 1 out]
            n494 = control-ref of="error out (USB6210)"() -> (w890:refnum<vi>)
            n495 = property class="Clust (strict)"(reference=w890, "Value"=w892) -> ()  [unwired: 1 in, 2 out]
          }
        }
      }
      event "log/linear 3": Value Change {
        n496 = event-data() -> ()  [unwired: 1 in, 6 out]
        n497 = flat-sequence {
          frame #0 {
            n498 = Boolean To (0,1)(Boolean="log/linear 3") -> (0, 1=w899:i16)
            n499 = control-ref of="Graph 3"() -> (w895:refnum<vi>)
            n500 = property class="XYGraph (strict)"(reference=w895, error in=errorcluster {"status"=FALSE, "code"=0, "source"=""} ("error in (no error)"), "YScale.Mapping Mode"=w899) -> (error out=w898:errorcluster)  [unwired: 1 out]
            n501 = control-ref of="error out (USB6210)"() -> (w897:refnum<vi>)
            n502 = property class="Clust (strict)"(reference=w897, "Value"=w898) -> ()  [unwired: 1 in, 2 out]
          }
        }
      }
      event "log/linear 4": Value Change {
        n503 = event-data() -> ()  [unwired: 1 in, 6 out]
        n504 = flat-sequence {
          frame #0 {
            n505 = Boolean To (0,1)(Boolean="log/linear 4") -> (0, 1=w905:i16)
            n506 = control-ref of="Graph 4"() -> (w901:refnum<vi>)
            n507 = property class="XYGraph (strict)"(reference=w901, error in=errorcluster {"status"=FALSE, "code"=0, "source"=""} ("error in (no error)"), "YScale.Mapping Mode"=w905) -> (error out=w904:errorcluster)  [unwired: 1 out]
            n508 = control-ref of="error out (USB6210)"() -> (w903:refnum<vi>)
            n509 = property class="Clust (strict)"(reference=w903, "Value"=w904) -> ()  [unwired: 1 in, 2 out]
          }
        }
      }
      event "Plot selecter LSI218(1)\n    1      2     3     4", "Plot selecter LSI218(2)\n    1      2     3     4", "Plot selecter (USB6210)\n    1      2     3     4", "Plot selecter LSI336 \n     1      2     3     4", "Plot selecter (USB6218)\n    1      2     3     4", "Plot selecter (HP34401A)\n    1      2     3     4": Value Change {
        n510 = event-data() -> ()  [unwired: 1 in, 6 out]
        n511 = local read "Labels (HP34401 LM)"() -> (w912:string[])
        n512 = call "BuildPlotLegends.vi"("Plot selecter \n    1      2     3     4"="Plot selecter (HP34401A)\n    1      2     3     4", "AllLabels"=w912) -> ("Series 4"=w907:string[], "Series 3"=w908:string[], "Series 2"=w909:string[], "Series 1"=w910:string[])  [unwired: 6 in]
        n513 = local read "All Labels (USB6210)"() -> (w929:string[])
        n514 = local read "All Labels (USB6218)"() -> (w918:string[])
        n515 = local read "Labels LSI218 (1)"() -> (w931:string[])
        n516 = local read "Labels LSI218 (2)"() -> (w932:string[])
        n517 = local read "Labels LSI336"() -> (w924:string[])
        n518 = call "BuildPlotLegends_LSI218.vi"("Plot selecter (2)\n    1      2     3     5"="Plot selecter LSI218(2)\n    1      2     3     4", "Plot selecter (1)\n    1      2     3     4"="Plot selecter LSI218(1)\n    1      2     3     4", "Labels (2)"=w932, "Labels (1)"=w931) -> ("Series 4"=w942:string[], "Series 3"=w940:string[], "Series 2"=w938:string[], "Series 1"=w936:string[])  [unwired: 4 in]
        n519 = call "BuildPlotLegends.vi"("Plot selecter \n    1      2     3     4"="Plot selecter (USB6210)\n    1      2     3     4", "AllLabels"=w929) -> ("Series 4"=w941:string[], "Series 3"=w939:string[], "Series 2"=w937:string[], "Series 1"=w935:string[])  [unwired: 6 in]
        n520 = call "BuildPlotLegends.vi"("Plot selecter \n    1      2     3     4"="Plot selecter LSI336 \n     1      2     3     4", "AllLabels"=w924) -> ("Series 4"=w919:string[], "Series 3"=w920:string[], "Series 2"=w921:string[], "Series 1"=w922:string[])  [unwired: 6 in]
        n521 = call "BuildPlotLegends.vi"("Plot selecter \n    1      2     3     4"="Plot selecter (USB6218)\n    1      2     3     4", "AllLabels"=w918) -> ("Series 4"=w914:string[], "Series 3"=w913:string[], "Series 2"=w915:string[], "Series 1"=w916:string[])  [unwired: 6 in]
        n522 = Build Array (concatenate)(w937, w938, w921, w915, w909) -> (w926:string[])
        "Series 2" <- w926
        n523 = Build Array (concatenate)(w939, w940, w920, w913, w908) -> (w927:string[])
        "Series 3" <- w927
        n524 = Build Array (concatenate)(w941, w942, w919, w914, w907) -> (w928:string[])
        "Series 4" <- w928
        n525 = Build Array (concatenate)(w935, w936, w922, w916, w910) -> (w925:string[])
        "Series 1" <- w925
        n526 = stacked-sequence {
          tunnel: [w952 _ _ _] -> w946
          tunnel: [_ w970 _ _] -> w947
          tunnel: [_ _ w987 _] -> w945
          tunnel: [_ _ _ w1004] -> w944
          tunnel: w925 -> [w950 _ _ _]
          tunnel: w926 -> [_ w968 _ _]
          tunnel: w927 -> [_ _ w985 _]
          tunnel: w928 -> [_ _ _ w1002]
          frame #0 {
            n527 = Array Size(array=w950) -> (size(s)=w954:i32)
            n528 = control-ref of="Graph 1"() -> (w948:refnum<vi>)
            n529 = property class="XYGraph (strict)"(reference=w948) -> ("LegNumRows"=w949:u32)  [unwired: 1 in, 2 out]
            n530 = for {
              N: w949 -> [_]
              tunnel: w948 -> [w963]
              shift-right: [w961] -> w953
              shift-left: errorcluster {"status"=FALSE, "code"=0, "source"=""} ("error in (no error)") -> [w962]
              i -> [w965]
              n531 = property class="XYGraph (strict)"(reference=w963, error in=w962, "Active Plot"=w965, "Plot.Plot Name"="") -> (error out=w961:errorcluster)  [unwired: 1 out]
            }
            n532 = for {
              N: w954 -> [_]
              tunnel: w948 -> [w959]
              shift-right: [w957] -> w952
              shift-left: w953 -> [w958]
              tunnel: w950 -> [w956] mode=indexing
              i -> [w960]
              n533 = property class="XYGraph (strict)"(reference=w959, error in=w958, "Active Plot"=w960, "Plot.Plot Name"=w956, "Plot.Visible?"=TRUE ("Plot.Visible")) -> (error out=w957:errorcluster)  [unwired: 1 out]
            }
          }
          frame #1 {
            n534 = Array Size(array=w968) -> (size(s)=w972:i32)
            n535 = control-ref of="Graph 2"() -> (w967:refnum<vi>)
            n536 = property class="XYGraph (strict)"(reference=w967) -> ("LegNumRows"=w966:u32)  [unwired: 1 in, 2 out]
            n537 = for {
              N: w966 -> [_]
              shift-right: [w979] -> w971
              shift-left: errorcluster {"status"=FALSE, "code"=0, "source"=""} ("error in (no error)") -> [w980]
              tunnel: w967 -> [w978]
              i -> [w982]
              n538 = property class="XYGraph (strict)"(reference=w978, error in=w980, "Active Plot"=w982, "Plot.Plot Name"="") -> (error out=w979:errorcluster)  [unwired: 1 out]
            }
            n539 = for {
              N: w972 -> [_]
              shift-right: [w975] -> w970
              shift-left: w971 -> [w976]
              tunnel: w968 -> [w974] mode=indexing
              tunnel: w967 -> [w973]
              i -> [w977]
              n540 = property class="XYGraph (strict)"(reference=w973, error in=w976, "Active Plot"=w977, "Plot.Plot Name"=w974) -> (error out=w975:errorcluster)  [unwired: 1 out]
            }
          }
          frame #2 {
            n541 = Array Size(array=w985) -> (size(s)=w989:i32)
            n542 = control-ref of="Graph 3"() -> (w983:refnum<vi>)
            n543 = property class="XYGraph (strict)"(reference=w983) -> ("LegNumRows"=w984:u32)  [unwired: 1 in, 2 out]
            n544 = for {
              N: w984 -> [_]
              tunnel: w983 -> [w997]
              shift-right: [w995] -> w988
              shift-left: errorcluster {"status"=FALSE, "code"=0, "source"=""} ("error in (no error)") -> [w996]
              i -> [w999]
              n545 = property class="XYGraph (strict)"(reference=w997, error in=w996, "Active Plot"=w999, "Plot.Plot Name"="") -> (error out=w995:errorcluster)  [unwired: 1 out]
            }
            n546 = for {
              N: w989 -> [_]
              tunnel: w983 -> [w993]
              shift-right: [w991] -> w987
              shift-left: w988 -> [w992]
              tunnel: w985 -> [w990] mode=indexing
              i -> [w994]
              n547 = property class="XYGraph (strict)"(reference=w993, error in=w992, "Active Plot"=w994, "Plot.Plot Name"=w990) -> (error out=w991:errorcluster)  [unwired: 1 out]
            }
          }
          frame #3 {
            n548 = Array Size(array=w1002) -> (size(s)=w1006:i32)
            n549 = control-ref of="Graph 4"() -> (w1000:refnum<vi>)
            n550 = property class="XYGraph (strict)"(reference=w1000) -> ("LegNumRows"=w1001:u32)  [unwired: 1 in, 2 out]
            n551 = for {
              N: w1001 -> [_]
              tunnel: w1000 -> [w1014]
              shift-right: [w1012] -> w1005
              shift-left: errorcluster {"status"=FALSE, "code"=0, "source"=""} ("error in (no error)") -> [w1013]
              i -> [w1016]
              n552 = property class="XYGraph (strict)"(reference=w1014, error in=w1013, "Active Plot"=w1016, "Plot.Plot Name"="") -> (error out=w1012:errorcluster)  [unwired: 1 out]
            }
            n553 = for {
              N: w1006 -> [_]
              tunnel: w1000 -> [w1010]
              shift-right: [w1008] -> w1004
              shift-left: w1005 -> [w1009]
              tunnel: w1002 -> [w1007] mode=indexing
              i -> [w1011]
              n554 = property class="XYGraph (strict)"(reference=w1010, error in=w1009, "Active Plot"=w1011, "Plot.Plot Name"=w1007) -> (error out=w1008:errorcluster)  [unwired: 1 out]
            }
          }
        }
        n555 = Merge Errors(w946, w947, w945, w944) -> (→"Plot errors":errorcluster)
      }
      event "Take Screenshot! 1": Value Change {
        n556 = event-data() -> ()  [unwired: 1 in, 6 out]
        n557 = flat-sequence {
          tunnel: [w1018] -> w1017
          frame #0 {
            n558 = flat-sequence {
              tunnel: [w1019] -> w1018
              frame #0 {
                w1028 = "_" ("string")
                n559 = Get Date/Time In Seconds() -> (seconds since 1Jan1904=w1025:timestamp)
                n560 = local read "RUN Identifier"() -> (w1030:string)
                n561 = call "LV_UNIXTIME.vi"("current time"=w1025) -> ("date/time string"=w1029:string)  [unwired: 9 in, 1 out]
                n562 = control-ref of="Graph 1"() -> (w1024:refnum<vi>)
                n563 = Concatenate Strings(w1030, w1028, w1029, w1028, "FIle suffix 1", ".png" ("string")) -> (w1032:string)
                n564 = local read "Base Path"() -> (w1031:path)
                n565 = invoke class="XYGraph (strict)" method="Get Image"(reference=w1024, error in=errorcluster {"status"=FALSE, "code"=0, "source"=""} ("error in (no error)")) -> (error out=w1020:errorcluster, "image data"=w1023:T24)  [unwired: 4 in, 4 out]
                n566 = Build Path(base path=w1031, name or relative path=w1032) -> (appended path=w1022:path)
                n567 = call <vilib>:"Write PNG File.vi"("error in (no error)"=w1020, "image data"=w1023, "path to PNG file"=w1022) -> ("error out"=w1019:errorcluster)  [unwired: 7 in, 1 out]
              }
              frame #1 {
                n568 = local write "Take Screenshot! 1"(FALSE ("Take Screenshot! 1")) -> ()
              }
            }
          }
        }
      }
      event "Take Screenshot! 2": Value Change {
        n569 = event-data() -> ()  [unwired: 1 in, 6 out]
        n570 = flat-sequence {
          tunnel: [w1035] -> w1034
          frame #0 {
            n571 = flat-sequence {
              tunnel: [w1041] -> w1035
              frame #0 {
                w1045 = "_" ("string")
                n572 = Get Date/Time In Seconds() -> (seconds since 1Jan1904=w1042:timestamp)
                n573 = local read "RUN Identifier"() -> (w1047:string)
                n574 = call "LV_UNIXTIME.vi"("current time"=w1042) -> ("date/time string"=w1046:string)  [unwired: 9 in, 1 out]
                n575 = control-ref of="Graph 2"() -> (w1036:refnum<vi>)
                n576 = Concatenate Strings(w1047, w1045, w1046, w1045, "FIle suffix 2", ".png" ("string")) -> (w1049:string)
                n577 = local read "Base Path"() -> (w1048:path)
                n578 = invoke class="XYGraph (strict)" method="Get Image"(reference=w1036, error in=errorcluster {"status"=FALSE, "code"=0, "source"=""} ("error in (no error)")) -> (error out=w1040:errorcluster, "image data"=w1038:T24)  [unwired: 4 in, 4 out]
                n579 = Build Path(base path=w1048, name or relative path=w1049) -> (appended path=w1037:path)
                n580 = call <vilib>:"Write PNG File.vi"("error in (no error)"=w1040, "image data"=w1038, "path to PNG file"=w1037) -> ("error out"=w1041:errorcluster)  [unwired: 7 in, 1 out]
              }
              frame #1 {
                n581 = local write "Take Screenshot! 2"(FALSE ("Take Screenshot! 1")) -> ()
              }
            }
          }
        }
      }
      event "Take Screenshot! 3": Value Change {
        n582 = event-data() -> ()  [unwired: 1 in, 6 out]
        n583 = flat-sequence {
          tunnel: [w1052] -> w1051
          frame #0 {
            n584 = flat-sequence {
              tunnel: [w1054] -> w1052
              frame #0 {
                w1062 = "_" ("string")
                n585 = Get Date/Time In Seconds() -> (seconds since 1Jan1904=w1060:timestamp)
                n586 = local read "RUN Identifier"() -> (w1064:string)
                n587 = call "LV_UNIXTIME.vi"("current time"=w1060) -> ("date/time string"=w1063:string)  [unwired: 9 in, 1 out]
                n588 = control-ref of="Graph 3"() -> (w1057:refnum<vi>)
                n589 = Concatenate Strings(w1064, w1062, w1063, w1062, "FIle suffix 3", ".png" ("string")) -> (w1066:string)
                n590 = local read "Base Path"() -> (w1065:path)
                n591 = invoke class="XYGraph (strict)" method="Get Image"(reference=w1057, error in=errorcluster {"status"=FALSE, "code"=0, "source"=""} ("error in (no error)")) -> (error out=w1055:errorcluster, "image data"=w1053:T24)  [unwired: 4 in, 4 out]
                n592 = Build Path(base path=w1065, name or relative path=w1066) -> (appended path=w1058:path)
                n593 = call <vilib>:"Write PNG File.vi"("error in (no error)"=w1055, "image data"=w1053, "path to PNG file"=w1058) -> ("error out"=w1054:errorcluster)  [unwired: 7 in, 1 out]
              }
              frame #1 {
                n594 = local write "Take Screenshot! 3"(FALSE ("Take Screenshot! 1")) -> ()
              }
            }
          }
        }
      }
      event "Take Screenshot! 4": Value Change {
        n595 = event-data() -> ()  [unwired: 1 in, 6 out]
        n596 = flat-sequence {
          tunnel: [w1069] -> w1068
          frame #0 {
            n597 = flat-sequence {
              tunnel: [w1072] -> w1069
              frame #0 {
                w1079 = "_" ("string")
                n598 = Get Date/Time In Seconds() -> (seconds since 1Jan1904=w1077:timestamp)
                n599 = local read "RUN Identifier"() -> (w1081:string)
                n600 = call "LV_UNIXTIME.vi"("current time"=w1077) -> ("date/time string"=w1080:string)  [unwired: 9 in, 1 out]
                n601 = control-ref of="Graph 4"() -> (w1073:refnum<vi>)
                n602 = Concatenate Strings(w1081, w1079, w1080, w1079, "FIle suffix 4", ".png" ("string")) -> (w1083:string)
                n603 = local read "Base Path"() -> (w1082:path)
                n604 = invoke class="XYGraph (strict)" method="Get Image"(reference=w1073, error in=errorcluster {"status"=FALSE, "code"=0, "source"=""} ("error in (no error)")) -> (error out=w1070:errorcluster, "image data"=w1074:T24)  [unwired: 4 in, 4 out]
                n605 = Build Path(base path=w1082, name or relative path=w1083) -> (appended path=w1075:path)
                n606 = call <vilib>:"Write PNG File.vi"("error in (no error)"=w1070, "image data"=w1074, "path to PNG file"=w1075) -> ("error out"=w1072:errorcluster)  [unwired: 7 in, 1 out]
              }
              frame #1 {
                n607 = local write "Take Screenshot! 4"(FALSE ("Take Screenshot! 1")) -> ()
              }
            }
          }
        }
      }
      event "Stop Button": Value Change {
        n608 = event-data() -> ()  [unwired: 1 in, 6 out]
      }
    }
    "error out (graph operations)" <- w873
    n609 = local write "Take Screenshot! 1"(FALSE ("Take Screenshot! 1")) -> ()
    n610 = local write "Take Screenshot! 2"(FALSE ("Take Screenshot! 1")) -> ()
    n611 = Wait (ms)(milliseconds to wait=u32 1000) -> ()  [unwired: 1 out]
    n612 = local write "Take Screenshot! 3"(FALSE ("Take Screenshot! 1")) -> ()
    n613 = local write "Take Screenshot! 4"(FALSE ("Take Screenshot! 1")) -> ()
  }
  n614 = while {
    i -> [w1091]
    stop <- w1088 stop-if-true
    n615 = Equal?(x=w1091, y=0) -> (x = y?=w1089:bool)
    n616 = case shown="True" w1089 {
      frame False {
      }
      frame True {
        (unwired) FALSE ("Value (Signaling)")
      }
    }
    n617 = Wait (ms)(milliseconds to wait=u32 123) -> ()  [unwired: 1 out]
    n618 = event shown="[5] \"Kikusui I (mA)\", \"I_lim_up (mA)\", \"I_lim_low (mA)\", \"OUTPUT  Kikusui\": Value Change" {
      selector: _ -> [_ _ _ _ _ _]
      dyn-events: _ -> [_ _ _ _ _ _]
      timeout: _ -> [_ _ _ _ _ _]
      tunnel: [FALSE ("Value (Signaling)") TRUE ("Value (Signaling)") _ FALSE ("Value (Signaling)") _ _] -> w1088
      tunnel: "VISA (Agilent 34402)" -> [_ _ w1097 w1101 _ _]
      event "CHF power supply selection": Value Change {
        n619 = event-data() -> ()  [unwired: 1 in, 3 out]
        n620 = Boolean To (0,1)(Boolean="CHF power supply selection") -> (0, 1=w1094:i16)
        n621 = property on="Tab Control 4" class="TabCtl (strict)"("Val(Sgnl)"=w1094) -> ()  [unwired: 2 in, 2 out]
      }
      event "Stop Button": Value Change {
        n622 = event-data() -> ()  [unwired: 1 in, 3 out]
      }
      event "Initialize (Agilent)": Value Change {
        n623 = event-data() -> ()  [unwired: 1 in, 3 out]
        n624 = call "Initialize.vi"("error in (no error)"=errorcluster {"status"=FALSE, "code"=0, "source"=""}, "VISA resource name"=w1097) -> ("error out"=→"error out (Agilent)":errorcluster)  [unwired: 8 in, 1 out]
        n625 = property on="Agilent\nIntialized?" class="Bool (strict)"("Val(Sgnl)"=TRUE ("Value (Signaling)")) -> ()  [unwired: 2 in, 2 out]
      }
      event "Kenwood set V (V)", "OUTPUT \nKenwood": Value Change {
        n626 = local read "Agilent\nIntialized?"() -> (w1103:bool)
        n627 = event-data() -> ()  [unwired: 1 in, 3 out]
        n628 = case shown="True" w1103 {
          tunnel: w1101 -> [_ w1104]
          frame False {
          }
          frame True {
            w1111 = u16 0 items=["DC", "Sine", "Square", "Triangle", "Ramp", "Pulse", "Noise", "Sinc", "Negative Ramp", "Exponential Rise", "Exponential Fall", "Cardiac"] ("Waveform Function (1: Sine)")
            n629 = xnode "Formula"("X1"="Kenwood set V (V)") -> ("Result"=w1108:dbl)  [unwired: 1 in, 1 out]
            n630 = call "Configure Standard Waveform.vi"("DC Offset (0.00 V)"=w1108, "Frequency (1000 Hz)"=1.0, "error in (no error)"=errorcluster {"status"=FALSE, "code"=0, "source"=""}, "Amplitude (1)"=1.0, "Waveform Function (1: Sine)"=w1111, "VISA resource name"=w1104) -> ("error out"=w1113:errorcluster, "VISA resource name out"=w1114:refnum<visa-resource-name>)  [unwired: 4 in]
            n631 = call "Enable Output.vi"("error in (no error)"=w1113, "Enable Output  (T: Enable)"="OUTPUT \nKenwood", "VISA resource name"=w1114) -> ("error out"=w1107:errorcluster)  [unwired: 7 in, 1 out]
            n632 = local write "error out (Agilent)"(w1107) -> ()
          }
        }
      }
      event "V_lim_low (V)", "V_lim_up (V)": Value Change {
        n633 = event-data() -> ()  [unwired: 1 in, 3 out]
        n634 = property on="Kenwood set V (V)" class="DigNum (strict)"("Minimum"="V_lim_low (V)", "Maximum"="V_lim_up (V)") -> ()  [unwired: 2 in, 2 out]
      }
      event "Kikusui I (mA)", "I_lim_up (mA)", "I_lim_low (mA)", "OUTPUT \nKikusui": Value Change {
        n635 = event-data() -> ()  [unwired: 1 in, 3 out]
        n636 = property on="OUTPUT\n(PWR)" class="Bool (strict)"("Val(Sgnl)"="OUTPUT \nKikusui") -> ()  [unwired: 2 in, 2 out]
        n637 = property on="upper limit (mA)\n (PWR)" class="DigNum (strict)"("Val(Sgnl)"="I_lim_low (mA)") -> ()  [unwired: 2 in, 2 out]
        n638 = property on="upper limit (mA)\n (PWR)" class="DigNum (strict)"("Val(Sgnl)"="I_lim_up (mA)") -> ()  [unwired: 2 in, 2 out]
        n639 = property on="Set Current (mA)\n (PWR)" class="DigNum (strict)"("Val(Sgnl)"="Kikusui I (mA)") -> ()  [unwired: 2 in, 2 out]
      }
    }
  }
  n640 = while {
    stop <- w1129 stop-if-true
    n641 = Wait (ms)(milliseconds to wait=u32 101) -> ()  [unwired: 1 out]
    n642 = event shown="[0] \"Initialize (DMMs)\": Value Change" {
      selector: _ -> [_ _ _]
      dyn-events: _ -> [_ _ _]
      timeout: _ -> [_ _ _]
      tunnel: [FALSE TRUE FALSE] -> w1129
      event "Initialize (DMMs)": Value Change {
        w1132 = T4 [] ("Value (Signaling)")
        n643 = event-data() -> ()  [unwired: 1 in, 3 out]
        n644 = property on="Graph DMMs 1" class="XYGraph (strict)"("Val(Sgnl)"=w1132) -> ()  [unwired: 2 in, 2 out]
        n645 = property on="Graph DMMs 2" class="XYGraph (strict)"("Val(Sgnl)"=w1132) -> ()  [unwired: 2 in, 2 out]
      }
      event "Stop Button": Value Change {
        n646 = event-data() -> ()  [unwired: 1 in, 3 out]
      }
      event Timeout {
        n647 = event-data() -> ()  [unwired: 1 in, 3 out]
      }
    }
  }
  n648 = Obtain Notifier(name (unnamed)="stop notifier", notification data type=w17, create if not found? (T)=w17, error in (no error)=errorcluster {"status"=FALSE, "code"=0, "source"=""}) -> (notifier out=w5:refnum<notifier>, error out=w4:errorcluster)  [unwired: 1 out]
  n649 = while {
    shift-right: [w1245] -> w40
    shift-left: refnum<class "USBData.lvclass"> refnum ("USBData.lvclass") -> [w1248]
    shift-right: [w1241] -> w39
    shift-left: w6 -> [w1247]
    tunnel: "Base Path" -> [w1147]
    shift-right: [w1223] -> w34
    shift-left: errorcluster {"status"=FALSE, "code"=0, "source"=""} ("error in (no error)") -> [w1239]
    shift-right: [w1224] -> w35
    shift-left: refnum<class "LSI218Data.lvclass"> refnum ("LSI218Data.lvclass") -> [w1238]
    shift-right: [w1211] -> w31
    shift-left: refnum<class "LSI336Data.lvclass"> refnum ("LSI336Data.lvclass") -> [w1220]
    shift-right: [w1210] -> w30
    shift-left: w21 -> [w1219]
    shift-right: [w1199] -> _
    shift-left: w6 -> [w1200]
    shift-right: [w1189] -> w25
    shift-left: refnum<class "USBData.lvclass"> refnum ("USBData.lvclass") -> [w1197]
    shift-right: [w1188] -> w24
    shift-left: errorcluster {"status"=FALSE, "code"=0, "source"=""} ("error in (no error)") -> [w1196]
    shift-right: [w1185] -> _
    shift-left: w21 -> [w1184]
    tunnel: w5 -> [w1155]
    tunnel: w4 -> [w1154]
    tunnel: [w1152] -> w13
    tunnel: [w1151] -> w12
    shift-right: [w1148] -> _
    shift-left: refnum<class "LMData.lvclass"> refnum ("LMData in") -> [w1149]
    shift-right: [w1145] -> _
    shift-left: errorcluster {"status"=FALSE, "code"=0, "source"=""} ("error in (no error)") -> [w1146]
    i -> [w1144]
    stop <- "Stop Button" stop-if-true
    w1140 = T26 [] ("appended array")
    w1206 = u32 24 ("Number of Rows")
    w1216 = T26 [] ("appended array")
    w1233 = T26 [] ("appended array")
    n650 = local read "LSI218Settings(A-F)"() -> (w1176:T3)
    n651 = control-ref of="Plot selecter LSI218(2)\n    1      2     3     4"() -> (w1204:refnum<vi>)
    n652 = control-ref of="Plot selecter LSI218(1)\n    1      2     3     4"() -> (w1205:refnum<vi>)
    n653 = control-ref of="Plot selecter LSI336 \n     1      2     3     4"() -> (w1203:refnum<vi>)
    n654 = property on="Property Node" class="Arr (strict)"(reference=w1204, "Number of Rows"=w1206) -> ()  [unwired: 1 in, 2 out]
    n655 = property on="Property Node" class="Arr (strict)"(reference=w1205, "Number of Rows"=w1206) -> ()  [unwired: 1 in, 2 out]
    n656 = local read "LSI336Settings(X,Y)"() -> (w1174:T3)
    n657 = Array Size(array=w1176) -> (size(s)=w1175:i32)
    n658 = property on="Property Node" class="Arr (strict)"(reference=w1203, "Number of Rows"=u32 8) -> ()  [unwired: 1 in, 2 out]
    n659 = Multiply(x="Measurement Interval (s)", y=u32 1000) -> (x*y=w1242:dbl)
    n660 = Wait (ms)(milliseconds to wait=w1242) -> ()  [unwired: 1 out]
    n661 = for {
      N: w1175 -> [_]
      tunnel: w1176 -> [w1336] mode=indexing
      tunnel: [w1335] -> w1172 mode=concatenating
      n662 = Unbundle By Name(w1336) -> ("SensorLocations"=w1335:T19)
    }
    n663 = for {
      tunnel: w1174 -> [w1334] mode=indexing
      tunnel: [w1333] -> w1173 mode=concatenating
      n664 = Unbundle By Name(w1334) -> ("SensorLocations"=w1333:T19)
    }
    n665 = Quotient & Remainder(x=w1144, y="Screenshots interval") -> (x-y*floor(x/y)=w1160:i64)  [unwired: 1 out]
    n666 = Equal?(x=w1144, y=0) -> (x = y?=w1150:bool)
    n667 = case shown="True" w1150 {
      tunnel: w1248 -> [w2399 w2422]
      tunnel: w1247 -> [w2393 w2420]
      tunnel: w1144 -> [w2384 _]
      tunnel: [w2391 w2417] -> w1241
      tunnel: [w2388 w2416] -> w1198
      tunnel: [w2389 w2415] -> w1245
      tunnel: [w2379 w2410] -> w1246
      tunnel: w1147 -> [_ w2409]
      tunnel: [w2378 w2406] -> w1181
      frame False {
        n668 = call-dynamic "USBData_measure.vi"("USBData in"=w2399, "DAQ sample #"=i64 5, "DAQ timeout"=100.0 ("DAQ timeout (def: 100)"), "MeasurementIndex"=w2384, "error in (no error)"=w2393, "save every ... measurements"="Record interval") -> ("USBData out"=w2398:refnum<class "USBData.lvclass">, "TimeMeasuremeent"=w2395:timestamp, "Status"=→"USB6210 Status":T6, "LastDataAcquired"=w2380:dbl[], "error out"=w2394:errorcluster)  [unwired: 3 in, 2 out]
        "Time of Last Measurement (USB6210)" <- w2395
        "Last Vol\n(USB6210)" <- w2380
        n669 = call-dynamic "USBData_convert.vi"("Save every ... measurements"="Record interval", "MeasurementIndex"=w2384, "error in (no error)"=w2394, "LastDataAcquired"=w2380, "TimeMeasuremeent"=w2395, "USBData in"=w2398) -> ("error out"=w2392:errorcluster, "LeakDet_FULL"=w2387:dbl, "LastDataConverted"=w2381:dbl[], "USBData out"=w2390:refnum<class "USBData.lvclass">)  [unwired: 2 in]
        n670 = call "USBData_read.vi"("USBData in"=w2390, "error in (no error)"=w2392) -> ("Status"=w2382:T6, "USBData out"=w2389:refnum<class "USBData.lvclass">, "Data"=w2388:T27, "Basic"=w2379:T28, "error out"=w2391:errorcluster)  [unwired: 2 in, 2 out]
        n671 = local write "USB6210 Status"(w2382) -> ()
        n672 = Unbundle By Name(w2379) -> ("ReadLeakDet?"=w2386:bool)
        n673 = Unbundle By Name(w2379) -> ("Labels"=w2378:string[])
        n674 = case shown="False" w2386 {
          tunnel: w2381 -> [w2400 w2403]
          tunnel: w2387 -> [_ w2402]
          tunnel: [w2400 w2401] -> w2385
          frame False {
          }
          frame True {
            n675 = Build Array (concatenate)(w2403, w2402) -> (w2401:dbl[])
          }
        }
        "Last Data \n(USB6210)" <- w2385
      }
      frame True {
        n676 = local read "RUN Identifier"() -> (w2404:string)
        n677 = call-dynamic "USBData_initialize.vi"("USBData in"=w2422, "SeriesSetting"="USB6210 Config", "BasePath"=w2409, "RunIdentifier"=w2404, "FileName"="InstName (USB6210)", "error in (no error)"=w2420) -> ("Status"=w2405:T6, "USBData out"=w2418:refnum<class "USBData.lvclass">, "error out"=w2419:errorcluster)  [unwired: 5 in, 2 out]
        n678 = local write "USB6210 Status"(w2405) -> ()
        n679 = call "USBData_read.vi"("USBData in"=w2418, "error in (no error)"=w2419) -> ("Status"=w2408:T6, "USBData out"=w2415:refnum<class "USBData.lvclass">, "Data"=w2416:T27, "Basic"=w2410:T28, "error out"=w2417:errorcluster)  [unwired: 2 in, 2 out]
        n680 = local write "USB6210 Status"(w2408) -> ()
        n681 = Unbundle By Name(w2410) -> ("ReadLeakDet?"=w2414:bool, "Labels"=w2406:string[])
        n682 = Array Size(array=w2406) -> (size(s)=w2413:i32)
        n683 = case shown="True" w2414 {
          tunnel: w2413 -> [w2423 w2425]
          tunnel: [w2423 w2424] -> w2411
          frame False {
          }
          frame True {
            n684 = Add(x=w2425, y=1) -> (x+y=w2424:i32)
          }
        }
        n685 = Initialize Array(TRUE ("Activate 2"), w2411) -> ()  [unwired: 1 out]
      }
    }
    "error out (USB6210)" <- w1241
    n686 = case shown="False" w1150 {
      tunnel: [w1917 w1944] -> w1188
      tunnel: [w1914 w1943] -> w1195
      tunnel: [w1915 w1942] -> w1189
      tunnel: [w1906 w1937] -> w1194
      tunnel: [w1905 w1935] -> _
      tunnel: w1197 -> [w1904 w1933]
      tunnel: w1147 -> [_ w1932]
      tunnel: w1196 -> [w1903 w1931]
      tunnel: w1144 -> [w1902 _]
      frame False {
        n687 = local read "Record interval"() -> (w1901:i64)
        n688 = call-dynamic "USBData_measure.vi"("USBData in"=w1904, "DAQ sample #"=i64 5, "DAQ timeout"=100.0 ("DAQ timeout (def: 100)"), "MeasurementIndex"=w1902, "error in (no error)"=w1903, "save every ... measurements"=w1901) -> ("USBData out"=w1923:refnum<class "USBData.lvclass">, "TimeMeasuremeent"=w1920:timestamp, "Status"=→"USB6218 Status":T6, "LastDataAcquired"=w1907:dbl[], "error out"=w1919:errorcluster)  [unwired: 3 in, 2 out]
        "Time of Last Measurement (USB6218)" <- w1920
        "Last Vol \n(USB6218)" <- w1907
        n689 = call-dynamic "USBData_convert.vi"("Save every ... measurements"=w1901, "MeasurementIndex"=w1902, "error in (no error)"=w1919, "LastDataAcquired"=w1907, "TimeMeasuremeent"=w1920, "USBData in"=w1923) -> ("error out"=w1918:errorcluster, "LeakDet_FULL"=w1913:dbl, "LastDataConverted"=w1908:dbl[], "USBData out"=w1916:refnum<class "USBData.lvclass">)  [unwired: 2 in]
        n690 = call "USBData_read.vi"("USBData in"=w1916, "error in (no error)"=w1918) -> ("Status"=w1909:T6, "USBData out"=w1915:refnum<class "USBData.lvclass">, "Data"=w1914:T27, "Basic"=w1906:T28, "error out"=w1917:errorcluster)  [unwired: 2 in, 2 out]
        n691 = local write "USB6218 Status"(w1909) -> ()
        n692 = Unbundle By Name(w1906) -> ("ReadLeakDet?"=w1912:bool)
        n693 = Unbundle By Name(w1906) -> ("Labels"=w1905:string[])
        n694 = case shown="True" w1912 {
          tunnel: w1908 -> [w1924 w1927]
          tunnel: w1913 -> [_ w1926]
          tunnel: [w1924 w1925] -> w1911
          frame False {
          }
          frame True {
            n695 = Build Array (concatenate)(w1927, w1926) -> (w1925:dbl[])
          }
        }
        "Last Data \n(USB6218)" <- w1911
      }
      frame True {
        n696 = local read "RUN Identifier"() -> (w1928:string)
        n697 = call-dynamic "USBData_initialize.vi"("USBData in"=w1933, "SeriesSetting"="USB6218 Config", "BasePath"=w1932, "RunIdentifier"=w1928, "FileName"="InstName (USB6218)", "error in (no error)"=w1931) -> ("Status"=w1929:T6, "USBData out"=w1945:refnum<class "USBData.lvclass">, "error out"=w1946:errorcluster)  [unwired: 5 in, 2 out]
        n698 = local write "USB6218 Status"(w1929) -> ()
        n699 = call "USBData_read.vi"("USBData in"=w1945, "error in (no error)"=w1946) -> ("Status"=w1936:T6, "USBData out"=w1942:refnum<class "USBData.lvclass">, "Data"=w1943:T27, "Basic"=w1937:T28, "error out"=w1944:errorcluster)  [unwired: 2 in, 2 out]
        n700 = local write "USB6218 Status"(w1936) -> ()
        n701 = Unbundle By Name(w1937) -> ("ReadLeakDet?"=w1941:bool, "Labels"=w1935:string[])
        n702 = Array Size(array=w1935) -> (size(s)=w1940:i32)
        n703 = case shown="True" w1941 {
          tunnel: w1940 -> [w1947 w1949]
          tunnel: [w1947 w1948] -> w1938
          frame False {
          }
          frame True {
            n704 = Add(x=w1949, y=1) -> (x+y=w1948:i32)
          }
        }
        n705 = Initialize Array(TRUE ("Activate 2"), w1938) -> ()  [unwired: 1 out]
      }
    }
    "error out (USB6218)" <- w1188
    n706 = case shown="False" w1150 {
      frame False {
      }
      frame True {
        n707 = local read "RUN label"() -> (w1327:string)
        n708 = Get Date/Time In Seconds() -> (seconds since 1Jan1904=w1331:timestamp)
        n709 = call "LV_UNIXTIME.vi"("current time"=w1331) -> ("date/time string"=w1330:string)  [unwired: 9 in, 1 out]
        n710 = Concatenate Strings(w1330, "_" ("string"), w1327) -> (→"RUN Identifier" →"RUN Identifier 2" →"RUN Identifier 3" →"RUN Identifier 4" →"RUN Identifier 5" →"RUN Identifier 6" →"RUN Identifier 7":string)
      }
    }
    n711 = Equal?(x=w1160, y=i64 0) -> (x = y?=w1157:bool)
    n712 = local read "LastData (LSI218)"() -> (w1170:dbl[])
    n713 = local read "Last Data \nLSI336"() -> (w1169:dbl[])
    n714 = And(x="Analog Out ON?", y=w1150) -> (x .and. y?=w1186:bool)
    n715 = And(x=w1157, y="Automatic \nScreenshots?") -> (x .and. y?=w1156:bool)
    n716 = Build Array (concatenate)(w1170, w1169) -> (w1168:dbl[])
    "AllTemperatures" <- w1168
    n717 = Build Array (concatenate)(w1172, w1173) -> (w1171:T19)
    "TempSensorsLocations" <- w1171
    n718 = case shown="True" w1186 {
      tunnel: w1147 -> [_ w1720]
      tunnel: [w1696 w1711] -> w1185
      tunnel: w1184 -> [w1696 w1710]
      frame False {
      }
      frame True {
        w1703 = "_raw" ("string")
        w1727 = 10.0 ("V_lim_max")
        w1726 = 0.0 ("V_lim_min")
        w1725 = -1 items=["Default"=-1, "RSE"=10083, "Differential"=10106, "Pseudodifferential"=12529] ("output terminal configuration")
        w1724 = 10348 items=["Volts"=10348, "From Custom Scale"=10065] ("units")
        n719 = local read "RUN Identifier"() -> (w1709:string)
        n720 = Concatenate Strings(w1709, "_AO" ("string")) -> (w1729:string)
        n721 = Concatenate Strings(w1709, "_", "USB_AOUT.csv" ("string")) -> (w1721:string)
        n722 = Array To Cluster(array="AOUT Labels") -> (cluster=w1707:T29)
        n723 = Unbundle By Name(w1707) -> ("AOUT Labels[0]"=w1706:string, "AOUT Labels[1]"=w1704:string)
        n724 = Build Path(base path=w1720, name or relative path=w1721) -> (appended path=w1717:path)
        n725 = Concatenate Strings(w1706, w1703) -> (w1705:string)
        n726 = Concatenate Strings(w1704, w1703) -> (w1702:string)
        n727 = Open/Create/Replace File(file path (use dialog)=w1717, operation (0:open)=T25."open or create") -> (refnum out=w1715:refnum<file>)  [unwired: 4 in, 2 out]
        n728 = Build Array(w1706, w1704, w1705, w1702) -> (w1713:string[])
        n729 = call "FileIntialize.vi"("Error In"=w1710, "Labels"=w1713, "refnum in"=w1715) -> ("Error Out"=w1712:errorcluster, "File Refnum"=→"File Refn USB AO":refnum<file>)  [unwired: 7 in]
        n730 = call <vilib>:"DAQmx Create Task.vi"("new task name"=w1729, "auto cleanup"=FALSE, "error in"=w1712) -> ("task out"=w1728:refnum<k21>, "error out"=w1730:errorcluster)  [unwired: 11 in]
        n731 = Index Array(array="AOUT assignment", index #1=0 ("index"), index #2=1 ("index")) -> (element #1=w1699:tag, element #2=w1697:tag)
        n732 = call-poly <vilib>:"DAQmx Create Virtual Channel.vi"("task in"=w1728, "maximum value"=w1727, "minimum value"=w1726, "output terminal configuration"=w1725, "physical channels"=w1699, "units"=w1724, "error in"=w1730) -> ("task out"=w1732:refnum<k21>, "error out"=w1733:errorcluster)  [unwired: 7 in]
        n733 = call-poly <vilib>:"DAQmx Create Virtual Channel.vi"("task in"=w1732, "maximum value"=w1727, "minimum value"=w1726, "physical channels"=w1697, "error in"=w1733) -> ("task out"=w1735:refnum<k21>, "error out"=w1734:errorcluster)  [unwired: 9 in]
        n734 = call <vilib>:"DAQmx Start Task.vi"("task/channels in"=w1735, "error in"=w1734) -> ("task out"=→"AO task out":refnum<k21>, "error out"=w1711:errorcluster)  [unwired: 12 in]
      }
    }
    "error out (USB6210/6218 AOUT)" <- w1185
    n735 = case shown="True" w1156 {
      frame False {
      }
      frame True {
        n736 = flat-sequence {
          frame #0 {
            n737 = property on="Frontpanel screenshots" class="Bool (strict)"("Val(Sgnl)"=TRUE ("Value (Signaling)")) -> ()  [unwired: 2 in, 2 out]
          }
        }
      }
    }
    n738 = flat-sequence {
      tunnel: w1168 -> [w1337]
      tunnel: w1171 -> [w1338]
      tunnel: w1163 -> [w1590]
      tunnel: w1162 -> [w1589]
      frame #0 {
        n739 = stacked-sequence {
          tunnel: w1338 -> [w1343 w1348 w1353 w1358 w1363 w1368 w1373 w1378 w1383 w1388 w1393 w1398 w1403 w1408 w1413 w1418 w1423 w1428 w1433 w1438 w1443 w1448 w1453 w1458 w1463 w1468 w1473 w1478 w1483 w1488 w1493 w1498 w1503 w1508 w1513 w1518 w1523 w1528 w1533 w1538 w1543 w1548 w1553 w1558 w1563 w1568 w1573 w1578 w1583 w1588]
          tunnel: w1337 -> [w1341 w1346 w1351 w1356 w1361 w1366 w1371 w1376 w1381 w1386 w1391 w1396 w1401 w1406 w1411 w1416 w1421 w1426 w1431 w1436 w1441 w1446 w1451 w1456 w1461 w1466 w1471 w1476 w1481 w1486 w1491 w1496 w1501 w1506 w1511 w1516 w1521 w1526 w1531 w1536 w1541 w1546 w1551 w1556 w1561 w1566 w1571 w1576 w1581 w1586]
          frame #0 {
            n740 = Search 1D Array(1D array=w1343, element=T14."T3He1-1" ("SensorLocations")) -> (index of element=w1340:i32)  [unwired: 1 in]
            n741 = Index Array(array=w1341, index=w1340) -> (element=→"T3He1-1":dbl)
          }
          frame #1 {
            n742 = Search 1D Array(1D array=w1348, element=T14."T3He1-2" ("SensorLocations")) -> (index of element=w1345:i32)  [unwired: 1 in]
            n743 = Index Array(array=w1346, index=w1345) -> (element=→"T3He1-2":dbl)
          }
          frame #2 {
            n744 = Search 1D Array(1D array=w1353, element=T14."T3He1-3" ("SensorLocations")) -> (index of element=w1350:i32)  [unwired: 1 in]
            n745 = Index Array(array=w1351, index=w1350) -> (element=→"T3He1-3":dbl)
          }
          frame #3 {
            n746 = Search 1D Array(1D array=w1358, element=T14."T3He1-4" ("SensorLocations")) -> (index of element=w1355:i32)  [unwired: 1 in]
            n747 = Index Array(array=w1356, index=w1355) -> (element=→"T3He1-4":dbl)
          }
          frame #4 {
            n748 = Search 1D Array(1D array=w1363, element=T14."T3He2-1" ("SensorLocations")) -> (index of element=w1360:i32)  [unwired: 1 in]
            n749 = Index Array(array=w1361, index=w1360) -> (element=→"T3He2-1":dbl)
          }
          frame #5 {
            n750 = Search 1D Array(1D array=w1368, element=T14."T3He2-2" ("SensorLocations")) -> (index of element=w1365:i32)  [unwired: 1 in]
            n751 = Index Array(array=w1366, index=w1365) -> (element=→"T3He2-2":dbl)
          }
          frame #6 {
            n752 = Search 1D Array(1D array=w1373, element=T14."T3He3" ("SensorLocations")) -> (index of element=w1370:i32)  [unwired: 1 in]
            n753 = Index Array(array=w1371, index=w1370) -> (element=→"T3He3":dbl)
          }
          frame #7 {
            n754 = Search 1D Array(1D array=w1378, element=T14."T3He4" ("SensorLocations")) -> (index of element=w1375:i32)  [unwired: 1 in]
            n755 = Index Array(array=w1376, index=w1375) -> (element=→"T3He4":dbl)
          }
          frame #8 {
            n756 = Search 1D Array(1D array=w1383, element=T14."T3He5" ("SensorLocations")) -> (index of element=w1380:i32)  [unwired: 1 in]
            n757 = Index Array(array=w1381, index=w1380) -> (element=→"T3He5":dbl)
          }
          frame #9 {
            n758 = Search 1D Array(1D array=w1388, element=T14."T3He6-1" ("SensorLocations")) -> (index of element=w1385:i32)  [unwired: 1 in]
            n759 = Index Array(array=w1386, index=w1385) -> (element=→"T3He6-1" →"T3He6-1/6-2 (HEX1)":dbl)
          }
          frame #10 {
            n760 = Search 1D Array(1D array=w1393, element=T14."T3He6-2" ("SensorLocations")) -> (index of element=w1390:i32)  [unwired: 1 in]
            n761 = Index Array(array=w1391, index=w1390) -> (element=→"T3He6-2" →"T3He6-1/6-2 (3He pot) 2":dbl)
          }
          frame #11 {
            n762 = Search 1D Array(1D array=w1398, element=T14."T3He7-1" ("SensorLocations")) -> (index of element=w1395:i32)  [unwired: 1 in]
            n763 = Index Array(array=w1396, index=w1395) -> (element=→"T3He7-1" →"T3He7-1/7-2 (HEX1)":dbl)
          }
          frame #12 {
            n764 = Search 1D Array(1D array=w1403, element=T14."T3He7-2" ("SensorLocations")) -> (index of element=w1400:i32)  [unwired: 1 in]
            n765 = Index Array(array=w1401, index=w1400) -> (element=→"T3He7-2" →"T3He7-1/6-2 (3He pot) 2":dbl)
          }
          frame #13 {
            n766 = Search 1D Array(1D array=w1408, element=T14."T3He8" ("SensorLocations")) -> (index of element=w1405:i32)  [unwired: 1 in]
            n767 = Index Array(array=w1406, index=w1405) -> (element=→"T3He8":dbl)
          }
          frame #14 {
            n768 = Search 1D Array(1D array=w1413, element=T14."T3He9" ("SensorLocations")) -> (index of element=w1410:i32)  [unwired: 1 in]
            n769 = Index Array(array=w1411, index=w1410) -> (element=→"T3He9":dbl)
          }
          frame #15 {
            n770 = Search 1D Array(1D array=w1418, element=T14."T3He10" ("SensorLocations")) -> (index of element=w1415:i32)  [unwired: 1 in]
            n771 = Index Array(array=w1416, index=w1415) -> (element=→"T3He10":dbl)
          }
          frame #16 {
            n772 = Search 1D Array(1D array=w1423, element=T14."T4He1" ("SensorLocations")) -> (index of element=w1420:i32)  [unwired: 1 in]
            n773 = Index Array(array=w1421, index=w1420) -> (element=→"T4He1" →"T4He1 (4K reservoir )":dbl)
          }
          frame #17 {
            n774 = Search 1D Array(1D array=w1428, element=T14."T4He2-1" ("SensorLocations")) -> (index of element=w1425:i32)  [unwired: 1 in]
            n775 = Index Array(array=w1426, index=w1425) -> (element=→"T4He2-1":dbl)
          }
          frame #18 {
            n776 = Search 1D Array(1D array=w1433, element=T14."T4He2-2" ("SensorLocations")) -> (index of element=w1430:i32)  [unwired: 1 in]
            n777 = Index Array(array=w1431, index=w1430) -> (element=→"T4He2-2":dbl)
          }
          frame #19 {
            n778 = Search 1D Array(1D array=w1438, element=T14."T4He3-1" ("SensorLocations")) -> (index of element=w1435:i32)  [unwired: 1 in]
            n779 = Index Array(array=w1436, index=w1435) -> (element=→"T4He3-1":dbl)
          }
          frame #20 {
            n780 = Search 1D Array(1D array=w1443, element=T14."T4He3-2" ("SensorLocations")) -> (index of element=w1440:i32)  [unwired: 1 in]
            n781 = Index Array(array=w1441, index=w1440) -> (element=→"T4He3-2":dbl)
          }
          frame #21 {
            n782 = Search 1D Array(1D array=w1448, element=T14."T4He3-3" ("SensorLocations")) -> (index of element=w1445:i32)  [unwired: 1 in]
            n783 = Index Array(array=w1446, index=w1445) -> (element=→"T4He3-3":dbl)
          }
          frame #22 {
            n784 = Search 1D Array(1D array=w1453, element=T14."T4He3-4" ("SensorLocations")) -> (index of element=w1450:i32)  [unwired: 1 in]
            n785 = Index Array(array=w1451, index=w1450) -> (element=→"T4He3-4":dbl)
          }
          frame #23 {
            n786 = Search 1D Array(1D array=w1458, element=T14."T4He4" ("SensorLocations")) -> (index of element=w1455:i32)  [unwired: 1 in]
            n787 = Index Array(array=w1456, index=w1455) -> (element=→"T4He4":dbl)
          }
          frame #24 {
            n788 = Search 1D Array(1D array=w1463, element=T14."T4He5" ("SensorLocations")) -> (index of element=w1460:i32)  [unwired: 1 in]
            n789 = Index Array(array=w1461, index=w1460) -> (element=→"T4He5":dbl)
          }
          frame #25 {
            n790 = Search 1D Array(1D array=w1468, element=T14."T4He6" ("SensorLocations")) -> (index of element=w1465:i32)  [unwired: 1 in]
            n791 = Index Array(array=w1466, index=w1465) -> (element=→"T4He6":dbl)
          }
          frame #26 {
            n792 = Search 1D Array(1D array=w1473, element=T14."T4He7" ("SensorLocations")) -> (index of element=w1470:i32)  [unwired: 1 in]
            n793 = Index Array(array=w1471, index=w1470) -> (element=→"T4He7":dbl)
          }
          frame #27 {
            n794 = Search 1D Array(1D array=w1478, element=T14."T4He8" ("SensorLocations")) -> (index of element=w1475:i32)  [unwired: 1 in]
            n795 = Index Array(array=w1476, index=w1475) -> (element=→"T4He8":dbl)
          }
          frame #28 {
            n796 = Search 1D Array(1D array=w1483, element=T14."T4He9" ("SensorLocations")) -> (index of element=w1480:i32)  [unwired: 1 in]
            n797 = Index Array(array=w1481, index=w1480) -> (element=→"T4He9":dbl)
          }
          frame #29 {
            n798 = Search 1D Array(1D array=w1488, element=T14."T4He10" ("SensorLocations")) -> (index of element=w1485:i32)  [unwired: 1 in]
            n799 = Index Array(array=w1486, index=w1485) -> (element=→"T4He10":dbl)
          }
          frame #30 {
            n800 = Search 1D Array(1D array=w1493, element=T14."T1K1" ("SensorLocations")) -> (index of element=w1490:i32)  [unwired: 1 in]
            n801 = Index Array(array=w1491, index=w1490) -> (element=→"T1K1":dbl)
          }
          frame #31 {
            n802 = Search 1D Array(1D array=w1498, element=T14."T1K2" ("SensorLocations")) -> (index of element=w1495:i32)  [unwired: 1 in]
            n803 = Index Array(array=w1496, index=w1495) -> (element=→"T1K2":dbl)
          }
          frame #32 {
            n804 = Search 1D Array(1D array=w1503, element=T14."T1K3-1" ("SensorLocations")) -> (index of element=w1500:i32)  [unwired: 1 in]
            n805 = Index Array(array=w1501, index=w1500) -> (element=→"T1K3-1" →"T1K3-1/3-2 (1K pot)":dbl)
          }
          frame #33 {
            n806 = Search 1D Array(1D array=w1508, element=T14."T1K3-2" ("SensorLocations")) -> (index of element=w1505:i32)  [unwired: 1 in]
            n807 = Index Array(array=w1506, index=w1505) -> (element=→"T1K3-2" →"T1K3-1/3-2 (1K pot) 2":dbl)
          }
          frame #34 {
            n808 = Search 1D Array(1D array=w1513, element=T14."T1K4" ("SensorLocations")) -> (index of element=w1510:i32)  [unwired: 1 in]
            n809 = Index Array(array=w1511, index=w1510) -> (element=→"T1K4":dbl)
          }
          frame #35 {
            n810 = Search 1D Array(1D array=w1518, element=T14."T1K5" ("SensorLocations")) -> (index of element=w1515:i32)  [unwired: 1 in]
            n811 = Index Array(array=w1516, index=w1515) -> (element=→"T1K5":dbl)
          }
          frame #36 {
            n812 = Search 1D Array(1D array=w1523, element=T14."T1K6" ("SensorLocations")) -> (index of element=w1520:i32)  [unwired: 1 in]
            n813 = Index Array(array=w1521, index=w1520) -> (element=→"T1K6":dbl)
          }
          frame #37 {
            n814 = Search 1D Array(1D array=w1528, element=T14."TIP1" ("SensorLocations")) -> (index of element=w1525:i32)  [unwired: 1 in]
            n815 = Index Array(array=w1526, index=w1525) -> (element=→"TIP1":dbl)
          }
          frame #38 {
            n816 = Search 1D Array(1D array=w1533, element=T14."TIP2" ("SensorLocations")) -> (index of element=w1530:i32)  [unwired: 1 in]
            n817 = Index Array(array=w1531, index=w1530) -> (element=→"TIP2":dbl)
          }
          frame #39 {
            n818 = Search 1D Array(1D array=w1538, element=T14."TIP3" ("SensorLocations")) -> (index of element=w1535:i32)  [unwired: 1 in]
            n819 = Index Array(array=w1536, index=w1535) -> (element=→"TIP3":dbl)
          }
          frame #40 {
            n820 = Search 1D Array(1D array=w1543, element=T14."TIP4" ("SensorLocations")) -> (index of element=w1540:i32)  [unwired: 1 in]
            n821 = Index Array(array=w1541, index=w1540) -> (element=→"TIP4":dbl)
          }
          frame #41 {
            n822 = Search 1D Array(1D array=w1548, element=T14."TIP5" ("SensorLocations")) -> (index of element=w1545:i32)  [unwired: 1 in]
            n823 = Index Array(array=w1546, index=w1545) -> (element=→"TIP5":dbl)
          }
          frame #42 {
            n824 = Search 1D Array(1D array=w1553, element=T14."TIP6" ("SensorLocations")) -> (index of element=w1550:i32)  [unwired: 1 in]
            n825 = Index Array(array=w1551, index=w1550) -> (element=→"TIP6":dbl)
          }
          frame #43 {
            n826 = Search 1D Array(1D array=w1558, element=T14."TIP7" ("SensorLocations")) -> (index of element=w1555:i32)  [unwired: 1 in]
            n827 = Index Array(array=w1556, index=w1555) -> (element=→"TIP7":dbl)
          }
          frame #44 {
            n828 = Search 1D Array(1D array=w1563, element=T14."TTH1" ("SensorLocations")) -> (index of element=w1560:i32)  [unwired: 1 in]
            n829 = Index Array(array=w1561, index=w1560) -> (element=→"TTH1":dbl)
          }
          frame #45 {
            n830 = Search 1D Array(1D array=w1568, element=T14."TTH2" ("SensorLocations")) -> (index of element=w1565:i32)  [unwired: 1 in]
            n831 = Index Array(array=w1566, index=w1565) -> (element=→"TTH2":dbl)
          }
          frame #46 {
            n832 = Search 1D Array(1D array=w1573, element=T14."TTH3" ("SensorLocations")) -> (index of element=w1570:i32)  [unwired: 1 in]
            n833 = Index Array(array=w1571, index=w1570) -> (element=→"TTH3":dbl)
          }
          frame #47 {
            n834 = Search 1D Array(1D array=w1578, element=T14."TTH4" ("SensorLocations")) -> (index of element=w1575:i32)  [unwired: 1 in]
            n835 = Index Array(array=w1576, index=w1575) -> (element=→"TTH4":dbl)
          }
          frame #48 {
            n836 = Search 1D Array(1D array=w1583, element="SensorLocation 1") -> (index of element=w1580:i32)  [unwired: 1 in]
            n837 = Index Array(array=w1581, index=w1580) -> (element=→"Temperature 1":dbl)
          }
          frame #49 {
            n838 = Search 1D Array(1D array=w1588, element="SensorLocation 2") -> (index of element=w1585:i32)  [unwired: 1 in]
            n839 = Index Array(array=w1586, index=w1585) -> (element=→"Temperature 2":dbl)
          }
        }
      }
      frame #1 {
        n840 = stacked-sequence {
          tunnel: w1590 -> [w1595 w1600 w1605 w1610 w1615 w1620 w1625 w1630 w1635 w1640 w1645 w1650 w1655 w1660 w1665 w1670 w1675 w1680 w1685]
          tunnel: w1589 -> [w1592 w1598 w1604 w1609 w1614 w1618 w1623 w1628 w1633 w1638 w1643 w1648 w1652 w1657 w1662 w1667 w1672 w1677 _]
          tunnel: w1589 -> [_ _ _ _ _ _ _ _ _ _ _ _ _ _ _ _ _ _ w1683]
          frame #0 {
            n841 = Search 1D Array(1D array=w1595, element="Insulation vacuum") -> (index of element=w1593:i32)  [unwired: 1 in]
            n842 = Index Array(array=w1592, index=w1593) -> (element=→"P_ins" →"P (insulation)":dbl)
          }
          frame #1 {
            n843 = Search 1D Array(1D array=w1600, element="4K reservoir pressure") -> (index of element=w1597:i32)  [unwired: 1 in]
            n844 = Index Array(array=w1598, index=w1597) -> (element=→"P_4Kres" →"P (4K reservoir)":dbl)
          }
          frame #2 {
            n845 = Search 1D Array(1D array=w1605, element="3He inlet pressure") -> (index of element=w1603:i32)  [unwired: 1 in]
            n846 = Index Array(array=w1604, index=w1603) -> (element=→"P_3HeIN" →"P (3He IN)":dbl)
          }
          frame #3 {
            n847 = Search 1D Array(1D array=w1610, element="Shield return press.") -> (index of element=w1608:i32)  [unwired: 1 in]
            n848 = Index Array(array=w1609, index=w1608) -> (element=→"P_SldRTN" →"P (shield return)":dbl)
          }
          frame #4 {
            n849 = Search 1D Array(1D array=w1615, element="3He pot pressure") -> (index of element=w1613:i32)  [unwired: 1 in]
            n850 = Index Array(array=w1614, index=w1613) -> (element=→"P_3Hepot" →"P (3He pot)":dbl)
          }
          frame #5 {
            n851 = Search 1D Array(1D array=w1620, element="1Kpot pressure") -> (index of element=w1617:i32)  [unwired: 1 in]
            n852 = Index Array(array=w1618, index=w1617) -> (element=→"P_1Kpot" →"P (1K pot)":dbl)
          }
          frame #6 {
            n853 = Search 1D Array(1D array=w1625, element="Dewar pressure") -> (index of element=w1622:i32)  [unwired: 1 in]
            n854 = Index Array(array=w1623, index=w1622) -> (element=→"P_Dewar" →"P (Dewar)":dbl)
          }
          frame #7 {
            n855 = Search 1D Array(1D array=w1630, element="HEX7 out pressure") -> (index of element=w1627:i32)  [unwired: 1 in]
            n856 = Index Array(array=w1628, index=w1627) -> (element=→"P_HEX7OUT" →"P (HEX7 out)":dbl)
          }
          frame #8 {
            n857 = Search 1D Array(1D array=w1635, element="Diff pressure HEX4") -> (index of element=w1632:i32)  [unwired: 1 in]
            n858 = Index Array(array=w1633, index=w1632) -> (element=→"DP_HEX4" →"DP HEX4":dbl)
          }
          frame #9 {
            n859 = Search 1D Array(1D array=w1640, element="Diff pressure HEX5") -> (index of element=w1637:i32)  [unwired: 1 in]
            n860 = Index Array(array=w1638, index=w1637) -> (element=→"DP_HEX5" →"DP HEX5":dbl)
          }
          frame #10 {
            n861 = Search 1D Array(1D array=w1645, element="3He pump exhaust flow") -> (index of element=w1642:i32)  [unwired: 1 in]
            n862 = Index Array(array=w1643, index=w1642) -> (element=→"F_1" →"F1 (3He pump exhaust) flow":dbl)
          }
          frame #11 {
            n863 = Search 1D Array(1D array=w1650, element="Shield flow") -> (index of element=w1647:i32)  [unwired: 1 in]
            n864 = Index Array(array=w1648, index=w1647) -> (element=→"F_2" →"F2 (shield flow)":dbl)
          }
          frame #12 {
            n865 = Search 1D Array(1D array=w1655, element="4He return flow from HEX7") -> (index of element=w1653:i32)  [unwired: 1 in]
            n866 = Index Array(array=w1652, index=w1653) -> (element=→"F_3" →"F3 (4He rtn flw via HEX7)":dbl)
          }
          frame #13 {
            n867 = Search 1D Array(1D array=w1660, element="3He incoming flow into HEX7") -> (index of element=w1658:i32)  [unwired: 1 in]
            n868 = Index Array(array=w1657, index=w1658) -> (element=→"F_4" →"F4 (3He in to HEX7)":dbl)
          }
          frame #14 {
            n869 = Search 1D Array(1D array=w1665, element="1Kpot pump exhaust flow") -> (index of element=w1663:i32)  [unwired: 1 in]
            n870 = Index Array(array=w1662, index=w1663) -> (element=→"F_5" →"F5 (1K pump ex.)":dbl)
          }
          frame #15 {
            n871 = Search 1D Array(1D array=w1670, element="4K reservoir level") -> (index of element=w1668:i32)  [unwired: 1 in]
            n872 = Index Array(array=w1667, index=w1668) -> (element=→"L3" →"He level (4K)":dbl)
          }
          frame #16 {
            n873 = Search 1D Array(1D array=w1675, element="1K pot level") -> (index of element=w1673:i32)  [unwired: 1 in]
            n874 = Index Array(array=w1672, index=w1673) -> (element=→"L(1K) (a1)" →"He level (1K)":dbl)
          }
          frame #17 {
            n875 = Search 1D Array(1D array=w1680, element="1K pot (b)") -> (index of element=w1678:i32)  [unwired: 1 in]
            n876 = Index Array(array=w1677, index=w1678) -> (element=→"1K pot(b1)" →"He level (1K) b":dbl)
          }
          frame #18 {
            n877 = case shown="False" TRUE {
              tunnel: w1685 -> [w1690 _]
              tunnel: "3He pot" -> [w1689 w1694]
              tunnel: w1683 -> [w1687 _]
              tunnel: [w1686 w1693] -> w1682
              frame False {
                n878 = Search 1D Array(1D array=w1690, element=w1689) -> (index of element=w1688:i32)  [unwired: 1 in]
                n879 = Index Array(array=w1687, index=w1688) -> (element=w1686:dbl)
              }
              frame True {
                n880 = local read "Labels (HP34401 LM)"() -> (w1695:string[])
                n881 = local read "LastData (HP34401 LM)"() -> (w1691:dbl[])
                n882 = Search 1D Array(1D array=w1695, element=w1694) -> (index of element=w1692:i32)  [unwired: 1 in]
                n883 = Index Array(array=w1691, index=w1692) -> (element=w1693:dbl)
              }
            }
            "3He pot level" <- w1682
            "He level (3He)" <- w1682
          }
        }
      }
    }
    n884 = case shown="True" w1150 {
      tunnel: [w2254 w2266] -> w1210
      tunnel: [w2244 w2265] -> w1218
      tunnel: [w2253 w2264] -> w1211
      tunnel: [w2252 timestamp[] [] ("TimeArray")] -> w1180
      tunnel: [w2251 dbl[][] [] ("DataArray")] -> w1178
      tunnel: w1220 -> [w2250 w2261]
      tunnel: w1219 -> [w2249 w2260]
      tunnel: w1144 -> [w2245 _]
      tunnel: w1147 -> [_ w2255]
      frame False {
        n885 = local read "Record interval"() -> (w2242:i64)
        n886 = call-dynamic "LSI336Data_measure.vi"("LSI336Data in"=w2250, "MeasurementIndex"=w2245, "error in (no error)"=w2249, "save every ... measurements"=w2242) -> ("Active?"=→"Active?\n(LSI336)":bool[], "TimeMeasuremeent"=→"Time of Last Measurement (LSI336)":timestamp, "LSI336Data out"=w2253:refnum<class "LSI336Data.lvclass">, "LastData"=→"Last Data \nLSI336":dbl[], "LastMeasurementConfig"=→"LastMeasurementConfig (336)":T18, "DataArray"=w2251:dbl[][], "Status"=w2244:u16, "TimeArray"=w2252:timestamp[], "error out"=w2254:errorcluster)  [unwired: 3 in]
      }
      frame True {
        n887 = local read "RUN Identifier"() -> (w2256:string)
        n888 = call-dynamic "LSI336Data_initialize.vi"("LSI336Data in"=w2261, "RunIdentifier"=w2256, "InstName"="InstName (LSI336)", "FileFormat"="FileFormat (336)", "LSI336Settings(X, Y)"="LSI336Settings(X,Y)", "error in (no error)"=w2260, "base path"=w2255) -> ("LSI336Data out"=w2264:refnum<class "LSI336Data.lvclass">, "Status"=w2265:T7, "AllLabels"=→"Labels LSI336":string[], "error out"=w2266:errorcluster)  [unwired: 5 in]
      }
    }
    "LSI336 Status" <- w1218
    "error out (LSI336)" <- w1210
    "TimeArray (LSI336)" <- w1180
    "DataArray (336)" <- w1178
    n889 = local read "Labels (HP34401 LM) 2"() -> (w1143:string[])
    n890 = case shown="True" w1150 {
      tunnel: [w2359 w2374] -> w1223
      tunnel: [w2354 w2373] -> w1240
      tunnel: [w2357 w2372] -> w1224
      tunnel: w1144 -> [w2358 _]
      tunnel: w1239 -> [w2348 w2367]
      tunnel: w1238 -> [w2349 w2366]
      tunnel: w1147 -> [_ w2365]
      tunnel: [w2346 timestamp[] [] ("TimeArray")] -> w1237
      tunnel: [w2345 dbl[][] [] ("DataArray")] -> w1236
      frame False {
        w2352 = 24 ("index")
        n891 = local read "Record interval"() -> (w2343:i64)
        n892 = call-dynamic "LSI218Data_measure.vi"("LSI218Data in"=w2349, "MeasurementIndex"=w2358, "error in (no error)"=w2348, "save every ... measurements"=w2343) -> ("TimeMeasuremeent"=→"Time of Last Measurement (LSI218)":timestamp, "Active?"=w2353:bool[], "LSI218Data out"=w2357:refnum<class "LSI218Data.lvclass">, "LastMeasurementConfig"=→"LastMeasurementConfig (218)":T18, "LastData"=w2347:dbl[], "Status"=w2354:u16, "TimeArray"=w2346:timestamp[], "DataArray"=w2345:dbl[][], "error out"=w2359:errorcluster)  [unwired: 3 in]
        "LastData (LSI218)" <- w2347
        n893 = Split 1D Array(array=w2353, index=w2352) -> (first subarray=→"Active?\n (1)":bool[], second subarray=→"Active?\n(2)":bool[])
        n894 = Split 1D Array(array=w2347, index=w2352) -> (first subarray=→"Last Data \nLSI218 (1)":dbl[], second subarray=→"Last Data \nLSI218 (2)":dbl[])
      }
      frame True {
        n895 = local read "RUN Identifier"() -> (w2361:string)
        n896 = call-dynamic "LSI218Data_initialize.vi"("LSI218Settings(A-F)"="LSI218Settings(A-F)", "FileFormat"="FileFormat (218)", "base path"=w2365, "error in (no error)"=w2367, "InstName"="InstName (LSI218)", "RunIdentifier"=w2361, "LSI218Data in"=w2366) -> ("error out"=w2374:errorcluster, "Status"=w2373:T7, "AllLabels"=w2364:string[], "LSI218Data out"=w2372:refnum<class "LSI218Data.lvclass">)  [unwired: 1 in]
        n897 = Split 1D Array(array=w2364, index=24) -> (first subarray=→"Labels LSI218 (1)":string[], second subarray=→"Labels LSI218 (2)":string[])
      }
    }
    "LSI218 Status" <- w1240
    "error out (LSI218)" <- w1223
    n898 = case shown="True" w1150 {
      tunnel: w1149 -> [w1312 w1326]
      tunnel: [w1309 w1325] -> w1148
      tunnel: w1147 -> [_ w1323]
      tunnel: w1146 -> [w1311 w1322]
      tunnel: [w1308 w1319] -> w1145
      tunnel: w1144 -> [w1310 _]
      tunnel: [w1306 dbl[][] [] ("LastDataArray")] -> w1141
      tunnel: [w1305 timestamp[] [] ("LastTimeArray")] -> w1139
      frame False {
        n899 = call-dynamic "LMData_measure.vi"("error in (no error)"=w1311, "MeasurementInterval(>0)"="LM measurement interval (>0)", "MeasurementIndex"=w1310, "LMData in"=w1312) -> ("error out"=w1308:errorcluster, "LastDataArray"=w1306:dbl[][], "LastMeasurement"=→"LastData (HP34401 LM)":dbl[], "LMData out"=w1309:refnum<class "LMData.lvclass">, "LastTimeArray"=w1305:timestamp[])  [unwired: 3 in]
      }
      frame True {
        n900 = local read "RUN Identifier"() -> (w1324:string)
        n901 = call-dynamic "LMData_initialize.vi"("LMData in"=w1326, "VISA resource name"="VISA (HP34401 LM)", "Labels"="Labels (HP34401 LM)", "FileFormat"="FileFormat (HP34401 LM)", "RunIdentifier"=w1324, "InstName"="InstName (HP34401 LM)", "base path"=w1323, "error in (no error)"=w1322, "LevelCalibration (R0, R1, L0, L1)"="LevelCalibration (R0, R1, L0, L1)", "Active?"="Active? (HP34401 LM)") -> ("LMData out"=w1325:refnum<class "LMData.lvclass">, "error out"=w1319:errorcluster)  [unwired: 4 in]
        "Labels (HP34401 LM) 2" <- "Labels (HP34401 LM)"
      }
    }
    "error out (HP34401 LM)" <- w1145
    n902 = Array Size(array=w1143) -> (size(s)=w1142:i32)
    n903 = for {
      N: w1142 -> [_]
      tunnel: w1141 -> [w1266]
      shift-right: [w1253] -> w1135
      shift-left: w1140 -> [w1252]
      shift-right: [w1256] -> w1137
      shift-left: w1140 -> [w1257]
      shift-right: [w1260] -> w1138
      shift-left: w1140 -> [w1261]
      shift-right: [w1255] -> w1136
      shift-left: w1140 -> [w1254]
      tunnel: w1139 -> [w1264]
      i -> [w1265]
      n904 = local read "Plot selecter (HP34401A)\n    1      2     3     4"() -> (w1271:bool[][])
      n905 = Index Array(array=w1266, index (col)=w1265) -> (element=w1263:dbl[])  [unwired: 1 in]
      n906 = Bundle("LastTimeArray"=w1264, "LastDataArray"=w1263) -> (w1262:T30)  [unwired: 1 in]
      n907 = Index Array(array=w1271, index (row) #1=w1265, index (col) #1=0 ("disabled index (col)"), index (row) #2=w1265, index (col) #2=1 ("index (col)"), index (row) #3=w1265, index (col) #3=2 ("index (col)"), index (row) #4=w1265, index (col) #4=3 ("disabled index (col)")) -> (element #1=w1259:bool, element #2=w1258:bool, element #3=w1251:bool, element #4=w1250:bool)
      n908 = stacked-sequence {
        tunnel: w1262 -> [w1273 w1280 w1291 w1299]
        tunnel: w1261 -> [w1275 _ _ _]
        tunnel: [w1274 _ _ _] -> w1260
        tunnel: w1259 -> [w1272 _ _ _]
        tunnel: w1258 -> [_ w1283 _ _]
        tunnel: w1257 -> [_ w1282 _ _]
        tunnel: [_ w1281 _ _] -> w1256
        tunnel: [_ _ w1290 _] -> w1255
        tunnel: w1254 -> [_ _ w1289 _]
        tunnel: [_ _ _ w1298] -> w1253
        tunnel: w1252 -> [_ _ _ w1297]
        tunnel: w1251 -> [_ _ w1288 _]
        tunnel: w1250 -> [_ _ _ w1296]
        frame #0 {
          n909 = case shown="True" w1272 {
            tunnel: w1275 -> [w1276 w1279]
            tunnel: [w1276 w1278] -> w1274
            tunnel: w1273 -> [_ w1277]
            frame False {
            }
            frame True {
              n910 = Build Array (concatenate)(w1279, w1277) -> (w1278:T31)
            }
          }
        }
        frame #1 {
          n911 = case shown="True" w1283 {
            tunnel: [w1284 w1287] -> w1281
            tunnel: w1282 -> [w1284 w1286]
            tunnel: w1280 -> [_ w1285]
            frame False {
            }
            frame True {
              n912 = Build Array (concatenate)(w1286, w1285) -> (w1287:T31)
            }
          }
        }
        frame #2 {
          n913 = case shown="True" w1288 {
            tunnel: [w1292 w1295] -> w1290
            tunnel: w1291 -> [_ w1294]
            tunnel: w1289 -> [w1292 w1293]
            frame False {
            }
            frame True {
              n914 = Build Array (concatenate)(w1293, w1294) -> (w1295:T31)
            }
          }
        }
        frame #3 {
          n915 = case shown="True" w1296 {
            tunnel: [w1300 w1303] -> w1298
            tunnel: w1299 -> [_ w1302]
            tunnel: w1297 -> [w1300 w1301]
            frame False {
            }
            frame True {
              n916 = Build Array (concatenate)(w1301, w1302) -> (w1303:T31)
            }
          }
        }
      }
    }
    n917 = local read "Last Data \n(USB6210)"() -> (w1164:dbl[])
    n918 = local read "Last Data \n(USB6218)"() -> (w1165:dbl[])
    n919 = local read "All Labels (USB6210)"() -> (w1167:string[])
    n920 = local read "All Labels (USB6218)"() -> (w1166:string[])
    n921 = flat-sequence {
      tunnel: w1194 -> [w1754]
      tunnel: [w1749] -> w1193
      tunnel: [w1747] -> w1192
      tunnel: [w1746] -> w1191
      tunnel: [w1745] -> w1190
      tunnel: w1195 -> [w1741]
      frame #0 {
        w1748 = T26 [] ("appended array")
        n922 = Unbundle By Name(w1741) -> ("TimeArray"=w1737:timestamp[], "DataArrayConv"=w1752:dbl[][], "LDArray"=w1751:dbl[])
        "TimeArray (USB6218)" <- w1737
        n923 = Unbundle By Name(w1754) -> ("ReadLeakDet?"=w1753:bool, "LabelLD"=w1756:string, "Labels"=w1750:string[])  [unwired: 1 out]
        n924 = case shown="True" w1753 {
          tunnel: w1756 -> [_ w1764]
          tunnel: w1752 -> [w1758 w1763]
          tunnel: w1751 -> [_ w1762]
          tunnel: [w1758 w1761] -> w1739
          tunnel: w1750 -> [w1757 w1760]
          tunnel: [w1757 w1759] -> w1742
          frame False {
          }
          frame True {
            n925 = Build Array (concatenate)(w1763, w1762) -> (w1761:dbl[][])
            n926 = Build Array (concatenate)(w1760, w1764) -> (w1759:string[])
          }
        }
        "All Labels (USB6218)" <- w1742
        "DataArrayConv (USB6218)" <- w1739
        n927 = Array Size(array=w1737) -> (size(s)=→"TimeArray size (6218)":i32)
        n928 = local read "Plot selecter (USB6218)\n    1      2     3     4"() -> (w1744:bool[][])
        n929 = control-ref of="Plot selecter (USB6218)\n    1      2     3     4"() -> (w1740:refnum<vi>)
        n930 = Array Size(array=w1742) -> (size(s)=w1743:i32)
        n931 = Array Size(array=w1742) -> (size(s)=w1755:i32)
        n932 = Array Size(array=w1739) -> (size(s)=→"DataArraySize (6218)":i32[])
        n933 = property on="Property Node" class="Arr (strict)"(reference=w1740, "Number of Rows"=w1743) -> ()  [unwired: 1 in, 2 out]
        n934 = for {
          N: w1755 -> [_]
          tunnel: w1739 -> [w1785]
          tunnel: w1737 -> [w1786]
          shift-right: [w1780] -> w1747
          shift-left: w1748 -> [w1783]
          shift-right: [w1778] -> w1745
          shift-left: w1748 -> [w1781]
          shift-right: [w1779] -> w1749
          shift-left: w1748 -> [w1777]
          shift-right: [w1776] -> w1746
          shift-left: w1748 -> [w1775]
          tunnel: w1744 -> [w1774]
          i -> [w1769]
          n935 = Index Array(array=w1785, index (col)=w1769) -> (element=w1784:dbl[])  [unwired: 1 in]
          n936 = Index Array(array=w1774, index (row) #1=w1769, index (col) #1=0 ("index (row)"), index (row) #2=w1769, index (col) #2=1 ("index (row)"), index (row) #3=w1769, index (col) #3=2 ("index (row)"), index (row) #4=w1769, index (col) #4=3 ("index (row)")) -> (element #1=w1768:bool, element #2=w1767:bool, element #3=w1766:bool, element #4=w1765:bool)
          n937 = Bundle("TimeArray"=w1786, "DataArrayConv"=w1784) -> (w1782:T32)  [unwired: 1 in]
          n938 = stacked-sequence {
            tunnel: w1768 -> [w1790 _ _ _]
            tunnel: w1783 -> [_ w1798 _ _]
            tunnel: w1766 -> [_ _ w1806 _]
            tunnel: w1782 -> [w1787 w1796 w1805 w1811]
            tunnel: w1765 -> [_ _ _ w1814]
            tunnel: w1781 -> [_ _ _ w1813]
            tunnel: [_ _ _ w1812] -> w1778
            tunnel: [_ w1797 _ _] -> w1780
            tunnel: [w1789 _ _ _] -> w1779
            tunnel: w1777 -> [w1788 _ _ _]
            tunnel: [_ _ w1804 _] -> w1776
            tunnel: w1775 -> [_ _ w1803 _]
            tunnel: w1767 -> [_ w1795 _ _]
            frame #0 {
              n939 = case shown="True" w1790 {
                tunnel: [w1791 w1794] -> w1789
                tunnel: w1787 -> [_ w1793]
                tunnel: w1788 -> [w1791 w1792]
                frame False {
                }
                frame True {
                  n940 = Build Array (concatenate)(w1792, w1793) -> (w1794:T26)
                }
              }
            }
            frame #1 {
              n941 = case shown="True" w1795 {
                tunnel: w1798 -> [w1799 w1802]
                tunnel: [w1799 w1801] -> w1797
                tunnel: w1796 -> [_ w1800]
                frame False {
                }
                frame True {
                  n942 = Build Array (concatenate)(w1802, w1800) -> (w1801:T26)
                }
              }
            }
            frame #2 {
              n943 = case shown="True" w1806 {
                tunnel: [w1807 w1810] -> w1804
                tunnel: w1805 -> [_ w1809]
                tunnel: w1803 -> [w1807 w1808]
                frame False {
                }
                frame True {
                  n944 = Build Array (concatenate)(w1808, w1809) -> (w1810:T26)
                }
              }
            }
            frame #3 {
              n945 = case shown="True" w1814 {
                tunnel: [w1815 w1818] -> w1812
                tunnel: w1811 -> [_ w1817]
                tunnel: w1813 -> [w1815 w1816]
                frame False {
                }
                frame True {
                  n946 = Build Array (concatenate)(w1816, w1817) -> (w1818:T26)
                }
              }
            }
          }
        }
      }
    }
    n947 = case shown="True" "Digital Out ON?" {
      tunnel: w1150 -> [_ w1957]
      tunnel: w1200 -> [w1951 w1956]
      tunnel: [w1951 w1955] -> w1199
      tunnel: w1198 -> [_ w1954]
      tunnel: w1147 -> [_ w1953]
      tunnel: w1181 -> [_ w1952]
      frame False {
      }
      frame True {
        n948 = case shown="True" w1957 {
          tunnel: w1956 -> [w1975 w2161]
          tunnel: [w1975 w2168] -> w1955
          tunnel: w1954 -> [w1976 _]
          tunnel: w1953 -> [_ w2140]
          tunnel: w1952 -> [_ _]
          frame False {
            n949 = flat-sequence {
              frame #0 {
              }
            }
            n950 = case shown="\"USB6218AI\"" "AutoFill Source (P)" {
              tunnel: [w1979 w1980] -> w1961
              frame "USB6210", Default {
                n951 = local read "All Labels (USB6210)"() -> (w1979:string[])
              }
              frame "USB6218AI" {
                n952 = local read "All Labels (USB6218)"() -> (w1980:string[])
              }
            }
            n953 = case shown="\"USB6210\", Default" "AutoFill Source (L)" {
              tunnel: [w1977 w1978] -> w1958
              frame "USB6210", Default {
                n954 = local read "All Labels (USB6210)"() -> (w1977:string[])
              }
              frame "USB6218AI" {
                n955 = local read "All Labels (USB6218)"() -> (w1978:string[])
              }
            }
            n956 = Multiply(x="N for sampling", y=i64 2) -> (x*y=w1970:i64)
            n957 = local read "Cycle #"() -> (w1974:u32)
            n958 = Search 1D Array(1D array=w1961, element="Auto Fll Dewar P. label") -> (index of element=→"Target Index (P)":i32)  [unwired: 1 in]
            n959 = Search 1D Array(1D array=w1958, element="Auto Fll He L. label") -> (index of element=→"Target Index (L)":i32)  [unwired: 1 in]
            n960 = Add(x=w1970, y="Mov. Avg Interval") -> (x+y=w1972:i64)
            n961 = Greater?(x=w1974, y=w1972) -> (0:w1968:bool)
            n962 = And(x=w1968, y="Auto Fill ON?") -> (x .and. y?=w1966:bool)
            n963 = case shown="True" w1966 {
              tunnel: w1976 -> [_ w2014]
              tunnel: "Mov. Avg Interval" -> [_ w2000]
              tunnel: w1970 -> [_ w1987]
              tunnel: "N for sampling" -> [_ w1998]
              frame False {
              }
              frame True {
                n964 = local read "AutoFill Source (L)"() -> (w1981:T8)
                n965 = local read "AutoFill Source (P)"() -> (w1982:T8)
                n966 = case shown="\"USB6218AI\"" w1982 {
                  tunnel: [w2018 w2019] -> w1983
                  frame "USB6210", Default {
                    n967 = local read "DataArrayConv (USB6210)"() -> (w2018:dbl[][])
                  }
                  frame "USB6218AI" {
                    n968 = local read "DataArrayConv (USB6218)"() -> (w2019:dbl[][])
                  }
                }
                n969 = case shown="\"USB6210\", Default" w1981 {
                  tunnel: [w2016 w2017] -> w1985
                  frame "USB6210", Default {
                    n970 = local read "DataArrayConv (USB6210)"() -> (w2016:dbl[][])
                  }
                  frame "USB6218AI" {
                    n971 = local read "DataArrayConv (USB6218)"() -> (w2017:dbl[][])
                  }
                }
                n972 = local read "Pstd"() -> (→"Pstd history":dbl)
                n973 = local read "Lstd"() -> (→"Lstd history":dbl)
                n974 = local read "Target Index (L)"() -> (w1986:i32)
                n975 = local read "Pav (Pa)"() -> (→"Pav history":dbl)
                n976 = local read "Lav (%)"() -> (→"Lav history":dbl)
                n977 = Index Array(array=w1985, index (col)=w1986) -> (element=w1984:dbl[])  [unwired: 1 in]
                n978 = local read "Target Index (P)"() -> (w2015:i32)
                n979 = Unbundle By Name(w2014) -> ("TimeArray"=w2013:timestamp[])
                n980 = Index Array(array=w1983, index (col)=w2015) -> (element=w2002:dbl[])  [unwired: 1 in]
                n981 = Delete From Array(array=w2002, length=w1987) -> (deleted portion=w2010:dbl[])  [unwired: 1 in, 1 out]
                n982 = Delete From Array(array=w1984, length=w1987) -> (deleted portion=w1997:dbl[])  [unwired: 1 in, 1 out]
                n983 = call "MovingAverage.vi"("Moving Average interval"=w2000, "Input Array"=w1984) -> ("M.A. Array"=w1999:dbl[])  [unwired: 9 in]
                n984 = call "MovingAverage.vi"("Moving Average interval"=w2000, "Input Array"=w2002) -> ("M.A. Array"=w2001:dbl[])  [unwired: 9 in]
                n985 = Delete From Array(array=w2001, length=w1987) -> (deleted portion=w2011:dbl[])  [unwired: 1 in, 1 out]
                n986 = Delete From Array(array=w2001, length=w1987) -> (deleted portion=w2007:dbl[])  [unwired: 1 in, 1 out]
                "Last N M.A. Pressures" <- w2007
                n987 = Delete From Array(array=w1999, length=w1987) -> (deleted portion=w1992:dbl[])  [unwired: 1 in, 1 out]
                "Last N M.A. Levels" <- w1992
                n988 = Delete From Array(array=w2013, length=w1987) -> (deleted portion=w1994:timestamp[])  [unwired: 1 in, 1 out]
                n989 = Bundle("TimeArray"=w1994, "DataArrayConv (USB6218)"=w2010) -> (w2009:T33)  [unwired: 1 in]
                n990 = Bundle("TimeArray"=w1994, "M.A. Array"=w2011) -> (w2012:T34)  [unwired: 1 in]
                n991 = Bundle("TimeArray"=w1994, "DataArrayConv (USB6218)"=w1997) -> (w1996:T33)  [unwired: 1 in]
                n992 = Bundle("TimeArray"=w1994, "M.A. Array"=w1992) -> (w1993:T34)  [unwired: 1 in]
                n993 = Array Size(array=w2007) -> (size(s)=w2006:i32)
                n994 = Greater Or Equal?(x=w2006, y=w1998) -> (x >= y?=w2005:bool)
                n995 = Build Array(w2009, w2012) -> (→"Dewar Pressure":T35)
                n996 = Build Array(w1996, w1993) -> (→"He Level":T35)
                n997 = case shown="True" w2005 {
                  tunnel: [w2123 w2128] -> w1991
                  tunnel: w2007 -> [_ w2129]
                  tunnel: w1992 -> [_ w2126]
                  tunnel: [w2123 w2124] -> w1990
                  frame False {
                    w2123 = nan ("mean")
                  }
                  frame True {
                    n998 = call <vilib>:"Std Deviation and Variance.vi"("X"=w2129) -> ("mean"=w2128:dbl, "standard deviation"=w2127:dbl)  [unwired: 1 in, 1 out]
                    n999 = call <vilib>:"Std Deviation and Variance.vi"("X"=w2126) -> ("mean"=w2124:dbl, "standard deviation"=w2125:dbl)  [unwired: 1 in, 1 out]
                    n1000 = local write "Pstd"(w2127) -> ()
                    n1001 = local write "Lstd"(w2125) -> ()
                    n1002 = local write "Pav (Pa)"(w2128) -> ()
                    n1003 = local write "Lav (%)"(w2124) -> ()
                  }
                }
                n1004 = flat-sequence {
                  tunnel: w1991 -> [w2020]
                  tunnel: w1990 -> [w2021]
                  frame #0 {
                    n1005 = flat-sequence {
                      tunnel: w2021 -> [w2023]
                      tunnel: w2020 -> [w2022]
                      tunnel: w2020 -> [w2091]
                      frame #0 {
                        n1006 = stacked-sequence {
                          tunnel: w2023 -> [w2030 w2034 _ _ _ _]
                          tunnel: w2022 -> [_ _ w2048 w2057 w2066 w2075]
                          frame #0 {
                            n1007 = local read "L_low (%)"() -> (w2029:dbl)
                            n1008 = local read "Fill state"() -> (w2027:bool)
                            n1009 = Less?(x=w2030, y=w2029) -> (x < y?=w2026:bool)
                            n1010 = Equal?(x=w2027, y=FALSE) -> (x = y?=w2025:bool)
                            n1011 = And(x=w2026, y=w2025) -> (x .and. y?=w2024:bool)
                            n1012 = case shown="False" w2024 {
                              frame False {
                              }
                              frame True {
                                w2032 = TRUE ("Value (Signaling)")
                                n1013 = property on="Fill state" class="Bool (strict)"("Val(Sgnl)"=w2032) -> ()  [unwired: 2 in, 2 out]
                                n1014 = Not(x=w2032) -> (.not. x?=w2031:bool)
                                n1015 = property on="Fill (false)" class="Bool (strict)"("Val(Sgnl)"=w2031) -> ()  [unwired: 2 in, 2 out]
                              }
                            }
                          }
                          frame #1 {
                            n1016 = local read "L_high (%)"() -> (w2035:dbl)
                            n1017 = local read "Fill state"() -> (w2038:bool)
                            n1018 = Greater?(x=w2034, y=w2035) -> (0:w2033:bool)
                            n1019 = Equal?(x=w2038, y=TRUE) -> (x = y?=w2037:bool)
                            n1020 = And(x=w2033, y=w2037) -> (x .and. y?=w2036:bool)
                            n1021 = case shown="True" w2036 {
                              frame False {
                              }
                              frame True {
                                w2040 = FALSE ("Value (Signaling)")
                                n1022 = property on="Fill state" class="Bool (strict)"("Val(Sgnl)"=w2040) -> ()  [unwired: 2 in, 2 out]
                                n1023 = Not(x=w2040) -> (.not. x?=w2041:bool)
                                n1024 = property on="Fill (false)" class="Bool (strict)"("Val(Sgnl)"=w2041) -> ()  [unwired: 2 in, 2 out]
                              }
                            }
                          }
                          frame #2 {
                            n1025 = local read "P_1_low (Pa)"() -> (w2047:dbl)
                            n1026 = property on="state 1" class="Bool (strict)"() -> ("Value"=w2045:bool)  [unwired: 2 in, 2 out]
                            n1027 = Less?(x=w2048, y=w2047) -> (x < y?=w2044:bool)
                            n1028 = Equal?(x=w2045, y=FALSE) -> (x = y?=w2043:bool)
                            n1029 = And(x=w2043, y=w2044) -> (x .and. y?=w2042:bool)
                            n1030 = case shown="True" w2042 {
                              frame False {
                              }
                              frame True {
                                w2050 = TRUE ("Value (Signaling)")
                                n1031 = property on="state 1" class="Bool (strict)"("Val(Sgnl)"=w2050) -> ()  [unwired: 2 in, 2 out]
                                n1032 = Not(x=w2050) -> (.not. x?=w2049:bool)
                                n1033 = property on="state 1 (false)" class="Bool (strict)"("Val(Sgnl)"=w2049) -> ()  [unwired: 2 in, 2 out]
                              }
                            }
                          }
                          frame #3 {
                            n1034 = local read "P_1_high (Pa)"() -> (w2056:dbl)
                            n1035 = property on="state 1" class="Bool (strict)"() -> ("Value"=w2054:bool)  [unwired: 2 in, 2 out]
                            n1036 = Greater?(x=w2057, y=w2056) -> (0:w2053:bool)
                            n1037 = Equal?(x=w2054, y=TRUE) -> (x = y?=w2052:bool)
                            n1038 = And(x=w2052, y=w2053) -> (x .and. y?=w2051:bool)
                            n1039 = case shown="True" w2051 {
                              frame False {
                              }
                              frame True {
                                w2059 = FALSE ("Value (Signaling)")
                                n1040 = property on="state 1" class="Bool (strict)"("Val(Sgnl)"=w2059) -> ()  [unwired: 2 in, 2 out]
                                n1041 = Not(x=w2059) -> (.not. x?=w2058:bool)
                                n1042 = property on="state 1 (false)" class="Bool (strict)"("Val(Sgnl)"=w2058) -> ()  [unwired: 2 in, 2 out]
                              }
                            }
                          }
                          frame #4 {
                            n1043 = local read "P_2_low (Pa)"() -> (w2065:dbl)
                            n1044 = property on="state 2" class="Bool (strict)"() -> ("Value"=w2060:bool)  [unwired: 2 in, 2 out]
                            n1045 = Less?(x=w2066, y=w2065) -> (x < y?=w2063:bool)
                            n1046 = Equal?(x=w2060, y=FALSE) -> (x = y?=w2062:bool)
                            n1047 = And(x=w2062, y=w2063) -> (x .and. y?=w2061:bool)
                            n1048 = case shown="True" w2061 {
                              frame False {
                              }
                              frame True {
                                w2067 = TRUE ("Value (Signaling)")
                                n1049 = property on="state 2" class="Bool (strict)"("Val(Sgnl)"=w2067) -> ()  [unwired: 2 in, 2 out]
                                n1050 = Not(x=w2067) -> (.not. x?=w2068:bool)
                                n1051 = property on="state 2 (false)" class="Bool (strict)"("Val(Sgnl)"=w2068) -> ()  [unwired: 2 in, 2 out]
                              }
                            }
                          }
                          frame #5 {
                            n1052 = local read "P_2_high (Pa)"() -> (w2074:dbl)
                            n1053 = property on="state 2" class="Bool (strict)"() -> ("Value"=w2069:bool)  [unwired: 2 in, 2 out]
                            n1054 = Greater?(x=w2075, y=w2074) -> (0:w2072:bool)
                            n1055 = Equal?(x=w2069, y=TRUE) -> (x = y?=w2071:bool)
                            n1056 = And(x=w2071, y=w2072) -> (x .and. y?=w2070:bool)
                            n1057 = case shown="True" w2070 {
                              frame False {
                              }
                              frame True {
                                w2076 = FALSE ("Value (Signaling)")
                                n1058 = property on="state 2" class="Bool (strict)"("Val(Sgnl)"=w2076) -> ()  [unwired: 2 in, 2 out]
                                n1059 = Not(x=w2076) -> (.not. x?=w2077:bool)
                                n1060 = property on="state 2 (false)" class="Bool (strict)"("Val(Sgnl)"=w2077) -> ()  [unwired: 2 in, 2 out]
                              }
                            }
                          }
                        }
                      }
                      frame #1 {
                        n1061 = property on="Fill state" class="Bool (strict)"() -> ("Value"=w2078:bool)  [unwired: 2 in, 2 out]
                        n1062 = case shown="True" w2078 {
                          frame False {
                            n1063 = property on="V1 (N.O.)" class="Bool (strict)"("Val(Sgnl)"=TRUE ("V1 (N.O.)")) -> ()  [unwired: 2 in, 2 out]
                            n1064 = property on="V2 (N.C.)" class="Bool (strict)"("Val(Sgnl)"=FALSE ("Value (Signaling)")) -> ()  [unwired: 2 in, 2 out]
                          }
                          frame True {
                            n1065 = property on="state 1" class="Bool (strict)"() -> ("Value"=w2082:bool)  [unwired: 2 in, 2 out]
                            n1066 = property on="state 2" class="Bool (strict)"() -> ("Value"=w2081:bool)  [unwired: 2 in, 2 out]
                            n1067 = case shown="True" w2082 {
                              frame False {
                                n1068 = property on="V1 (N.O.)" class="Bool (strict)"("Val(Sgnl)"=TRUE ("Value (Signaling)")) -> ()  [unwired: 2 in, 2 out]
                                n1069 = local write "Status V1 CTRL"(enum16{"Pressurize", "Release"}."Release" ("Status V1 CTRL")) -> ()
                              }
                              frame True {
                                n1070 = property on="V1 (N.O.)" class="Bool (strict)"("Val(Sgnl)"=FALSE ("V1 (N.O.)")) -> ()  [unwired: 2 in, 2 out]
                                n1071 = local write "Status V1 CTRL"(enum16{"Pressurize", "Release"}."Pressurize" ("Status V1 CTRL")) -> ()
                              }
                            }
                            n1072 = case shown="True" w2081 {
                              frame False {
                                n1073 = property on="V2 (N.C.)" class="Bool (strict)"("Val(Sgnl)"=FALSE ("Value (Signaling)")) -> ()  [unwired: 2 in, 2 out]
                                n1074 = local write "Status V2 CTRL"(enum16{"Pressurize", "Release"}."Release" ("Status V2 CTRL")) -> ()
                              }
                              frame True {
                                n1075 = property on="V2 (N.C.)" class="Bool (strict)"("Val(Sgnl)"=TRUE ("Value (Signaling)")) -> ()  [unwired: 2 in, 2 out]
                                n1076 = local write "Status V2 CTRL"(enum16{"Pressurize", "Release"}."Pressurize" ("Status V2 CTRL")) -> ()
                              }
                            }
                          }
                        }
                      }
                      frame #2 {
                        n1077 = Greater?(x=w2091, y="P_safelimit_high (Pa)") -> (0:w2093:bool)
                        n1078 = Less?(x=w2091, y="P_safelimit_low (Pa)") -> (x < y?=w2095:bool)
                        n1079 = Or(x=w2093, y=w2095) -> (x .or. y?=w2096:bool)
                        n1080 = case shown="False" w2096 {
                          frame False {
                          }
                          frame True {
                            w2097 = FALSE ("Value (Signaling)")
                            w2099 = FALSE ("Value (Signaling)")
                            n1081 = property on="V2 (N.C.)" class="Bool (strict)"("Val(Sgnl)"=FALSE ("V1 (N.O.)")) -> ()  [unwired: 2 in, 2 out]
                            n1082 = property on="state 1" class="Bool (strict)"("Val(Sgnl)"=w2097) -> ()  [unwired: 2 in, 2 out]
                            n1083 = property on="V1 (N.O.)" class="Bool (strict)"("Val(Sgnl)"=TRUE ("V1 (N.O.)")) -> ()  [unwired: 2 in, 2 out]
                            n1084 = property on="state 2" class="Bool (strict)"("Val(Sgnl)"=w2099) -> ()  [unwired: 2 in, 2 out]
                            n1085 = Not(x=w2097) -> (.not. x?=w2098:bool)
                            n1086 = Not(x=w2099) -> (.not. x?=w2100:bool)
                            n1087 = property on="state 1 (false)" class="Bool (strict)"("Val(Sgnl)"=w2098) -> ()  [unwired: 2 in, 2 out]
                            n1088 = property on="state 2 (false)" class="Bool (strict)"("Val(Sgnl)"=w2100) -> ()  [unwired: 2 in, 2 out]
                          }
                        }
                      }
                    }
                  }
                  frame #1 {
                    n1089 = property on="V2 (N.C.)" class="Bool (strict)"() -> ("Value"=w2110:bool)  [unwired: 2 in, 2 out]
                    n1090 = property on="V1 (N.O.)" class="Bool (strict)"() -> ("Value"=w2121:bool)  [unwired: 2 in, 2 out]
                    n1091 = local read "P_1_high (Pa)"() -> (w2115:dbl)
                    n1092 = local read "P_2_high (Pa)"() -> (w2113:dbl)
                    n1093 = local read "P_1_low (Pa)"() -> (w2116:dbl)
                    n1094 = local read "P_2_low (Pa)"() -> (w2114:dbl)
                    n1095 = local read "L_high (%)"() -> (w2111:dbl)
                    n1096 = local read "L_low (%)"() -> (w2112:dbl)
                    n1097 = local read "Pav (Pa)"() -> (w2104:dbl)
                    n1098 = local read "Lav (%)"() -> (w2103:dbl)
                    n1099 = Boolean To (0,1)(Boolean=w2110) -> (0, 1=w2109:i16)
                    n1100 = Boolean To (0,1)(Boolean=w2121) -> (0, 1=w2122:i16)
                    n1101 = local read "File Refn DewarCTRL"() -> (w2117:refnum<file>)
                    n1102 = local read "Cycle #"() -> (w2120:u32)
                    n1103 = Build Array(w2104, w2103, w2116, w2115, w2114, w2113, w2112, w2111, w2122, w2109) -> (w2108:dbl[])
                    n1104 = Get Date/Time In Seconds() -> (seconds since 1Jan1904=w2118:timestamp)
                    n1105 = call "FileWrite.vi"("DataArray"=w2108, "Time Stamp"=w2118, "Error In"=errorcluster {"status"=FALSE, "code"=0, "source"=""}, "FileFormat"=string[] ["%4.5e", "%4.2f", "%4.4e", "%4.4e", "%4.4e", "%4.4e", "%4.4e", "%d", "%d"] ("Array"), "Index"=w2120, "refnum in"=w2117) -> ("Error Out"=→"Error Out (Dewar CTRL":errorcluster, "Byte Stream File Refnum"=w2107:refnum<file>)  [unwired: 4 in]
                    n1106 = local write "File Refn DewarCTRL"(w2107) -> ()
                  }
                }
              }
            }
          }
          frame True {
            n1107 = flat-sequence {
              frame #0 {
                w2183 = FALSE ("V1 (N.O.)")
                n1108 = local write "V1 (N.O.)"(TRUE ("V1 (N.O.)")) -> ()
                n1109 = local write "V2 (N.C.)"(FALSE ("V1 (N.O.)")) -> ()
                n1110 = local write "state 2"(w2183) -> ()
                n1111 = local write "state 1"(w2183) -> ()
                n1112 = local write "Fill state"(w2183) -> ()
                n1113 = Not(x=w2183) -> (.not. x?=w2185:bool)
                n1114 = Not(x=w2183) -> (.not. x?=w2184:bool)
                n1115 = local write "state 1 (false)"(w2184) -> ()
                n1116 = local write "state 2 (false)"(w2184) -> ()
                n1117 = local write "Fill (false)"(w2185) -> ()
              }
            }
            n1118 = local read "RUN Identifier"() -> (w2132:string)
            n1119 = Concatenate Strings(w2132, "_DO" ("new task name")) -> (w2175:string)
            n1120 = Concatenate Strings(w2132, "_") -> (w2143:string)
            n1121 = Concatenate Strings(w2143, "DEWAR.csv" ("string")) -> (w2153:string)
            n1122 = Concatenate Strings(w2143, "USB_DOUT.csv" ("string")) -> (w2155:string)
            n1123 = Build Path(base path=w2140, name or relative path=w2153) -> (appended path=w2152:path)
            n1124 = Build Path(base path=w2140, name or relative path=w2155) -> (appended path=w2166:path)
            n1125 = Open/Create/Replace File(file path (use dialog)=w2166, error in=w2161, operation (0:open)=T25."open or create") -> (refnum out=w2164:refnum<file>, error out=w2160:errorcluster)  [unwired: 3 in, 1 out]
            n1126 = call "FileIntialize.vi"("Error In"=w2160, "Labels"="DOUT6218 Labels", "refnum in"=w2164) -> ("Error Out"=w2149:errorcluster, "File Refnum"=→"File Refn USB DO":refnum<file>)  [unwired: 7 in]
            n1127 = Open/Create/Replace File(file path (use dialog)=w2152, error in=w2149, operation (0:open)=T25."open or create") -> (refnum out=w2158:refnum<file>, error out=w2159:errorcluster)  [unwired: 3 in, 1 out]
            n1128 = Concatenate Strings(w2143, "AZDAX.csv" ("string")) -> (w2141:string)
            n1129 = call "FileIntialize.vi"("Error In"=w2159, "Labels"=string[] ["P_av", "L_av", "P_1_low", "P_1_high", "P_2_low", "P_2_high", "L_low", "L_high", "V1(NO)", "V2(NC)"], "refnum in"=w2158) -> ("Error Out"=w2135:errorcluster, "File Refnum"=→"File Refn DewarCTRL":refnum<file>)  [unwired: 7 in]
            n1130 = Build Path(base path=w2140, name or relative path=w2141) -> (appended path=w2137:path)
            n1131 = Array Size(array="DOUT Physical CH") -> (size(s)=w2130:i32)
            n1132 = Open/Create/Replace File(file path (use dialog)=w2137, operation (0:open)=T25."open or create") -> (refnum out=w2138:refnum<file>)  [unwired: 4 in, 2 out]
            n1133 = call "FileIntialize.vi"("Error In"=w2135, "Labels"=string[] ["AZDAX"] ("string"), "refnum in"=w2138) -> ("Error Out"=w2134:errorcluster, "File Refnum"=→"File ref AZD-AX status":refnum<file>)  [unwired: 7 in]
            n1134 = call <vilib>:"DAQmx Create Task.vi"("new task name"=w2175, "auto cleanup"=FALSE, "error in"=w2134) -> ("task out"=w2147:refnum<k21>, "error out"=w2148:errorcluster)  [unwired: 11 in]
            n1135 = for {
              N: w2130 -> [_]
              tunnel: "DOUT Physical CH" -> [w2180] mode=indexing
              shift-right: [w2178] -> w2145
              shift-left: w2147 -> [w2179]
              tunnel: [FALSE ("auto cleanup")] -> w2146 mode=indexing
              shift-right: [w2176] -> w2144
              shift-left: w2148 -> [w2182]
              w2181 = 1 items=["one channel for each line", "one channel for all lines"] ("line grouping")
              n1136 = call-poly <vilib>:"DAQmx Create Virtual Channel.vi"("task in"=w2179, "lines"=w2180, "line grouping"=w2181, "error in"=w2182) -> ("task out"=w2178:refnum<k21>, "error out"=w2176:errorcluster)  [unwired: 10 in]
            }
            n1137 = call <vilib>:"DAQmx Start Task.vi"("task/channels in"=w2145, "error in"=w2144) -> ("task out"=w2171:refnum<k21>, "error out"=w2169:errorcluster)  [unwired: 12 in]
            n1138 = call <vilib>:"DAQmx Write (Digital 1D Bool NChan 1Samp 1Line).vi"("task/channels in"=w2171, "data"=w2146, "timeout"=10.0, "error in"=w2169) -> ("task out"=→"DOUT task out":refnum<k21>, "error out"=w2168:errorcluster)  [unwired: 9 in, 1 out]
          }
        }
      }
    }
    "error out (USB6210/6218 DOUT)" <- w1199
    n1139 = Build Array (concatenate)(w1164, w1165) -> (w1162:dbl[])
    n1140 = Build Array (concatenate)(w1167, w1166) -> (w1163:string[])
    n1141 = flat-sequence {
      tunnel: w1246 -> [w1835]
      tunnel: [w1830] -> w1234
      tunnel: [w1828] -> w1232
      tunnel: [w1827] -> w1229
      tunnel: [w1826] -> w1227
      tunnel: w1198 -> [w1821]
      frame #0 {
        w1829 = T26 [] ("appended array")
        n1142 = Unbundle By Name(w1821) -> ("TimeArray"=w1838:timestamp[], "DataArrayConv"=w1833:dbl[][], "LDArray"=w1832:dbl[])
        n1143 = Unbundle By Name(w1835) -> ("ReadLeakDet?"=w1834:bool, "LabelLD"=w1837:string, "Labels"=w1831:string[])  [unwired: 1 out]
        n1144 = case shown="True" w1834 {
          tunnel: w1837 -> [_ w1846]
          tunnel: w1833 -> [w1840 w1845]
          tunnel: w1832 -> [_ w1844]
          tunnel: [w1840 w1843] -> w1820
          tunnel: w1831 -> [w1839 w1842]
          tunnel: [w1839 w1841] -> w1823
          frame False {
          }
          frame True {
            n1145 = Build Array (concatenate)(w1845, w1844) -> (w1843:dbl[][])
            n1146 = Build Array (concatenate)(w1842, w1846) -> (w1841:string[])
          }
        }
        "All Labels (USB6210)" <- w1823
        "DataArrayConv (USB6210)" <- w1820
        n1147 = control-ref of="Plot selecter (USB6210)\n    1      2     3     4"() -> (w1822:refnum<vi>)
        n1148 = local read "Plot selecter (USB6210)\n    1      2     3     4"() -> (w1825:bool[][])
        n1149 = Array Size(array=w1823) -> (size(s)=w1836:i32)
        n1150 = Array Size(array=w1823) -> (size(s)=w1824:i32)
        n1151 = Array Size(array=w1820) -> (size(s)=→"Data Array sizes (6210)":i32[])
        n1152 = property on="Property Node" class="Arr (strict)"(reference=w1822, "Number of Rows"=w1824) -> ()  [unwired: 1 in, 2 out]
        n1153 = for {
          N: w1836 -> [_]
          tunnel: w1820 -> [w1867]
          tunnel: w1838 -> [w1868]
          shift-right: [w1863] -> w1828
          shift-left: w1829 -> [w1866]
          shift-right: [w1861] -> w1826
          shift-left: w1829 -> [w1864]
          shift-right: [w1862] -> w1830
          shift-left: w1829 -> [w1860]
          shift-right: [w1859] -> w1827
          shift-left: w1829 -> [w1858]
          tunnel: w1825 -> [w1857]
          i -> [w1852]
          n1154 = Index Array(array=w1867, index (col)=w1852) -> (element=w1847:dbl[])  [unwired: 1 in]
          n1155 = Index Array(array=w1857, index (row) #1=w1852, index (col) #1=0 ("index (row)"), index (row) #2=w1852, index (col) #2=1 ("index (row)"), index (row) #3=w1852, index (col) #3=2 ("index (row)"), index (row) #4=w1852, index (col) #4=3 ("index (row)")) -> (element #1=w1851:bool, element #2=w1850:bool, element #3=w1849:bool, element #4=w1848:bool)
          n1156 = Bundle("TimeArray"=w1868, "DataArrayConv"=w1847) -> (w1865:T32)  [unwired: 1 in]
          n1157 = stacked-sequence {
            tunnel: w1851 -> [w1872 _ _ _]
            tunnel: w1866 -> [_ w1880 _ _]
            tunnel: w1849 -> [_ _ w1888 _]
            tunnel: w1865 -> [w1869 w1878 w1887 w1893]
            tunnel: w1848 -> [_ _ _ w1896]
            tunnel: w1864 -> [_ _ _ w1895]
            tunnel: [_ _ _ w1894] -> w1861
            tunnel: [_ w1879 _ _] -> w1863
            tunnel: [w1871 _ _ _] -> w1862
            tunnel: w1860 -> [w1870 _ _ _]
            tunnel: [_ _ w1886 _] -> w1859
            tunnel: w1858 -> [_ _ w1885 _]
            tunnel: w1850 -> [_ w1877 _ _]
            frame #0 {
              n1158 = case shown="True" w1872 {
                tunnel: [w1873 w1876] -> w1871
                tunnel: w1869 -> [_ w1875]
                tunnel: w1870 -> [w1873 w1874]
                frame False {
                }
                frame True {
                  n1159 = Build Array (concatenate)(w1874, w1875) -> (w1876:T26)
                }
              }
            }
            frame #1 {
              n1160 = case shown="True" w1877 {
                tunnel: w1880 -> [w1881 w1884]
                tunnel: [w1881 w1883] -> w1879
                tunnel: w1878 -> [_ w1882]
                frame False {
                }
                frame True {
                  n1161 = Build Array (concatenate)(w1884, w1882) -> (w1883:T26)
                }
              }
            }
            frame #2 {
              n1162 = case shown="True" w1888 {
                tunnel: [w1889 w1892] -> w1886
                tunnel: w1887 -> [_ w1891]
                tunnel: w1885 -> [w1889 w1890]
                frame False {
                }
                frame True {
                  n1163 = Build Array (concatenate)(w1890, w1891) -> (w1892:T26)
                }
              }
            }
            frame #3 {
              n1164 = case shown="True" w1896 {
                tunnel: [w1897 w1900] -> w1894
                tunnel: w1893 -> [_ w1899]
                tunnel: w1895 -> [w1897 w1898]
                frame False {
                }
                frame True {
                  n1165 = Build Array (concatenate)(w1898, w1899) -> (w1900:T26)
                }
              }
            }
          }
        }
      }
    }
    n1166 = local read "Plot selecter LSI218(2)\n    1      2     3     4"() -> (w1221:bool[][])
    n1167 = local read "Plot selecter LSI218(1)\n    1      2     3     4"() -> (w1222:bool[][])
    n1168 = for {
      N: 48 -> [_]
      tunnel: w1237 -> [w2287]
      tunnel: w1236 -> [w2284]
      tunnel: w1222 -> [w2268]
      tunnel: w1221 -> [w2269]
      shift-right: [w2285] -> w1235
      shift-left: w1233 -> [w2286]
      shift-right: [w2280] -> w1230
      shift-left: w1233 -> [w2281]
      shift-right: [w2279] -> w1228
      shift-left: w1233 -> [w2278]
      shift-right: [w2277] -> w1226
      shift-left: w1233 -> [w2276]
      i -> [w2274]
      n1169 = Index Array(array=w2284, index (col)=w2274) -> (element=w2283:dbl[])  [unwired: 1 in]
      n1170 = Less?(x=w2274, y=24) -> (x < y?=w2275:bool)
      n1171 = case shown="True" w2275 {
        tunnel: [w2292 w2310] -> w2273
        tunnel: [w2291 w2309] -> w2272
        tunnel: [w2290 w2307] -> w2271
        tunnel: [w2289 w2306] -> w2270
        tunnel: w2268 -> [_ w2305]
        tunnel: w2269 -> [w2299 _]
        tunnel: w2274 -> [w2294 w2302]
        frame False {
          n1172 = Subtract(x=w2294, y=24) -> (x-y=w2298:i32)
          n1173 = Index Array(array=w2299, index (row) #1=w2298, index (col) #1=0 ("index (row)"), index (row) #2=w2298, index (col) #2=1 ("index (row)"), index (row) #3=w2298, index (col) #3=2 ("index (row)"), index (row) #4=w2298, index (col) #4=3 ("index (row)")) -> (element #1=w2292:bool, element #2=w2291:bool, element #3=w2290:bool, element #4=w2289:bool)
        }
        frame True {
          n1174 = Index Array(array=w2305, index (row) #1=w2302, index (col) #1=0 ("index (row)"), index (row) #2=w2302, index (col) #2=1 ("index (row)"), index (row) #3=w2302, index (col) #3=2 ("index (row)"), index (row) #4=w2302, index (col) #4=3 ("index (row)")) -> (element #1=w2310:bool, element #2=w2309:bool, element #3=w2307:bool, element #4=w2306:bool)
        }
      }
      n1175 = Bundle("TimeArray"=w2287, "DataArray"=w2283) -> (w2282:T36)  [unwired: 1 in]
      n1176 = stacked-sequence {
        tunnel: w2286 -> [w2314 _ _ _]
        tunnel: [w2313 _ _ _] -> w2285
        tunnel: w2282 -> [w2312 w2322 w2330 w2338]
        tunnel: w2281 -> [_ w2321 _ _]
        tunnel: [_ w2320 _ _] -> w2280
        tunnel: [_ _ w2329 _] -> w2279
        tunnel: w2278 -> [_ _ w2328 _]
        tunnel: [_ _ _ w2337] -> w2277
        tunnel: w2276 -> [_ _ _ w2336]
        tunnel: w2273 -> [w2311 _ _ _]
        tunnel: w2272 -> [_ w2319 _ _]
        tunnel: w2271 -> [_ _ w2327 _]
        tunnel: w2270 -> [_ _ _ w2335]
        frame #0 {
          n1177 = case shown="False" w2311 {
            tunnel: w2312 -> [_ w2316]
            tunnel: w2314 -> [w2315 w2318]
            tunnel: [w2315 w2317] -> w2313
            frame False {
            }
            frame True {
              n1178 = Build Array (concatenate)(w2318, w2316) -> (w2317:T4)
            }
          }
        }
        frame #1 {
          n1179 = case shown="True" w2319 {
            tunnel: [w2323 w2326] -> w2320
            tunnel: w2322 -> [_ w2325]
            tunnel: w2321 -> [w2323 w2324]
            frame False {
            }
            frame True {
              n1180 = Build Array (concatenate)(w2324, w2325) -> (w2326:T4)
            }
          }
        }
        frame #2 {
          n1181 = case shown="True" w2327 {
            tunnel: [w2331 w2334] -> w2329
            tunnel: w2330 -> [_ w2333]
            tunnel: w2328 -> [w2331 w2332]
            frame False {
            }
            frame True {
              n1182 = Build Array (concatenate)(w2332, w2333) -> (w2334:T4)
            }
          }
        }
        frame #3 {
          n1183 = case shown="True" w2335 {
            tunnel: [w2339 w2342] -> w2337
            tunnel: w2338 -> [_ w2341]
            tunnel: w2336 -> [w2339 w2340]
            frame False {
            }
            frame True {
              n1184 = Build Array (concatenate)(w2340, w2341) -> (w2342:T4)
            }
          }
        }
      }
    }
    n1185 = local read "Labels LSI336"() -> (w1209:string[])
    n1186 = Array Size(array=w1209) -> (size(s)=w1208:i32)
    n1187 = local read "Plot selecter LSI336 \n     1      2     3     4"() -> (w1217:bool[][])
    n1188 = for {
      N: w1208 -> [_]
      tunnel: w1217 -> [w2200]
      shift-right: [w2194] -> w1215
      shift-left: w1216 -> [w2209]
      shift-right: [w2190] -> w1214
      shift-left: w1216 -> [w2207]
      shift-right: [w2191] -> w1213
      shift-left: w1216 -> [w2206]
      shift-right: [w2189] -> w1212
      shift-left: w1216 -> [w2205]
      tunnel: w1178 -> [w2197]
      tunnel: w1180 -> [w2195]
      i -> [w2198]
      n1189 = Index Array(array=w2197, index (col)=w2198) -> (element=w2196:dbl[])  [unwired: 1 in]
      n1190 = Index Array(array=w2200, index (row) #1=w2198, index (col) #1=0 ("index (row)"), index (row) #2=w2198, index (col) #2=1 ("index (row)"), index (row) #3=w2198, index (col) #3=2 ("index (row)"), index (row) #4=w2198, index (col) #4=3 ("index (row)")) -> (element #1=w2199:bool, element #2=w2193:bool, element #3=w2192:bool, element #4=w2188:bool)
      n1191 = Bundle("TimeArray"=w2195, "DataArray"=w2196) -> (w2208:T36)  [unwired: 1 in]
      n1192 = stacked-sequence {
        tunnel: w2209 -> [w2213 _ _ _]
        tunnel: [w2212 _ _ _] -> w2194
        tunnel: w2208 -> [w2211 w2221 w2229 w2237]
        tunnel: w2207 -> [_ w2220 _ _]
        tunnel: [_ w2219 _ _] -> w2190
        tunnel: [_ _ w2228 _] -> w2191
        tunnel: w2206 -> [_ _ w2227 _]
        tunnel: [_ _ _ w2236] -> w2189
        tunnel: w2205 -> [_ _ _ w2235]
        tunnel: w2199 -> [w2210 _ _ _]
        tunnel: w2193 -> [_ w2218 _ _]
        tunnel: w2192 -> [_ _ w2226 _]
        tunnel: w2188 -> [_ _ _ w2234]
        frame #0 {
          n1193 = case shown="False" w2210 {
            tunnel: w2211 -> [_ w2215]
            tunnel: w2213 -> [w2214 w2217]
            tunnel: [w2214 w2216] -> w2212
            frame False {
            }
            frame True {
              n1194 = Build Array (concatenate)(w2217, w2215) -> (w2216:T4)
            }
          }
        }
        frame #1 {
          n1195 = case shown="True" w2218 {
            tunnel: [w2222 w2225] -> w2219
            tunnel: w2221 -> [_ w2223]
            tunnel: w2220 -> [w2222 w2224]
            frame False {
            }
            frame True {
              n1196 = Build Array (concatenate)(w2224, w2223) -> (w2225:T4)
            }
          }
        }
        frame #2 {
          n1197 = case shown="True" w2226 {
            tunnel: [w2230 w2233] -> w2228
            tunnel: w2229 -> [_ w2231]
            tunnel: w2227 -> [w2230 w2232]
            frame False {
            }
            frame True {
              n1198 = Build Array (concatenate)(w2232, w2231) -> (w2233:T4)
            }
          }
        }
        frame #3 {
          n1199 = case shown="True" w2234 {
            tunnel: [w2238 w2241] -> w2236
            tunnel: w2237 -> [_ w2239]
            tunnel: w2235 -> [w2238 w2240]
            frame False {
            }
            frame True {
              n1200 = Build Array (concatenate)(w2240, w2239) -> (w2241:T4)
            }
          }
        }
      }
    }
    n1201 = Array Size(array=w1180) -> (size(s)=→"TimeArray Size (336)":i32)
    n1202 = Array Size(array=w1178) -> (size(s)=→"DataArray size (336)":i32[])
    n1203 = Build Array (concatenate)(w1234, w1235, w1215, w1193, w1138) -> (→"Graph 1":T26)
    n1204 = Build Array (concatenate)(w1232, w1230, w1214, w1192, w1137) -> (→"Graph 2":T26)
    n1205 = Build Array (concatenate)(w1229, w1228, w1213, w1191, w1136) -> (→"Graph 3":T26)
    n1206 = Build Array (concatenate)(w1227, w1226, w1212, w1190, w1135) -> (→"Graph 4":T26)
    n1207 = Send Notification(notification="Stop Button", notifier=w1155, error in (no error)=w1154) -> (notifier out=w1151:refnum<notifier>, error out=w1152:errorcluster)
    "Cycle #" <- w1144
  }
  n1208 = while {
    tunnel: w5 -> [w2433]
    tunnel: w4 -> [w2432]
    stop <- w2434 stop-if-true
    n1209 = flat-sequence {
      frame #0 {
        n1210 = Divide(x="V_sample", y="I_sample") -> (x/y=w2440:dbl)
        "R_sample" <- w2440
        n1211 = Multiply(x="I_sample", y="V_sample") -> (x*y=→"Q_sample":dbl)
        n1212 = Divide(x="Q_input", y=w2440) -> (x/y=w2439:dbl)
        n1213 = Square Root(x=w2439) -> (sqrt(x)=→"V_input":dbl)
      }
    }
    n1214 = Wait (ms)(milliseconds to wait=u32 214) -> ()  [unwired: 1 out]
    n1215 = property on="CHF power supply selection" class="Bool (strict)"() -> ("Value"=w2427:bool)  [unwired: 2 in, 2 out]
    n1216 = Boolean To (0,1)(Boolean=w2427) -> (0, 1=w2428:i16)
    n1217 = property on="Tab Control 5" class="TabCtl (strict)"("Val(Sgnl)"=w2428) -> ()  [unwired: 2 in, 2 out]
    n1218 = case shown="True" "START heater cycle" {
      frame False {
      }
      frame True {
        n1219 = flat-sequence {
          frame #0 {
            n1220 = while {
              i -> [w2447]
              stop <- w2445 stop-if-true
              n1221 = flat-sequence {
                frame #0 {
                  (unwired) TRUE ("Value (Signaling)")
                }
                frame #1 {
                  n1222 = Multiply(x="t_on", y=1000.0) -> (x*y=w2451:dbl)
                  n1223 = Wait (ms)(milliseconds to wait=w2451) -> ()  [unwired: 1 out]
                }
                frame #2 {
                  (unwired) 0.0 ("Value (Signaling)")
                  (unwired) FALSE ("Value (Signaling)")
                }
                frame #3 {
                  n1224 = Multiply(x="t_off", y=1000.0) -> (x*y=w2456:dbl)
                  n1225 = Wait (ms)(milliseconds to wait=w2456) -> ()  [unwired: 1 out]
                }
              }
              n1226 = case shown="True" "STOP heater cycle" {
                tunnel: [FALSE TRUE] -> w2445
                frame False {
                }
                frame True {
                  n1227 = property on="START heater cycle" class="Bool (strict)"("Val(Sgnl)"=FALSE ("Value (Signaling)")) -> ()  [unwired: 2 in, 2 out]
                }
              }
              "Heat Cycle counter" <- w2447
            }
          }
          frame #1 {
            n1228 = property on="STOP heater cycle" class="Bool (strict)"("Val(Sgnl)"=FALSE ("Value (Signaling)")) -> ()  [unwired: 2 in, 2 out]
          }
        }
      }
    }
    n1229 = case shown="True" "RECORD GRAPH" {
      frame False {
      }
      frame True {
        n1230 = stacked-sequence {
          frame #0 {
            n1231 = Get Date/Time In Seconds() -> (seconds since 1Jan1904=w2475:timestamp)
            n1232 = local read "Base Path"() -> (w2460:path)
            n1233 = local read "RUN Identifier"() -> (w2476:string)
            n1234 = call "LV_UNIXTIME.vi"("current time"=w2475) -> ("date/time string"=w2477:string)  [unwired: 9 in, 1 out]
            n1235 = control-ref of="Graph CHF"() -> (w2466:refnum<vi>)
            n1236 = Concatenate Strings(w2476, "_CHF" ("string"), w2477, "_" ("string"), "CHF Graph Comment") -> (w2462:string)
            n1237 = Concatenate Strings(w2462, ".png" ("string")) -> (w2461:string)
            n1238 = Concatenate Strings(w2462, ".csv" ("string")) -> (w2464:string)
            "CHF file name" <- w2464
            n1239 = Build Path(base path=w2460, name or relative path=w2464) -> (appended path=w2471:path)
            n1240 = invoke class="XYGraph (strict)" method="Get Image"(reference=w2466) -> ("image data"=w2458:T24)  [unwired: 5 in, 5 out]
            n1241 = local read "ƒ¢T_array"() -> (w2468:dbl[])
            n1242 = local read "Q_array"() -> (w2467:dbl[])
            n1243 = Build Path(base path=w2460, name or relative path=w2461) -> (appended path=w2459:path)
            n1244 = Open/Create/Replace File(file path (use dialog)=w2471, operation (0:open)=T25."open or create") -> (refnum out=w2469:refnum<file>)  [unwired: 4 in, 2 out]
            n1245 = for {
              tunnel: w2469 -> [w2481]
              tunnel: w2468 -> [w2479] mode=indexing
              tunnel: w2467 -> [w2478] mode=indexing
              n1246 = Format Into String(format string="%4.4e,%4.4e\\n" ("prompt"), initial string=w2481, w2479, w2478) -> ()  [unwired: 1 in, 2 out]
            }
            n1247 = call <vilib>:"Write PNG File.vi"("image data"=w2458, "path to PNG file"=w2459) -> ()  [unwired: 8 in, 2 out]
          }
          frame #1 {
            n1248 = local write "RECORD GRAPH"(FALSE ("RECORD GRAPH")) -> ()
          }
        }
      }
    }
    n1249 = case shown="True" "START CHF" {
      tunnel: "RecordSettings" -> [_ w2487]
      tunnel: w2427 -> [_ w2486]
      frame False {
      }
      frame True {
        n1250 = stacked-sequence {
          tunnel: [w2492 _ _] -> _
          tunnel: w2487 -> [w2491 w2559 _]
          tunnel: w2486 -> [w2488 w2554 _]
          frame #0 {
            (unwired) T25."open or create" ("operation (0:open)")
            n1251 = case shown="False" w2488 {
              frame False {
                n1252 = property on="Kenwood set V (V)" class="DigNum (strict)"("Val(Sgnl)"="V_start (V)") -> ()  [unwired: 2 in, 2 out]
              }
              frame True {
                n1253 = property on="Kikusui I (mA)" class="DigNum (strict)"("Val(Sgnl)"="I_start (mA)") -> ()  [unwired: 2 in, 2 out]
              }
            }
            n1254 = Get Date/Time In Seconds() -> (seconds since 1Jan1904=w2504:timestamp)
            n1255 = for {
              tunnel: [w2553] -> w2490 mode=indexing
              tunnel: w2491 -> [w2552] mode=indexing
              n1256 = Unbundle By Name(w2552) -> ("SourceLabel"=w2553:string)
            }
            "CHF Data Labels" <- w2490
            n1257 = local read "Base Path"() -> (w2499:path)
            n1258 = local read "RUN Identifier"() -> (w2503:string)
            n1259 = call "LV_UNIXTIME.vi"("current time"=w2504) -> ("date/time string"=w2502:string)  [unwired: 9 in, 1 out]
            n1260 = Concatenate Strings(w2503, "_" ("string"), w2502, "_CHFlog.csv" ("string")) -> (w2498:string)
            "CHF log file name" <- w2498
            n1261 = Build Path(base path=w2499, name or relative path=w2498) -> (appended path=w2497:path)
            n1262 = Open/Create/Replace File(file path (use dialog)=w2497, error in=errorcluster {"status"=FALSE, "code"=0, "source"=""}, operation (0:open)=T25."open or create", access (0:read/write)=enum16{"read/write", "read-only", "write-only"}."read/write") -> (refnum out=w2495:refnum<file>, error out=w2494:errorcluster)  [unwired: 2 in, 1 out]
            n1263 = call "FileIntialize.vi"("Error In"=w2494, "Labels"=w2490, "refnum in"=w2495) -> ("File Refnum"=w2492:refnum<file>)  [unwired: 7 in, 1 out]
            "File Refnum (CHF)" <- w2492
            n1264 = local write "CHF measurement counter"(0 ("CHF counter")) -> ()
            n1265 = stacked-sequence {
              tunnel: w2490 -> [w2509 w2532]
              frame #0 {
                n1266 = Array Size(array=w2509) -> (size(s)=w2517:i32)
                n1267 = control-ref of="Graph CHF log 1"() -> (w2510:refnum<vi>)
                n1268 = property class="XYGraph (strict)"(reference=w2510, error in=errorcluster {"status"=FALSE, "code"=0, "source"=""} ("error in (no error)")) -> (reference out=w2512:refnum<vi>, error out=w2514:errorcluster, "LegNumRows"=w2515:u32)
                n1269 = for {
                  N: w2515 -> [_]
                  shift-right: [w2526] -> w2516
                  shift-left: w2514 -> [w2527]
                  tunnel: w2512 -> [w2525]
                  tunnel: [w2524] -> w2511 mode=indexing
                  i -> [w2529]
                  n1270 = property class="XYGraph (strict)"(reference=w2525, error in=w2527, "Active Plot"=w2529, "Plot.Plot Name"="") -> (reference out=w2524:refnum<vi>, error out=w2526:errorcluster)
                }
                n1271 = for {
                  N: w2517 -> [_]
                  shift-right: [w2521] -> w2508
                  shift-left: w2516 -> [w2522]
                  tunnel: w2511 -> [w2519] mode=indexing
                  tunnel: w2509 -> [w2518] mode=indexing
                  i -> [w2523]
                  n1272 = property class="XYGraph (strict)"(reference=w2519, error in=w2522, "Active Plot"=w2523, "Plot.Plot Name"=w2518, "Plot.Visible?"=TRUE ("Plot.Visible")) -> (error out=w2521:errorcluster)  [unwired: 1 out]
                }
                n1273 = local write "Error out (CHF rec)"(w2508) -> ()
              }
              frame #1 {
                n1274 = Array Size(array=w2532) -> (size(s)=w2539:i32)
                n1275 = control-ref of="Graph CHF log 2"() -> (w2531:refnum<vi>)
                n1276 = property class="XYGraph (strict)"(reference=w2531, error in=errorcluster {"status"=FALSE, "code"=0, "source"=""} ("error in (no error)")) -> (reference out=w2534:refnum<vi>, error out=w2536:errorcluster, "LegNumRows"=w2537:u32)
                n1277 = for {
                  N: w2537 -> [_]
                  shift-right: [w2548] -> w2538
                  shift-left: w2536 -> [w2549]
                  tunnel: w2534 -> [w2547]
                  tunnel: [w2546] -> w2533 mode=indexing
                  i -> [w2551]
                  n1278 = property class="XYGraph (strict)"(reference=w2547, error in=w2549, "Active Plot"=w2551, "Plot.Plot Name"="") -> (reference out=w2546:refnum<vi>, error out=w2548:errorcluster)
                }
                n1279 = for {
                  N: w2539 -> [_]
                  shift-right: [w2543] -> w2530
                  shift-left: w2538 -> [w2544]
                  tunnel: w2533 -> [w2541] mode=indexing
                  tunnel: w2532 -> [w2540] mode=indexing
                  i -> [w2545]
                  n1280 = property class="XYGraph (strict)"(reference=w2541, error in=w2544, "Active Plot"=w2545, "Plot.Plot Name"=w2540, "Plot.Visible?"=TRUE ("Plot.Visible")) -> (error out=w2543:errorcluster)  [unwired: 1 out]
                }
                n1281 = local write "Error out (CHF rec)"(w2530) -> ()
              }
            }
          }
          frame #1 {
            n1282 = case shown="False" w2554 {
              tunnel: ["ƒ¢V / cycle (V)" "ƒ¢I / cycle (mA)"] -> w2558
              tunnel: [w2561 w2573] -> w2557
              frame False {
                n1283 = local read "V_start (V)"() -> (w2560:dbl)
                n1284 = Absolute Value(x="V_end (V)") -> (abs(x)=w2567:dbl)
                n1285 = Absolute Value(x=w2560) -> (abs(x)=w2568:dbl)
                n1286 = Build Array(w2568, w2567) -> (w2566:dbl[])
                n1287 = Array Max & Min(array=w2566) -> (max value=w2565:dbl, min value=w2564:dbl)  [unwired: 2 out]
                n1288 = Subtract(x=w2565, y=w2564) -> (x-y=w2563:dbl)
                n1289 = Quotient & Remainder(x=w2563, y="ƒ¢V / cycle (V)") -> (floor(x/y)=w2561:dbl)  [unwired: 1 out]
              }
              frame True {
                n1290 = local read "I_start (mA)"() -> (w2571:dbl)
                n1291 = Absolute Value(x="I_end (mA)") -> (abs(x)=w2578:dbl)
                n1292 = Absolute Value(x=w2571) -> (abs(x)=w2579:dbl)
                n1293 = Build Array(w2579, w2578) -> (w2577:dbl[])
                n1294 = Array Max & Min(array=w2577) -> (max value=w2576:dbl, min value=w2575:dbl)  [unwired: 2 out]
                n1295 = Subtract(x=w2576, y=w2575) -> (x-y=w2574:dbl)
                n1296 = Quotient & Remainder(x=w2574, y="ƒ¢I / cycle (mA)") -> (floor(x/y)=w2573:dbl)  [unwired: 1 out]
              }
            }
            n1297 = for {
              N: w2557 -> [_]
              tunnel: w2559 -> [w2588]
              shift-right: [w2584] -> _
              shift-left: dbl[][] [] -> [w2586]
              shift-right: [w2583] -> _
              shift-left: timestamp[] [] -> [w2585]
              tunnel: w2558 -> [w2582]
              tunnel: w2554 -> [w2580]
              i -> [w2587]
              n1298 = case shown="False" "STOP CHF" {
                tunnel: w2588 -> [w2605 _]
                tunnel: w2587 -> [w2604 _]
                tunnel: w2586 -> [w2603 w2835]
                tunnel: w2585 -> [w2599 w2834]
                tunnel: [w2596 w2835] -> w2584
                tunnel: [w2595 w2834] -> w2583
                tunnel: w2582 -> [w2589 _]
                tunnel: w2580 -> [w2590 _]
                frame False {
                  n1299 = stacked-sequence {
                    tunnel: w2605 -> [_ _ w2642]
                    tunnel: [_ _ w2633] -> w2594
                    tunnel: w2604 -> [_ _ w2632]
                    tunnel: w2604 -> [w2613 _ _]
                    tunnel: [_ _ w2630] -> w2593
                    tunnel: [_ _ w2629] -> w2598
                    tunnel: [_ _ w2628] -> w2602
                    tunnel: w2603 -> [_ _ w2628]
                    tunnel: [_ _ w2627] -> w2601
                    tunnel: w2599 -> [_ _ w2626]
                    tunnel: [_ _ w2626] -> w2600
                    tunnel: w2589 -> [_ _ _]
                    tunnel: w2590 -> [w2612 _ _]
                    tunnel: w2589 -> [w2611 _ _]
                    frame #0 {
                      n1300 = property on="CHF measurement counter" class="DigNum (strict)"("Val(Sgnl)"=w2613) -> ()  [unwired: 2 in, 2 out]
                      n1301 = case shown="False" w2612 {
                        tunnel: w2611 -> [w2615 w2619]
                        frame False {
                          n1302 = property on="Kenwood set V (V)" class="DigNum (strict)"() -> ("Value"=w2616:dbl)  [unwired: 2 in, 2 out]
                          n1303 = Add(x=w2616, y=w2615) -> (x+y=w2614:dbl)
                          n1304 = property on="Kenwood set V (V)" class="DigNum (strict)"("Val(Sgnl)"=w2614) -> ()  [unwired: 2 in, 2 out]
                        }
                        frame True {
                          n1305 = property on="Kikusui I (mA)" class="DigNum (strict)"() -> ("Value"=w2618:dbl)  [unwired: 2 in, 2 out]
                          n1306 = Add(x=w2618, y=w2619) -> (x+y=w2617:dbl)
                          n1307 = property on="Kikusui I (mA)" class="DigNum (strict)"("Val(Sgnl)"=w2617) -> ()  [unwired: 2 in, 2 out]
                        }
                      }
                    }
                    frame #1 {
                      n1308 = Multiply(x="CHF cycle interval (s) (>1s)", y=1000.0) -> (x*y=w2621:dbl)
                      n1309 = Wait (ms)(milliseconds to wait=w2621) -> ()  [unwired: 1 out]
                    }
                    frame #2 {
                      n1310 = for {
                        tunnel: w2642 -> [w2799] mode=indexing
                        tunnel: [w2797] -> w2629 mode=indexing
                        tunnel: [w2795] -> w2640 mode=indexing
                        n1311 = Unbundle By Name(w2799) -> ("Source"=w2798:T37, "SourceLabel"=w2796:string, "FileFormat"=w2795:string)
                        n1312 = case shown="\"LSI218\"" w2798 {
                          tunnel: [w2800 w2805 w2810 w2816 w2824 w2829] -> w2797
                          tunnel: w2796 -> [w2801 w2807 w2812 w2815 w2825 w2833]
                          frame "USB\n6218\n", Default {
                            n1313 = local read "All Labels (USB6210)"() -> (w2803:string[])
                            n1314 = local read "Last Data \n(USB6210)"() -> (w2804:dbl[])
                            n1315 = Search 1D Array(1D array=w2803, element=w2801) -> (index of element=w2802:i32)  [unwired: 1 in]
                            n1316 = Index Array(array=w2804, index=w2802) -> (element=w2800:dbl)
                          }
                          frame "USB6218AI" {
                            n1317 = local read "All Labels (USB6218)"() -> (w2808:string[])
                            n1318 = local read "Last Data \n(USB6218)"() -> (w2809:dbl[])
                            n1319 = Search 1D Array(1D array=w2808, element=w2807) -> (index of element=w2806:i32)  [unwired: 1 in]
                            n1320 = Index Array(array=w2809, index=w2806) -> (element=w2805:dbl)
                          }
                          frame "USB6218AO" {
                            n1321 = local read "USB 6218 AOUT"() -> (w2814:dbl[])
                            n1322 = local read "AOUT Labels"() -> (w2813:string[])
                            n1323 = Search 1D Array(1D array=w2813, element=w2812) -> (index of element=w2811:i32)  [unwired: 1 in]
                            n1324 = Index Array(array=w2814, index=w2811) -> (element=w2810:dbl)
                          }
                          frame "LSI218" {
                            n1325 = local read "Labels LSI218 (1)"() -> (w2819:string[])
                            n1326 = local read "Labels LSI218 (2)"() -> (w2818:string[])
                            n1327 = local read "Last Data \nLSI218 (1)"() -> (w2822:dbl[])
                            n1328 = local read "Last Data \nLSI218 (2)"() -> (w2821:dbl[])
                            n1329 = Build Array (concatenate)(w2819, w2818) -> (w2817:string[])
                            n1330 = Build Array (concatenate)(w2822, w2821) -> (w2820:dbl[])
                            n1331 = Search 1D Array(1D array=w2817, element=w2815) -> (index of element=w2823:i32)  [unwired: 1 in]
                            n1332 = Index Array(array=w2820, index=w2823) -> (element=w2816:dbl)
                          }
                          frame "LSI336" {
                            n1333 = local read "Last Data \nLSI336"() -> (w2827:dbl[])
                            n1334 = local read "Labels LSI336"() -> (w2828:string[])
                            n1335 = Search 1D Array(1D array=w2828, element=w2825) -> (index of element=w2826:i32)  [unwired: 1 in]
                            n1336 = Index Array(array=w2827, index=w2826) -> (element=w2824:dbl)
                          }
                          frame "DMMs" {
                            n1337 = local read "DMM LastMeasurements"() -> (w2830:dbl[])
                            n1338 = local read "DMMsLabels"() -> (w2832:string[])
                            n1339 = Search 1D Array(1D array=w2832, element=w2833) -> (index of element=w2831:i32)  [unwired: 1 in]
                            n1340 = Index Array(array=w2830, index=w2831) -> (element=w2829:dbl)
                          }
                        }
                      }
                      "CHF last data" <- w2629
                      n1341 = stacked-sequence {
                        tunnel: [w2643 _ _ _] -> w2638
                        tunnel: [_ w2681 _ _] -> w2637
                        tunnel: [_ _ _ w2757] -> w2636
                        tunnel: [_ _ w2719 _] -> w2635
                        frame #0 {
                          n1342 = Unbundle By Name("Data I") -> ("Source"=w2645:T38, "SourceLabel"=w2644:string)
                          n1343 = case shown="\"DMMs\"" w2645 {
                            tunnel: w2644 -> [w2648 w2653 w2658 w2663 w2672 w2677]
                            tunnel: [w2647 w2652 w2657 w2662 w2671 w2676] -> w2643
                            frame "USB6210", Default {
                              n1344 = local read "All Labels (USB6210)"() -> (w2650:string[])
                              n1345 = local read "Last Data \n(USB6210)"() -> (w2649:dbl[])
                              n1346 = Search 1D Array(1D array=w2650, element=w2648) -> (index of element=w2651:i32)  [unwired: 1 in]
                              n1347 = Index Array(array=w2649, index=w2651) -> (element=w2647:dbl)
                            }
                            frame "USB6218AI" {
                              n1348 = local read "All Labels (USB6218)"() -> (w2655:string[])
                              n1349 = local read "Last Data \n(USB6218)"() -> (w2654:dbl[])
                              n1350 = Search 1D Array(1D array=w2655, element=w2653) -> (index of element=w2656:i32)  [unwired: 1 in]
                              n1351 = Index Array(array=w2654, index=w2656) -> (element=w2652:dbl)
                            }
                            frame "USB6218AO" {
                              n1352 = local read "USB 6218 AOUT"() -> (w2659:dbl[])
                              n1353 = local read "AOUT Labels"() -> (w2660:string[])
                              n1354 = Search 1D Array(1D array=w2660, element=w2658) -> (index of element=w2661:i32)  [unwired: 1 in]
                              n1355 = Index Array(array=w2659, index=w2661) -> (element=w2657:dbl)
                            }
                            frame "LSI218" {
                              n1356 = local read "Labels LSI218 (1)"() -> (w2668:string[])
                              n1357 = local read "Labels LSI218 (2)"() -> (w2669:string[])
                              n1358 = local read "Last Data \nLSI218 (1)"() -> (w2665:dbl[])
                              n1359 = local read "Last Data \nLSI218 (2)"() -> (w2666:dbl[])
                              n1360 = Build Array (concatenate)(w2668, w2669) -> (w2670:string[])
                              n1361 = Build Array (concatenate)(w2665, w2666) -> (w2667:dbl[])
                              n1362 = Search 1D Array(1D array=w2670, element=w2663) -> (index of element=w2664:i32)  [unwired: 1 in]
                              n1363 = Index Array(array=w2667, index=w2664) -> (element=w2662:dbl)
                            }
                            frame "LSI336" {
                              n1364 = local read "Last Data \nLSI336"() -> (w2674:dbl[])
                              n1365 = local read "Labels LSI336"() -> (w2673:string[])
                              n1366 = Search 1D Array(1D array=w2673, element=w2672) -> (index of element=w2675:i32)  [unwired: 1 in]
                              n1367 = Index Array(array=w2674, index=w2675) -> (element=w2671:dbl)
                            }
                            frame "DMMs" {
                              n1368 = local read "DMM LastMeasurements"() -> (w2680:dbl[])
                              n1369 = local read "DMMsLabels"() -> (w2678:string[])
                              n1370 = Search 1D Array(1D array=w2678, element=w2677) -> (index of element=w2679:i32)  [unwired: 1 in]
                              n1371 = Index Array(array=w2680, index=w2679) -> (element=w2676:dbl)
                            }
                          }
                          "I" <- w2643
                        }
                        frame #1 {
                          n1372 = Unbundle By Name("Data V") -> ("Source"=w2684:T38, "SourceLabel"=w2683:string)
                          n1373 = case shown="\"LSI218\"" w2684 {
                            tunnel: w2683 -> [w2686 w2691 w2696 w2701 w2710 w2715]
                            tunnel: [w2685 w2690 w2695 w2700 w2709 w2714] -> w2681
                            frame "USB6210", Default {
                              n1374 = local read "All Labels (USB6210)"() -> (w2688:string[])
                              n1375 = local read "Last Data \n(USB6210)"() -> (w2687:dbl[])
                              n1376 = Search 1D Array(1D array=w2688, element=w2686) -> (index of element=w2689:i32)  [unwired: 1 in]
                              n1377 = Index Array(array=w2687, index=w2689) -> (element=w2685:dbl)
                            }
                            frame "USB6218AI" {
                              n1378 = local read "All Labels (USB6218)"() -> (w2693:string[])
                              n1379 = local read "Last Data \n(USB6218)"() -> (w2692:dbl[])
                              n1380 = Search 1D Array(1D array=w2693, element=w2691) -> (index of element=w2694:i32)  [unwired: 1 in]
                              n1381 = Index Array(array=w2692, index=w2694) -> (element=w2690:dbl)
                            }
                            frame "USB6218AO" {
                              n1382 = local read "USB 6218 AOUT"() -> (w2697:dbl[])
                              n1383 = local read "AOUT Labels"() -> (w2698:string[])
                              n1384 = Search 1D Array(1D array=w2698, element=w2696) -> (index of element=w2699:i32)  [unwired: 1 in]
                              n1385 = Index Array(array=w2697, index=w2699) -> (element=w2695:dbl)
                            }
                            frame "LSI218" {
                              n1386 = local read "Labels LSI218 (1)"() -> (w2706:string[])
                              n1387 = local read "Labels LSI218 (2)"() -> (w2707:string[])
                              n1388 = local read "Last Data \nLSI218 (1)"() -> (w2703:dbl[])
                              n1389 = local read "Last Data \nLSI218 (2)"() -> (w2704:dbl[])
                              n1390 = Build Array (concatenate)(w2706, w2707) -> (w2708:string[])
                              n1391 = Build Array (concatenate)(w2703, w2704) -> (w2705:dbl[])
                              n1392 = Search 1D Array(1D array=w2708, element=w2701) -> (index of element=w2702:i32)  [unwired: 1 in]
                              n1393 = Index Array(array=w2705, index=w2702) -> (element=w2700:dbl)
                            }
                            frame "LSI336" {
                              n1394 = local read "Last Data \nLSI336"() -> (w2712:dbl[])
                              n1395 = local read "Labels LSI336"() -> (w2711:string[])
                              n1396 = Search 1D Array(1D array=w2711, element=w2710) -> (index of element=w2713:i32)  [unwired: 1 in]
                              n1397 = Index Array(array=w2712, index=w2713) -> (element=w2709:dbl)
                            }
                            frame "DMMs" {
                              n1398 = local read "DMM LastMeasurements"() -> (w2718:dbl[])
                              n1399 = local read "DMMsLabels"() -> (w2716:string[])
                              n1400 = Search 1D Array(1D array=w2716, element=w2715) -> (index of element=w2717:i32)  [unwired: 1 in]
                              n1401 = Index Array(array=w2718, index=w2717) -> (element=w2714:dbl)
                            }
                          }
                          "V" <- w2681
                        }
                        frame #2 {
                          n1402 = Unbundle By Name("Data T_low") -> ("Source"=w2722:T38, "SourceLabel"=w2721:string)
                          n1403 = case shown="\"DMMs\"" w2722 {
                            tunnel: w2721 -> [w2724 w2729 w2734 w2739 w2748 w2753]
                            tunnel: [w2723 w2728 w2733 w2738 w2747 w2752] -> w2719
                            frame "USB6210", Default {
                              n1404 = local read "All Labels (USB6210)"() -> (w2726:string[])
                              n1405 = local read "Last Data \n(USB6210)"() -> (w2725:dbl[])
                              n1406 = Search 1D Array(1D array=w2726, element=w2724) -> (index of element=w2727:i32)  [unwired: 1 in]
                              n1407 = Index Array(array=w2725, index=w2727) -> (element=w2723:dbl)
                            }
                            frame "USB6218AI" {
                              n1408 = local read "All Labels (USB6218)"() -> (w2731:string[])
                              n1409 = local read "Last Data \n(USB6218)"() -> (w2730:dbl[])
                              n1410 = Search 1D Array(1D array=w2731, element=w2729) -> (index of element=w2732:i32)  [unwired: 1 in]
                              n1411 = Index Array(array=w2730, index=w2732) -> (element=w2728:dbl)
                            }
                            frame "USB6218AO" {
                              n1412 = local read "USB 6218 AOUT"() -> (w2735:dbl[])
                              n1413 = local read "AOUT Labels"() -> (w2736:string[])
                              n1414 = Search 1D Array(1D array=w2736, element=w2734) -> (index of element=w2737:i32)  [unwired: 1 in]
                              n1415 = Index Array(array=w2735, index=w2737) -> (element=w2733:dbl)
                            }
                            frame "LSI218" {
                              n1416 = local read "Labels LSI218 (1)"() -> (w2744:string[])
                              n1417 = local read "Labels LSI218 (2)"() -> (w2745:string[])
                              n1418 = local read "Last Data \nLSI218 (1)"() -> (w2741:dbl[])
                              n1419 = local read "Last Data \nLSI218 (2)"() -> (w2742:dbl[])
                              n1420 = Build Array (concatenate)(w2744, w2745) -> (w2746:string[])
                              n1421 = Build Array (concatenate)(w2741, w2742) -> (w2743:dbl[])
                              n1422 = Search 1D Array(1D array=w2746, element=w2739) -> (index of element=w2740:i32)  [unwired: 1 in]
                              n1423 = Index Array(array=w2743, index=w2740) -> (element=w2738:dbl)
                            }
                            frame "LSI336" {
                              n1424 = local read "Last Data \nLSI336"() -> (w2750:dbl[])
                              n1425 = local read "Labels LSI336"() -> (w2749:string[])
                              n1426 = Search 1D Array(1D array=w2749, element=w2748) -> (index of element=w2751:i32)  [unwired: 1 in]
                              n1427 = Index Array(array=w2750, index=w2751) -> (element=w2747:dbl)
                            }
                            frame "DMMs" {
                              n1428 = local read "DMM LastMeasurements"() -> (w2756:dbl[])
                              n1429 = local read "DMMsLabels"() -> (w2754:string[])
                              n1430 = Search 1D Array(1D array=w2754, element=w2753) -> (index of element=w2755:i32)  [unwired: 1 in]
                              n1431 = Index Array(array=w2756, index=w2755) -> (element=w2752:dbl)
                            }
                          }
                          "T_low" <- w2719
                        }
                        frame #3 {
                          n1432 = Unbundle By Name("Data T_high") -> ("Source"=w2760:T38, "SourceLabel"=w2759:string)
                          n1433 = case shown="\"DMMs\"" w2760 {
                            tunnel: w2759 -> [w2762 w2767 w2772 w2777 w2786 w2791]
                            tunnel: [w2761 w2766 w2771 w2776 w2785 w2790] -> w2757
                            frame "USB6210", Default {
                              n1434 = local read "All Labels (USB6210)"() -> (w2764:string[])
                              n1435 = local read "Last Data \n(USB6210)"() -> (w2763:dbl[])
                              n1436 = Search 1D Array(1D array=w2764, element=w2762) -> (index of element=w2765:i32)  [unwired: 1 in]
                              n1437 = Index Array(array=w2763, index=w2765) -> (element=w2761:dbl)
                            }
                            frame "USB6218AI" {
                              n1438 = local read "All Labels (USB6218)"() -> (w2769:string[])
                              n1439 = local read "Last Data \n(USB6218)"() -> (w2768:dbl[])
                              n1440 = Search 1D Array(1D array=w2769, element=w2767) -> (index of element=w2770:i32)  [unwired: 1 in]
                              n1441 = Index Array(array=w2768, index=w2770) -> (element=w2766:dbl)
                            }
                            frame "USB6218AO" {
                              n1442 = local read "USB 6218 AOUT"() -> (w2773:dbl[])
                              n1443 = local read "AOUT Labels"() -> (w2774:string[])
                              n1444 = Search 1D Array(1D array=w2774, element=w2772) -> (index of element=w2775:i32)  [unwired: 1 in]
                              n1445 = Index Array(array=w2773, index=w2775) -> (element=w2771:dbl)
                            }
                            frame "LSI218" {
                              n1446 = local read "Labels LSI218 (1)"() -> (w2782:string[])
                              n1447 = local read "Labels LSI218 (2)"() -> (w2783:string[])
                              n1448 = local read "Last Data \nLSI218 (1)"() -> (w2779:dbl[])
                              n1449 = local read "Last Data \nLSI218 (2)"() -> (w2780:dbl[])
                              n1450 = Build Array (concatenate)(w2782, w2783) -> (w2784:string[])
                              n1451 = Build Array (concatenate)(w2779, w2780) -> (w2781:dbl[])
                              n1452 = Search 1D Array(1D array=w2784, element=w2777) -> (index of element=w2778:i32)  [unwired: 1 in]
                              n1453 = Index Array(array=w2781, index=w2778) -> (element=w2776:dbl)
                            }
                            frame "LSI336" {
                              n1454 = local read "Last Data \nLSI336"() -> (w2788:dbl[])
                              n1455 = local read "Labels LSI336"() -> (w2787:string[])
                              n1456 = Search 1D Array(1D array=w2787, element=w2786) -> (index of element=w2789:i32)  [unwired: 1 in]
                              n1457 = Index Array(array=w2788, index=w2789) -> (element=w2785:dbl)
                            }
                            frame "DMMs" {
                              n1458 = local read "DMM LastMeasurements"() -> (w2794:dbl[])
                              n1459 = local read "DMMsLabels"() -> (w2792:string[])
                              n1460 = Search 1D Array(1D array=w2792, element=w2791) -> (index of element=w2793:i32)  [unwired: 1 in]
                              n1461 = Index Array(array=w2794, index=w2793) -> (element=w2790:dbl)
                            }
                          }
                          "T_high" <- w2757
                        }
                      }
                      n1462 = local read "File Refnum (CHF)"() -> (w2623:refnum<file>)
                      n1463 = Get Date/Time In Seconds() -> (seconds since 1Jan1904=w2627:timestamp)
                      n1464 = Subtract(x=w2636, y=w2635) -> (x-y=w2631:dbl)
                      "ƒ¢T" <- w2631
                      n1465 = Multiply(x=w2638, y=w2637) -> (x*y=w2634:dbl)
                      "Q" <- w2634
                      n1466 = local read "ƒ¢T_array"() -> (w2625:dbl[])
                      n1467 = local read "Q_array"() -> (w2624:dbl[])
                      n1468 = call "FileWrite.vi"("DataArray"=w2629, "Time Stamp"=w2627, "Error In"=errorcluster {"status"=FALSE, "code"=0, "source"=""}, "FileFormat"=w2640, "Index"=w2632, "refnum in"=w2623) -> ("Error Out"=→"Error out (CHF rec)":errorcluster)  [unwired: 4 in, 1 out]
                      n1469 = Build Array (concatenate)(w2625, w2631) -> (w2630:dbl[])
                      n1470 = Build Array (concatenate)(w2624, w2634) -> (w2633:dbl[])
                    }
                  }
                  n1471 = Build Array (concatenate)(w2602, w2598) -> (w2596:dbl[][])
                  n1472 = Build Array (concatenate)(w2600, w2601) -> (w2595:timestamp[])
                  n1473 = Bundle(w2593, w2594) -> (→"Graph CHF":cluster{dbl[], dbl[]})  [unwired: 1 in]
                  n1474 = local write "ƒ¢T_array"(w2593) -> ()
                  n1475 = local write "Q_array"(w2594) -> ()
                  n1476 = Array Size(array=w2598) -> (size(s)=w2597:i32)
                  n1477 = for {
                    N: w2597 -> [_]
                    tunnel: w2596 -> [w2610]
                    tunnel: w2595 -> [w2608]
                    tunnel: [w2606] -> w2591 mode=indexing
                    i -> [w2609]
                    n1478 = Index Array(array=w2610, index (col)=w2609) -> (element=w2607:dbl[])  [unwired: 1 in]
                    n1479 = Bundle(w2608, w2607) -> (w2606:cluster{timestamp[], dbl[]})  [unwired: 1 in]
                  }
                  "Graph CHF log 2" <- w2591
                  "Graph CHF log 1" <- w2591
                  "Graph CHF log 3" <- w2591
                }
                frame True {
                }
              }
            }
          }
          frame #2 {
            n1480 = local write "CHF measurement counter"(0 ("CHF counter")) -> ()
            n1481 = local write "START CHF"(FALSE ("START CHF")) -> ()
            n1482 = local write "STOP CHF"(FALSE ("STOP CHF")) -> ()
          }
        }
      }
    }
    n1483 = case shown="False" "REFRESH GRAPH" {
      frame False {
      }
      frame True {
        n1484 = stacked-sequence {
          frame #0 {
            w2484 = dbl[] [] ("ƒ¢T_array")
            n1485 = local write "ƒ¢T_array"(w2484) -> ()
            n1486 = local write "Q_array"(w2484) -> ()
            n1487 = Bundle("ƒ¢T_array"=w2484, "ƒ¢T_array"=w2484) -> (w2483:cluster{"ƒ¢T_array":dbl[], "ƒ¢T_array":dbl[]})  [unwired: 1 in]
            n1488 = local write "Graph CHF"(w2483) -> ()
          }
          frame #1 {
            n1489 = local write "REFRESH GRAPH"(FALSE ("REFRESH GRAPH")) -> ()
          }
        }
      }
    }
    n1490 = Get Notifier Status(notifier=w2433, error in (no error)=w2432) -> (current notification=w2434:bool)  [unwired: 4 out]
  }
  n1491 = while {
    shift-right: [w2848] -> w8
    shift-left: refnum<class "DMMsData.lvclass"> refnum ("DMMsData.lvclass") -> [w2847]
    shift-right: [w2846] -> w7
    shift-left: errorcluster {"status"=FALSE, "code"=0, "source"=""} ("error in (no error)") -> [w2839]
    tunnel: w5 -> [w2844]
    tunnel: w4 -> [w2843]
    tunnel: [w2842] -> w11
    i -> [w2845]
    stop <- w2841 stop-if-true
    n1492 = Equal?(x=w2845, y=0) -> (x = y?=w2849:bool)
    n1493 = Wait (ms)(milliseconds to wait="Measurement Interval DMMs (ms)") -> ()  [unwired: 1 out]
    n1494 = case shown="False" "Measure DMMs?" {
      tunnel: w2849 -> [_ w2860]
      tunnel: [w2853 w2858] -> w2848
      tunnel: w2847 -> [w2853 w2857]
      tunnel: w2839 -> [w2852 w2856]
      tunnel: [w2852 w2855] -> w2846
      tunnel: w2845 -> [_ w2854]
      frame False {
      }
      frame True {
        n1495 = Or(x="Initialize (DMMs)", y=w2860) -> (x .or. y?=w2859:bool)
        n1496 = case shown="False" w2859 {
          tunnel: w2857 -> [w2891 w2927]
          tunnel: [w2888 w2926] -> w2858
          tunnel: w2856 -> [w2890 w2923]
          tunnel: [w2889 w2920] -> w2855
          tunnel: w2854 -> [w2887 _]
          frame False {
            n1497 = local read "VariableSources"() -> (w2880:T12)
            n1498 = for {
              tunnel: w2880 -> [w2894] mode=indexing
              tunnel: [w2893] -> w2879 mode=indexing
              tunnel: [w2892] -> w2878 mode=indexing
              n1499 = case shown="\"LSI218\"" w2894 {
                tunnel: [w2896 w2898 w2900 w2901 w2907] -> w2893
                tunnel: [w2895 w2897 w2899 w2902 w2908] -> w2892
                frame "USB6210" {
                  n1500 = local read "All Labels (USB6210)"() -> (w2896:string[])
                  n1501 = local read "Last Data \n(USB6210)"() -> (w2895:dbl[])
                }
                frame "USB6218AI" {
                  n1502 = local read "Last Data \n(USB6218)"() -> (w2897:dbl[])
                  n1503 = local read "All Labels (USB6218)"() -> (w2898:string[])
                }
                frame "USB6218AO" {
                  n1504 = local read "USB 6218 AOUT"() -> (w2899:dbl[])
                  n1505 = local read "AOUT Labels"() -> (w2900:string[])
                }
                frame "LSI218" {
                  n1506 = local read "Last Data \nLSI218 (2)"() -> (w2903:dbl[])
                  n1507 = local read "Last Data \nLSI218 (1)"() -> (w2904:dbl[])
                  n1508 = local read "Labels LSI218 (2)"() -> (w2906:string[])
                  n1509 = local read "Labels LSI218 (1)"() -> (w2905:string[])
                  n1510 = Build Array (concatenate)(w2904, w2903) -> (w2902:dbl[])
                  n1511 = Build Array (concatenate)(w2905, w2906) -> (w2901:string[])
                }
                frame "LSI336" {
                  n1512 = local read "Last Data \nLSI336"() -> (w2908:dbl[])
                  n1513 = local read "Labels LSI336"() -> (w2907:string[])
                }
              }
            }
            n1514 = local read "DMMsConfig (variables)"() -> (w2872:T13)
            n1515 = local read "DMMsConfig"() -> (w2884:T11)
            n1516 = call-dynamic "DMMs_measure.vi"("DMMsData in"=w2891, "Sample #"="Sample #", "MeasurementIndex"=w2887, "SourceDataLabels"=w2879, "error in (no error)"=w2890, "SourceDataArray"=w2878) -> ("TimeArray"=w2886:timestamp[], "DMMsData out"=w2888:refnum<class "DMMsData.lvclass">, "LastData"=w2866:dbl[], "DataArray"=w2883:dbl[][], "DeviceActive?"=→"Active?":bool[], "error out"=w2889:errorcluster)  [unwired: 4 in]
            "DMM LastMeasurements" <- w2866
            n1517 = Array Size(array=w2872) -> (size(s)=w2870:i32)
            n1518 = Array Size(array=w2884) -> (size(s)=w2871:i32)
            n1519 = Add(x=w2871, y=w2870) -> (x+y=w2869:i32)
            n1520 = for {
              N: w2869 -> [_]
              tunnel: w2886 -> [w2911]
              tunnel: w2883 -> [w2915]
              shift-right: [w2909] -> w2868
              shift-left: T4 [] -> [w2910]
              i -> [w2914]
              n1521 = Index Array(array=w2915, index (col)=w2914) -> (element=w2913:dbl[])  [unwired: 1 in]
              n1522 = Bundle("TimeArray"=w2911, "DataArray"=w2913) -> (w2912:T36)  [unwired: 1 in]
              n1523 = Build Array (concatenate)(w2910, w2912) -> (w2909:T4)
            }
            "Graph DMMs 2" <- w2868
            "Graph DMMs 1" <- w2868
            "Graph DMMs 3" <- w2868
            n1524 = Index Array(array=w2866, index #1="index T_2", index #2="index T_ 1") -> (element #1=w2865:dbl, element #2=w2862:dbl)
            n1525 = Index Array(array=w2866, index #1="index V", index #2="index I") -> (element #1=w2875:dbl, element #2=w2874:dbl)
            n1526 = Subtract(x=w2865, y=w2862) -> (x-y=→"ƒ¢T=T_2 -T_1":dbl)
            n1527 = Multiply(x=w2875, y=w2874) -> (x*y=→"Q = I *V":dbl)
          }
          frame True {
            n1528 = local write "Initialize (DMMs)"(FALSE ("Initialize 2")) -> ()
            n1529 = local read "RUN Identifier"() -> (w2919:string)
            n1530 = local read "Base Path"() -> (w2924:path)
            n1531 = call-dynamic "DMMs_initialize.vi"("DMMsConfig (variables)"="DMMsConfig (variables)", "DMMsConfig"="DMMsConfig", "InstName"="InstName DMMs", "error in (no error)"=w2923, "base path"=w2924, "RunIdentifier"=w2919, "DMMsData in"=w2927) -> ("error out"=w2920:errorcluster, "DMMsLabels"=w2921:string[], "FileName"=→"DMMFileName":string, "DMMsData out"=w2926:refnum<class "DMMsData.lvclass">, "VariableSources"=→"VariableSources":T12)
            "DMMsLabels" <- w2921
            n1532 = stacked-sequence {
              tunnel: w2921 -> [w2929 w2952 w2975]
              frame #0 {
                n1533 = Array Size(array=w2929) -> (size(s)=w2938:i32)
                n1534 = control-ref of="Graph DMMs 1"() -> (w2935:refnum<vi>)
                n1535 = property class="XYGraph (strict)"(reference=w2935, error in=errorcluster {"status"=FALSE, "code"=0, "source"=""} ("error in (no error)")) -> (reference out=w2931:refnum<vi>, error out=w2934:errorcluster, "LegNumRows"=w2936:u32)
                n1536 = for {
                  N: w2936 -> [_]
                  shift-right: [w2947] -> w2937
                  shift-left: w2934 -> [w2948]
                  tunnel: w2931 -> [w2946]
                  tunnel: [w2945] -> w2930 mode=indexing
                  i -> [w2950]
                  n1537 = property class="XYGraph (strict)"(reference=w2946, error in=w2948, "Active Plot"=w2950, "Plot.Plot Name"="") -> (reference out=w2945:refnum<vi>, error out=w2947:errorcluster)
                }
                n1538 = for {
                  N: w2938 -> [_]
                  shift-right: [w2942] -> w2932
                  shift-left: w2937 -> [w2943]
                  tunnel: w2930 -> [w2940] mode=indexing
                  tunnel: w2929 -> [w2939] mode=indexing
                  i -> [w2944]
                  n1539 = property class="XYGraph (strict)"(reference=w2940, error in=w2943, "Active Plot"=w2944, "Plot.Plot Name"=w2939, "Plot.Visible?"=TRUE ("Plot.Visible")) -> (error out=w2942:errorcluster)  [unwired: 1 out]
                }
                "error out (DMM graphs)" <- w2932
              }
              frame #1 {
                n1540 = Array Size(array=w2952) -> (size(s)=w2960:i32)
                n1541 = control-ref of="Graph DMMs 2"() -> (w2955:refnum<vi>)
                n1542 = property class="XYGraph (strict)"(reference=w2955, error in=errorcluster {"status"=FALSE, "code"=0, "source"=""} ("error in (no error)")) -> (reference out=w2954:refnum<vi>, error out=w2957:errorcluster, "LegNumRows"=w2958:u32)
                n1543 = for {
                  N: w2958 -> [_]
                  shift-right: [w2969] -> w2959
                  shift-left: w2957 -> [w2970]
                  tunnel: w2954 -> [w2968]
                  tunnel: [w2967] -> w2953 mode=indexing
                  i -> [w2972]
                  n1544 = property class="XYGraph (strict)"(reference=w2968, error in=w2970, "Active Plot"=w2972, "Plot.Plot Name"="") -> (reference out=w2967:refnum<vi>, error out=w2969:errorcluster)
                }
                n1545 = for {
                  N: w2960 -> [_]
                  shift-right: [w2964] -> w2951
                  shift-left: w2959 -> [w2965]
                  tunnel: w2953 -> [w2962] mode=indexing
                  tunnel: w2952 -> [w2961] mode=indexing
                  i -> [w2966]
                  n1546 = property class="XYGraph (strict)"(reference=w2962, error in=w2965, "Active Plot"=w2966, "Plot.Plot Name"=w2961, "Plot.Visible?"=TRUE ("Plot.Visible")) -> (error out=w2964:errorcluster)  [unwired: 1 out]
                }
                n1547 = local write "error out (DMM graphs)"(w2951) -> ()
              }
              frame #2 {
                n1548 = Array Size(array=w2975) -> (size(s)=w2982:i32)
                n1549 = control-ref of="Graph DMMs 3"() -> (w2973:refnum<vi>)
                n1550 = property class="XYGraph (strict)"(reference=w2973, error in=errorcluster {"status"=FALSE, "code"=0, "source"=""} ("error in (no error)")) -> (reference out=w2977:refnum<vi>, error out=w2979:errorcluster, "LegNumRows"=w2980:u32)
                n1551 = for {
                  N: w2980 -> [_]
                  shift-right: [w2991] -> w2981
                  shift-left: w2979 -> [w2992]
                  tunnel: w2977 -> [w2990]
                  tunnel: [w2989] -> w2976 mode=indexing
                  i -> [w2994]
                  n1552 = property class="XYGraph (strict)"(reference=w2990, error in=w2992, "Active Plot"=w2994, "Plot.Plot Name"="") -> (reference out=w2989:refnum<vi>, error out=w2991:errorcluster)
                }
                n1553 = for {
                  N: w2982 -> [_]
                  shift-right: [w2986] -> w2974
                  shift-left: w2981 -> [w2987]
                  tunnel: w2976 -> [w2984] mode=indexing
                  tunnel: w2975 -> [w2983] mode=indexing
                  i -> [w2988]
                  n1554 = property class="XYGraph (strict)"(reference=w2984, error in=w2987, "Active Plot"=w2988, "Plot.Plot Name"=w2983, "Plot.Visible?"=TRUE ("Plot.Visible")) -> (error out=w2986:errorcluster)  [unwired: 1 out]
                }
                n1555 = local write "error out (DMM graphs)"(w2974) -> ()
              }
            }
          }
        }
        "error out (DMMs)" <- w2855
      }
    }
    n1556 = Get Notifier Status(notifier=w2844, error in (no error)=w2843) -> (current notification=w2841:bool, error out=w2842:errorcluster)  [unwired: 3 out]
    "cycle # (DMMs)" <- w2845
  }
  n1557 = call-dynamic "USBData_terminate.vi"("error in (no error)"=w24, "USBData in"=w25) -> ("error out"=w26:errorcluster)  [unwired: 8 in, 1 out]
  n1558 = local write "error out (USB6210)"(w26) -> ()
  n1559 = call-dynamic "DMMs_terminate.vi"("error in (no error)"=w7, "DMMsData in"=w8) -> ("error out"=→"error out (DMMs) 2":errorcluster)  [unwired: 8 in, 1 out]
  n1560 = call-dynamic "USBData_terminate.vi"("error in (no error)"=w39, "USBData in"=w40) -> ("error out"=w41:errorcluster)  [unwired: 8 in, 1 out]
  n1561 = call-dynamic "LSI336Data_terminate.vi"("error in (no error)"=w30, "LSI336Data in"=w31) -> ("error out"=w29:errorcluster)  [unwired: 8 in, 1 out]
  n1562 = Merge Errors(w11, w13) -> (w14:errorcluster)
  n1563 = local write "error out (USB6210)"(w41) -> ()
  n1564 = local write "error out (LSI336)"(w29) -> ()
  n1565 = call "LSI218Data_terminate.vi"("error in (no error)"=w34, "LSI218Data in"=w35) -> ("error out"=w33:errorcluster)  [unwired: 8 in, 1 out]
  n1566 = Release Notifier(notifier=w12, error in (no error)=w14) -> (error out=→"error out (notifier)":errorcluster)  [unwired: 1 in, 2 out]
  n1567 = local write "error out (LSI218)"(w33) -> ()
